vi "Main.vi"() -> ()   [LabVIEW 2024]
uses:
  1. CTL/Brain_Loop_CTL.ctl
  <vilib>/Utility/sysdir.llb/System Directory Type.ctl
  <vilib>/Utility/miscctls.llb/LVPointTypeDef.ctl
panel:
  out "Water_Velocity_2_4":waveform(dbl)(graph)
  out "현재 날짜":string="20"
  out "Averange_Soundspeed_4_5":dbl=7.316387579983064e-08
  out "Averange_Soundspeed_3_5":dbl=2.63750763247972e-07
  out "Averange_Soundspeed_3_4":dbl=7.517605612501092e-08
  out "Averange_Soundspeed_2_5":dbl=3.648976015497772e-07
  out "Averange_Soundspeed_2_4":dbl=2.893826616008644e-07
  out "Averange_Soundspeed_2_3":dbl=7.204154122037209e-07
  out "Averange_Soundspeed_1_5":dbl=6.49097871998956e-08
  out "Averange_Soundspeed_1_4":dbl=1.690561397420498e-07
  out "Averange_Soundspeed_1_3":dbl=1.3254525208911302e-07
  out "Averange_Soundspeed_1_2":dbl=1.8535860648145934e-07
  out "Water_Velocity_4_5":dbl=-0.00010251507677933109
  out "Water_Velocity_3_5":dbl=2.0738097770401804e-05
  out "Water_Velocity_3_4":dbl=-0.00010383942518398899
  out "Water_Velocity_2_5":dbl=-0.01115620755326451
  out "Water_Velocity_2_4":dbl=-0.05349117371632417
  out "Water_Velocity_2_3":dbl=-0.0019132083831803978
  out "Water_Velocity_1_5":dbl=-2.0298889268723733e-05
  out "Water_Velocity_1_4":dbl=0.0007566055432670952
  out "Water_Velocity_1_2":dbl=-0.0005455624048940616
  out "Water_Velocity_1_3":dbl=-0.00019492950449177826
  out "배열":string[](array[string])=["5.120312e-10", "+004.20"]
  out "Averange_Soundspeed_4_5":waveform(dbl)(graph)
  out "Averange_Soundspeed_3_5":waveform(dbl)(graph)
  out "Averange_Soundspeed_3_4":waveform(dbl)(graph)
  out "Averange_Soundspeed_2_5":waveform(dbl)(graph)
  out "Averange_Soundspeed_2_4":waveform(dbl)(graph)
  out "Averange_Soundspeed_2_3":waveform(dbl)(graph)
  out "Averange_Soundspeed_1_5":waveform(dbl)(graph)
  out "Averange_Soundspeed_1_4":waveform(dbl)(graph)
  out "Averange_Soundspeed_1_3":waveform(dbl)(graph)
  out "Averange_Soundspeed_1_2":waveform(dbl)(graph)
  out "Water_Velocity_4_5":waveform(dbl)(graph)
  out "Water_Velocity_3_5":waveform(dbl)(graph)
  out "Water_Velocity_3_4":waveform(dbl)(graph)
  out "Water_Velocity_2_5":waveform(dbl)(graph)
  out "Water_Velocity_2_3":waveform(dbl)(graph)
  out "Water_Velocity_1_5":waveform(dbl)(graph)
  out "Water_Velocity_1_4":waveform(dbl)(graph)
  out "Water_Velocity_1_3":waveform(dbl)(graph)
  out "Water_Velocity_1_2":waveform(dbl)(graph)
  in  "유속 데이터 흐름표_50분":i32(listbox)=-1
  in  "유속 데이터 흐름표_30분":i32(listbox)=-1
  in  "유속 데이터 흐름표_10분":i32(listbox)=-1
  in  "유속 데이터":T1
  in  "데이터 통계":T2
  in  "관리자":T3
  out "디버깅 로그 기록":string="queue2:배터리 전원,소모전류,컨트롤 온도,수온,압력,ROLL,Pitch,2, queue3:(1, 2, 2000, 0, 0, 0, 0, 0, 0, 0, 0, 0, 0, 0, 0, 0, 0, 0, 0, 0, 0, 0, 0, 0, 0, 0, 0, 0, 0, 0, 0, 0, 0, 0, 0, 0, 0, 0, 0, 0, 0, 0, 0, 0, 0, 0, 0, 0, 0, 0, 0, 0, 0, 0, 0, 0, 0, 0, 0, 0, 0, 0, 0, 0, 0, 0, 0, 0, 0, 0, 0, 0, 0, 0, 0, 0, 0, 0, 0, 0, 0, 0, 0, 0, 0, 0, 0, 0, 0, 0, 0, 0, 0, 0, 0, 0, 0, 0, 0, 0, 0, 0, 0, 0, 0, 0, 0, 0, 0, 0, 0, 0, 0, 0, 0, 0, 0, 0, 0, 0, 0, 0, 0, 0, 0, 0, 0, 0, 0, 0, 0, 0, 0, 0, 0, 0, 0, 0, 0, 0, 0, 0, 0, 0, 0, 0, 0, 0, 0, 0, 0, 0, 0, 0, 0, 0, 0, 0, 0, 0, 0, 0, 0, 0, 0, 0, 0, 0, 0, 0, 0, 0, 0, 0, 0, 0, 0, 0, 0, 0, 0, 0, 0, 0, 0, 0, 0, 0, 1, 1, 1, 1, 1, 1, 1, 1, 1, 1, 1, 1, 1, 1, 1, 1, 1, 1, 1, 1, 1, 1, 1, 1, 1, 1, 1, 1, 1, 1, 1, 1, 1, 1, 1, 1, 1, 1, 1, 1, 1, 1, 1, 1, 1, 1, 1, 1, 1, 1, 1, 1, 1, 1, 1, 1, 1, 1, 1, 1, 1, 1, 1, 1, 1, 1, 1, 1, 1, 1, 1, 1, 1, 1, 1, 1, 1, 1, 1, 1, 1, 1, 1, 1, 1, 1, 1, 1, 1, 1, 1, 1, 1, 1, 1, 1, 1, 1, 1, 1, 1, 1, 1, 1, 1, 1, 1, 1, 1, 1, 1, 1, 1, 1, 1, 1, 1, 1, 1, 1, 1, 1, 1, 1, 1, 1, 1, 1, 1, 1, 1, 1, 1, 1, 1, 1, 1, 1, 1, 1, 2, 2, 2, 2, 2, 2, 2, 2, 2, 2, 2, 2, 2, 2, 2, 2, 2, 2, 2, 2, 2, 2, 2, 2, 2, 2, 2, 2, 2, 2, 2, 2, 2, 2, 2, 2, 2, 2, 2, 2, 2, 2, 2, 2, 2, 2, 2, 2, 2, 2, 2, 2, 2, 2, 2, 2, 2, 2, 2, 2, 2, 2, 2, 2, 2, 2, 2, 2, 2, 2, 2, 2, 2, 2, 2, 2, 2, 2, 2, 2, 2, 2, 2, 2, 2, 2, 2, 2, 2, 2, 2, 2, 2, 2, 2, 2, 2, 2, 3, 3, 3, 3, 3, 3, 3, 3, 3, 3, 3, 3, 3, 3, 3, 3, 3, 3, 3, 3, 3, 3, 3, 3, 3, 3, 3, 3, 3, 3, 3, 3, 3, 3, 3, 3, 3, 3, 3, 3, 3, 3, 3, 3, 3, 3, 3, 3, 3, 3, 3, 3, 3, 3, 3, 3, 3, 3, 3, 3, 3, 3, 3, 3, 3, 3, 3, 3, 3, 3, 3, 3, 3, 3, 3, 3, 3, 3, 3, 3, 3, 3, 4, 4, 4, 4, 4, 4, 4, 4, 4, 4, 4, 4, 4, 4, 4, 4, 4, 4, 4, 4, 4, 4, 4, 4, 4, 4, 4, 4, 4, 4, 4, 4, 4, 4, 4, 4, 4, 4, 4, 4, 4, 4, 4, 4, 4, 4, 4, 4, 4, 4, 4, 4, 4, 4, 4, 4, 4, 4, 4, 4, 4, 4, 4, 4, 4, 4, 4, 4, 4, 4, 4, 5, 5, 5, 5, 5, 5, 5, 5, 5, 5, 5, 5, 5, 5, 5, 5, 5, 5, 5, 5, 5, 5, 5, 5, 5, 5, 5, 5, 5, 5, 5, 5, 5, 5, 5, 5, 5, 5, 5, 5, 5, 5, 5, 5, 5, 5, 5, 5, 5, 5, 5, 5, 5, 5, 5, 5, 5, 5, 5, 5, 5, 5, 5, 5, 5, 6, 6, 6, 6, 6, 6, 6, 6, 6, 6, 6, 6, 6, 6, 6, 6, 6, 6, 6, 6, 6, 6, 6, 6, 6, 6, 6, 6, 6, 6, 6, 6, 6, 6, 6, 6, 6, 6, 6, 6, 6, 6, 6, 6, 6, 6, 6, 6, 6, 6, 6, 6, 6, 6, 6, 6, 6, 6, 6, 7, 7, 7, 7, 7, 7, 7, 7, 7, 7, 7, 7, 7, 7, 7, 7, 7, 7, 7, 7, 7, 7, 7, 7, 7, 7, 7, 7, 7, 7, 7, 7, 7, 7, 7, 7, 7, 7, 7, 7, 7, 7, 7, 7, 7, 7, 7, 7, 7, 7, 7, 7, 7, 7, 7, 7, 8, 8, 8, 8, 8, 8, 8, 8, 8, 8, 8, 8, 8, 8, 8, 8, 8, 8, 8, 8, 8, 8, 8, 8, 8, 8, 8, 8, 8, 8, 8, 8, 8, 8, 8, 8, 8, 8, 8, 8, 8, 8, 8, 8, 8, 8, 8, 8, 8, 8, 8, 8, 8, 9, 9, 9, 9, 9, 9, 9, 9, 9, 9, 9, 9, 9, 9, 9, 9, 9, 9, 9, 9, 9, 9, 9, 9, 9, 9, 9, 9, 9, 9, 9, 9, 9, 9, 9, 9, 9, 9, 9, 9, 9, 9, 9, 9, 9, 9, 9, 9, 9, 9, 9, 10, 10, 10, 10, 10, 10, 10, 10, 10, 10, 10, 10, 10, 10, 10, 10, 10, 10, 10, 10, 10, 10, 10, 10, 10, 10, 10, 10, 10, 10, 10, 10, 10, 10, 10, 10, 10, 10, 10, 10, 10, 10, 10, 10, 10, 10, 10, 10, 11, 11, 11, 11, 11, 11, 11, 11, 11, 11, 11, 11, 11, 11, 11, 11, 11, 11, 11, 11, 11, 11, 11, 11, 11, 11, 11, 11, 11, 11, 11, 11, 11, 11, 11, 11, 11, 11, 11, 11, 11, 11, 11, 11, 11, 11, 11, 12, 12, 12, 12, 12, 12, 12, 12, 12, 12, 12, 12, 12, 12, 12, 12, 12, 12, 12, 12, 12, 12, 12, 12, 12, 12, 12, 12, 12, 12, 12, 12, 12, 12, 12, 12, 12, 12, 12, 12, 12, 12, 12, 12, 12, 13, 13, 13, 13, 13, 13, 13, 13, 13, 13, 13, 13, 13, 13, 13, 13, 13, 13, 13, 13, 13, 13, 13, 13, 13, 13, 13, 13, 13, 13, 13, 13, 13, 13, 13, 13, 13, 13, 13, 13, 13, 13, 13, 13, 14, 14, 14, 14, 14, 14, 14, 14, 14, 14, 14, 14, 14, 14, 14, 14, 14, 14, 14, 14, 14, 14, 14, 14, 14, 14, 14, 14, 14, 14, 14, 14, 14, 14, 14, 14, 14, 14, 14, 14, 14, 14, 15, 15, 15, 15, 15, 15, 15, 15, 15, 15, 15, 15, 15, 15, 15, 15, 15, 15, 15, 15, 15, 15, 15, 15, 15, 15, 15, 15, 15, 15, 15, 15, 15, 15, 15, 15, 15, 15, 15, 15, 15, 15, 16, 16, 16, 16, 16, 16, 16, 16, 16, 16, 16, 16, 16, 16, 16, 16, 16, 16, 16, 16, 16, 16, 16, 16, 16, 16, 16, 16, 16, 16, 16, 16, 16, 16, 16, 16, 16, 16, 16, 16, 16, 17, 17, 17, 17, 17, 17, 17, 17, 17, 17, 17, 17, 17, 17, 17, 17, 17, 17, 17, 17, 17, 17, 17, 17, 17, 17, 17, 17, 17, 17, 17, 17, 17, 17, 17, 17, 17, 17, 17, 17, 18, 18, 18, 18, 18, 18, 18, 18, 18, 18, 18, 18, 18, 18, 18, 18, 18, 18, 18, 18, 18, 18, 18, 18, 18, 18, 18, 18, 18, 18, 18, 18, 18, 18, 18, 18, 18, 18, 18, 19, 19, 19, 19, 19, 19, 19, 19, 19, 19, 19, 19, 19, 19, 19, 19, 19, 19, 19, 19, 19, 19, 19, 19, 19, 19, 19, 19, 19, 19, 19, 19, 19, 19, 19, 19, 19, 19, 20, 20, 20, 20, 20, 20, 20, 20, 20, 20, 20, 20, 20, 20, 20, 20, 20, 20, 20, 20, 20, 20, 20, 20, 20, 20, 20, 20, 20, 20, 20, 20, 20, 20, 20, 20, 20, 20, 21, 21, 21, 21, 21, 21, 21, 21, 21, 21, 21, 21, 21, 21, 21, 21, 21, 21, 21, 21, 21, 21, 21, 21, 21, 21, 21, 21, 21, 21, 21, 21, 21, 21, 21, 21, 21, 21, 22, 22, 22, 22, 22, 22, 22, 22, 22, 22, 22, 22, 22, 22, 22, 22, 22, 22, 22, 22, 22, 22, 22, 22, 22, 22, 22, 22, 22, 22, 22, 22, 22, 22, 22, 22, 23, 23, 23, 23, 23, 23, 23, 23, 23, 23, 23, 23, 23, 23, 23, 23, 23, 23, 23, 23, 23, 23, 23, 23, 23, 23, 23, 23, 23, 23, 23, 23, 23, 23, 23, 23, 23, 24, 24, 24, 24, 24, 24, 24, 24, 24, 24, 24, 24, 24, 24, 24, 24, 24, 24, 24, 24, 24, 24, 24, 24, 24, 24, 24, 24, 24, 24, 24, 24, 24, 24, 24, 24, 25, 25, 25, 25, 25, 25, 25, 25, 25, 25, 25, 25, 25, 25, 25, 25, 25, 25, 25, 25, 25, 25, 25, 25, 25, 25, 25, 25, 25, 25, 25, 25, 25, 25, 25, 25, 26, 26, 26, 26, 26, 26, 26, 26, 26, 26, 26, 26, 26, 26, 26, 26, 26, 26, 26, 26, 26, 26, 26, 26, 26, 26, 26, 26, 26, 26, 26, 26, 26, 26, 26, 27, 27, 27, 27, 27, 27, 27, 27, 27, 27, 27, 27, 27, 27, 27, 27, 27, 27, 27, 27, 27, 27, 27, 27, 27, 27, 27, 27, 27, 27, 27, 27, 27, 27, 27, 28, 28, 28, 28, 28, 28, 28, 28, 28, 28, 28, 28, 28, 28, 28, 28, 28, 28, 28, 28, 28, 28, 28, 28, 28, 28, 28, 28, 28, 28, 28, 28, 28, 28, 28, 29, 29, 29, 29, 29, 29, 29, 29, 29, 29, 29, 29, 29, 29, 29, 29, 29, 29, 29, 29, 29, 29, 29, 29, 29, 29, 29, 29, 29, 29, 29, 29, 29, 29, 30, 30, 30, 30, 30, 30, 30, 30, 30, 30, 30, 30, 30, 30, 30, 30, 30, 30, 30, 30, 30, 30, 30, 30, 30, 30, 30, 30, 30, 30, 30, 30, 30, 30, 31, 31, 31, 31, 31, 31, 31, 31, 31, 31, 31, 31, 31, 31, 31, 31, 31, 31, 31, 31, 31, 31, 31, 31, 31, 31, 31, 31, 31, 31, 31, 31, 31, 31, 31, 32, 32, 32, 32, 32, 32, 32, 32, 32, 32, 32, 32, 32, 32, 32, 32, 32, 32, 32, 32, 32, 32, 32, 32, 32, 32, 32, 32, 32, 32, 32, 32, 32, 33, 33, 33, 33, 33, 33, 33, 33, 33, 33, 33, 33, 33, 33, 33, 33, 33, 33, 33, 33, 33, 33, 33, 33, 33, 33, 33, 33, 33, 33, 33, 33, 33, 33, 34, 34, 34, 34, 34, 34, 34, 34, 34, 34, 34, 34, 34, 34, 34, 34, 34, 34, 34, 34, 34, 34, 34, 34, 34, 34, 34, 34, 34, 34, 34, 34, 34, 34, 35, 35, 35, 35, 35, 35, 35, 35, 35, 35, 35, 35, 35, 35, 35, 35, 35, 35, 35, 35, 35, 35, 35, 35, 35, 35, 35, 35, 35, 35, 35, 35, 35, 36, 36, 36, 36, 36, 36, 36, 36, 36, 36, 36, 36, 36, 36, 36, 36, 36, 36, 36, 36, 36, 36, 36, 36, 36, 36, 36, 36, 36, 36, 36, 36, 36, 36, 37, 37, 37, 37, 37, 37, 37, 37, 37, 37, 37, 37, 37, 37, 37, 37, 37, 37, 37, 37, 37, 37, 37, 37, 37, 37, 37, 37, 37, 37, 37, 37, 37, 38, 38, 38, 38, 38, 38, 38, 38, 38, 38, 38, 38, 38, 38, 38, 38, 38, 38, 38, 38, 38, 38, 38, 38, 38, 38, 38, 38, 38, 38, 38, 38, 38, 38, 39, 39, 39, 39, 39, 39, 39, 39, 39, 39, 39, 39, 39, 39, 39, 39, 39, 39, 39, 39, 39, 39, 39, 39, 39, 39, 39, 39, 39, 39, 39, 39, 39, 40, 40, 40, 40, 40, 40, 40, 40, 40, 40, 40, 40, 40, 40, 40, 40, 40, 40, 40, 40, 40, 40, 40, 40, 40, 40, 40, 40, 40, 40, 40, 40, 40, 40, 40, 39, 39, 39, 39, 39, 39, 39, 39, 39, 39, 39, 39, 39, 39, 39, 39, 39, 39, 39, 39, 39, 39, 39, 39, 39, 39, 39, 39, 39, 39, 39, 39, 39, 38, 38, 38, 38, 38, 38, 38, 38, 38, 38, 38, 38, 38, 38, 38, 38, 38, 38, 38, 38, 38, 38, 38, 38, 38, 38, 38, 38, 38, 38, 38, 38, 38, 38, 37, 37, 37, 37, 37, 37, 37, 37, 37, 37, 37, 37, 37, 37, 37, 37, 37, 37, 37, 37, 37, 37, 37, 37, 37, 37, 37, 37, 37, 37, 37, 37, 37, 36, 36, 36, 36, 36, 36, 36, 36, 36, 36, 36, 36, 36, 36, 36, 36, 36, 36, 36, 36, 36, 36, 36, 36, 36, 36, 36, 36, 36, 36, 36, 36, 36, 36, 35, 35, 35, 35, 35, 35, 35, 35, 35, 35, 35, 35, 35, 35, 35, 35, 35, 35, 35, 35, 35, 35, 35, 35, 35, 35, 35, 35, 35, 35, 35, 35, 35, 34, 34, 34, 34, 34, 34, 34, 34, 34, 34, 34, 34, 34, 34, 34, 34, 34, 34, 34, 34, 34, 34, 34, 34, 34, 34, 34, 34, 34, 34, 34, 34, 34, 34, 33, 33, 33, 33, 33, 33, 33, 33, 33, 33, 33, 33, 33, 33, 33, 33, 33, 33, 33, 33, 33, 33, 33, 33, 33, 33, 33, 33, 33, 33, 33, 33, 33, 33, 32, 32, 32, 32, 32, 32, 32, 32, 32, 32, 32, 32, 32, 32, 32, 32, 32, 32, 32, 32, 32, 32, 32, 32, 32, 32, 32, 32, 32, 32, 32, 32, 32, 31, 31, 31, 31, 31, 31, 31, 31, 31, 31, 31, 31, 31, 31, 31, 31, 31, 31, 31, 31, 31, 31, 31, 31, 31, 31, 31, 31, 31, 31, 31, 31, 31, 31, 31, 30, 30, 30, 30, 30, 30, 30, 30, 30, 30, 30, 30, 30, 30, 30, 30, 30, 30, 30, 30, 30, 30, 30, 30, 30, 30, 30, 30, 30, 30, 30, 30, 30, 30, 29, 29, 29, 29, 29, 29, 29, 29, 29, 29, 29, 29, 29, 29, 29, 29, 29, 29, 29, 29, 29, 29, 29, 29, 29, 29, 29, 29, 29, 29, 29, 29, 29, 29, 28, 28, 28, 28, 28, 28, 28, 28, 28, 28, 28, 28, 28, 28, 28, 28, 28, 28, 28, 28, 28, 28, 28, 28, 28, 28, 28, 28, 28, 28, 28, 28, 28, 28, 28, 27, 27, 27, 27, 27, 27, 27, 27, 27, 27, 27, 27, 27, 27, 27, 27, 27, 27, 27, 27, 27, 27, 27, 27, 27, 27, 27, 27, 27, 27, 27, 27, 27, 27, 27, 26, 26, 26, 26, 26, 26, 26, 26, 26, 26, 26, 26, 26, 26, 26, 26, 26, 26, 26, 26, 26, 26, 26, 26, 26, 26, 26, 26, 26, 26, 26, 26, 26, 26, 26, 25, 25, 25, 25, 25, 25, 25, 25, 25, 25, 25, 25, 25, 25, 25, 25, 25, 25, 25, 25, 25, 25, 25, 25, 25, 25, 25, 25, 25, 25, 25, 25, 25, 25, 25, 25, 24, 24, 24, 24, 24, 24, 24, 24, 24, 24, 24, 24, 24, 24, 24, 24, 24, 24, 24, 24, 24, 24, 24, 24, 24, 24, 24, 24, 24, 24, 24, 24, 24, 24, 24, 24, 23, 23, 23, 23, 23, 23, 23, 23, 23, 23, 23, 23, 23, 23, 23, 23, 23, 23, 23, 23, 23, 23, 23, 23, 23, 23, 23, 23, 23, 23, 23, 23, 23, 23, 23, 23, 23, 22, 22, 22, 22, 22, 22, 22, 22, 22, 22, 22, 22, 22, 22, 22, 22, 22, 22, 22, 22, 22, 22, 22, 22, 22, 22, 22, 22, 22, 22, 22, 22, 22, 22, 22, 22, 21, 21, 21, 21, 21, 21, 21, 21, 21, 21, 21, 21, 21, 21, 21, 21, 21, 21, 21, 21, 21, 21, 21, 21, 21, 21, 21, 21, 21, 21, 21, 21, 21, 21, 21, 21, 21, 21, 20, 20, 20, 20, 20, 20, 20, 20, 20, 20, 20, 20, 20, 20, 20, 20, 20, 20, 20, 20, 20, 20, 20, 20, 20, 20, 20, 20, 20, 20, 20, 20, 20, 20, 20, 20, 20, 20, 19, 19, 19, 19, 19, 19, 19, 19, 19, 19, 19, 19, 19, 19, 19, 19, 19, 19, 19, 19, 19, 19, 19, 19, 19, 19, 19, 19, 19, 19, 19, 19, 19, 19, 19, 19, 19, 19, 18, 18, 18, 18, 18, 18, 18, 18, 18, 18, 18, 18, 18, 18, 18, 18, 18, 18, 18, 18, 18, 18, 18, 18, 18, 18, 18, 18, 18, 18, 18, 18, 18, 18, 18, 18, 18, 18, 18, 17, 17, 17, 17, 17, 17, 17, 17, 17, 17, 17, 17, 17, 17, 17, 17, 17, 17, 17, 17, 17, 17, 17, 17, 17, 17, 17, 17, 17, 17, 17, 17, 17, 17, 17, 17, 17, 17, 17, 17, 16, 16, 16, 16, 16, 16, 16, 16, 16, 16, 16, 16, 16, 16, 16, 16, 16, 16, 16, 16, 16, 16, 16, 16, 16, 16, 16, 16, 16, 16, 16, 16, 16, 16, 16, 16, 16, 16, 16, 16, 16, 15, 15, 15, 15, 15, 15, 15, 15, 15, 15, 15, 15, 15, 15, 15, 15, 15, 15, 15, 15, 15, 15, 15, 15, 15, 15, 15, 15, 15, 15, 15, 15, 15, 15, 15, 15, 15, 15, 15, 15, 15, 15, 14, 14, 14, 14, 14, 14, 14, 14, 14, 14, 14, 14, 14, 14, 14, 14, 14, 14, 14, 14, 14, 14, 14, 14, 14, 14, 14, 14, 14, 14, 14, 14, 14, 14, 14, 14, 14, 14, 14, 14, 14, 14, 13, 13, 13, 13, 13, 13, 13, 13, 13, 13, 13, 13, 13, 13, 13, 13, 13, 13, 13, 13, 13, 13, 13, 13, 13, 13, 13, 13, 13, 13, 13, 13, 13, 13, 13, 13, 13, 13, 13, 13, 13, 13, 13, 13, 12, 12, 12, 12, 12, 12, 12, 12, 12, 12, 12, 12, 12, 12, 12, 12, 12, 12, 12, 12, 12, 12, 12, 12, 12, 12, 12, 12, 12, 12, 12, 12, 12, 12, 12, 12, 12, 12, 12, 12, 12, 12, 12, 12, 12, 11, 11, 11, 11, 11, 11, 11, 11, 11, 11, 11, 11, 11, 11, 11, 11, 11, 11, 11, 11, 11, 11, 11, 11, 11, 11, 11, 11, 11, 11, 11, 11, 11, 11, 11, 11, 11, 11, 11, 11, 11, 11, 11, 11, 11, 11, 11, 10, 10, 10, 10, 10, 10, 10, 10, 10, 10, 10, 10, 10, 10, 10, 10, 10, 10, 10, 10, 10, 10, 10, 10, 10, 10, 10, 10, 10, 10, 10, 10, 10, 10, 10, 10, 10, 10, 10, 10, 10, 10, 10, 10, 10, 10, 10, 10, 9, 9, 9, 9, 9, 9, 9, 9, 9, 9, 9, 9, 9, 9, 9, 9, 9, 9, 9, 9, 9, 9, 9, 9, 9, 9, 9, 9, 9, 9, 9, 9, 9, 9, 9, 9, 9, 9, 9, 9, 9, 9, 9, 9, 9, 9, 9, 9, 9, 9, 9, 8, 8, 8, 8, 8, 8, 8, 8, 8, 8, 8, 8, 8, 8, 8, 8, 8, 8, 8, 8, 8, 8, 8, 8, 8, 8, 8, 8, 8, 8, 8, 8, 8, 8, 8, 8, 8, 8, 8, 8, 8, 8, 8, 8, 8, 8, 8, 8, 8, 8, 8, 8, 8, 7, 7, 7, 7, 7, 7, 7, 7, 7, 7, 7, 7, 7, 7, 7, 7, 7, 7, 7, 7, 7, 7, 7, 7, 7, 7, 7, 7, 7, 7, 7, 7, 7, 7, 7, 7, 7, 7, 7, 7, 7, 7, 7, 7, 7, 7, 7, 7, 7, 7, 7, 7, 7, 7, 7, 7, 6, 6, 6, 6, 6, 6, 6, 6, 6, 6, 6, 6, 6, 6, 6, 6, 6, 6, 6, 6, 6, 6, 6, 6, 6, 6, 6, 6, 6, 6, 6, 6, 6, 6, 6, 6, 6, 6, 6, 6, 6, 6, 6, 6, 6, 6, 6, 6, 6, 6, 6, 6, 6, 6, 6, 6, 6, 6, 6, 5, 5, 5, 5, 5, 5, 5, 5, 5, 5, 5, 5, 5, 5, 5, 5, 5, 5, 5, 5, 5, 5, 5, 5, 5, 5, 5, 5, 5, 5, 5, 5, 5, 5, 5, 5, 5, 5, 5, 5, 5, 5, 5, 5, 5, 5, 5, 5, 5, 5, 5, 5, 5, 5, 5, 5, 5, 5, 5, 5, 5, 5, 5, 5, 5, 4, 4, 4, 4, 4, 4, 4, 4, 4, 4, 4, 4, 4, 4, 4, 4, 4, 4, 4, 4, 4, 4, 4, 4, 4, 4, 4, 4, 4, 4, 4, 4, 4, 4, 4, 4, 4, 4, 4, 4, 4, 4, 4, 4, 4, 4, 4, 4, 4, 4, 4, 4, 4, 4, 4, 4, 4, 4, 4, 4, 4, 4, 4, 4, 4, 4, 4, 4, 4, 4, 4, 3, 3, 3, 3, 3, 3, 3, 3, 3, 3, 3, 3, 3, 3, 3, 3, 3, 3, 3, 3, 3, 3, 3, 3, 3, 3, 3, 3, 3, 3, 3, 3, 3, 3, 3, 3, 3, 3, 3, 3, 3, 3, 3, 3, 3, 3, 3, 3, 3, 3, 3, 3, 3, 3, 3, 3, 3, 3, 3, 3, 3, 3, 3, 3, 3, 3, 3, 3, 3, 3, 3, 3, 3, 3, 3, 3, 3, 3, 3, 3, 3, 3, 2, 2, 2, 2, 2, 2, 2, 2, 2, 2, 2, 2, 2, 2, 2, 2, 2, 2, 2, 2, 2, 2, 2, 2, 2, 2, 2, 2, 2, 2, 2, 2, 2, 2, 2, 2, 2, 2, 2, 2, 2, 2, 2, 2, 2, 2, 2, 2, 2, 2, 2, 2, 2, 2, 2, 2, 2, 2, 2, 2, 2, 2, 2, 2, 2, 2, 2, 2, 2, 2, 2, 2, 2, 2, 2, 2, 2, 2, 2, 2, 2, 2, 2, 2, 2, 2, 2, 2, 2, 2, 2, 2, 2, 2, 2, 2, 2, 2, 1, 1, 1, 1, 1, 1, 1, 1, 1, 1, 1, 1, 1, 1, 1, 1, 1, 1, 1, 1, 1, 1, 1, 1, 1, 1, 1, 1, 1, 1, 1, 1, 1, 1, 1, 1, 1, 1, 1, 1, 1, 1, 1, 1, 1, 1, 1, 1, 1, 1, 1, 1, 1, 1, 1, 1, 1, 1, 1, 1, 1, 1, 1, 1, 1, 1, 1, 1, 1, 1, 1, 1, 1, 1, 1, 1, 1, 1, 1, 1, 1, 1, 1, 1, 1, 1, 1, 1, 1, 1, 1, 1, 1, 1, 1, 1, 1, 1, 1, 1, 1, 1, 1, 1, 1, 1, 1, 1, 1, 1, 1, 1, 1, 1, 1, 1, 1, 1, 1, 1, 1, 1, 1, 1, 1, 1, 1, 1, 1, 1, 1, 1, 1, 1, 1, 1, 1, 1, 1, 1, 0, 0, 0, 0, 0, 0, 0, 0, 0, 0, 0, 0, 0, 0, 0, 0, 0, 0, 0, 0, 0, 0, 0, 0, 0, 0, 0, 0, 0, 0, 0, 0, 0, 0, 0, 0, 0, 0, 0, 0, 0, 0, 0, 0, 0, 0, 0, 0, 0, 0, 0, 0, 0, 0, 0, 0, 0, 0, 0, 0, 0, 0, 0, 0, 0, 0, 0, 0, 0, 0, 0, 0, 0, 0, 0, 0, 0, 0, 0, 0, 0, 0, 0, 0, 0, 0, 0, 0, 0, 0, 0, 0, 0, 0, 0, 0, 0, 0, 0, 0, 0, 0, 0, 0, 0, 0, 0, 0, 0, 0, 0, 0, 0, 0, 0, 0, 0, 0, 0, 0, 0, 0, 0, 0, 0, 0, 0, 0, 0, 0, 0, 0, 0, 0, 0, 0, 0, 0, 0, 0, 0, 0, 0, 0, 0, 0, 0, 0, 0, 0, 0, 0, 0, 0, 0, 0, 0, 0, 0, 0, 0, 0, 0, 0, 0, 0, 0, 0, 0, 0, 0, 0, 0, 0, 0, 0, 0, 0, 0, 0, 0, 0, 0, 0, 0), queue4:1PPS,37.4172384,127.1338756,2"
  in  "전체메뉴_탭_컨트롤":enum32{"지도", "데이터 통계", "관리자", "유속 데이터"}(tab)=enum."관리자"
  out "Station_5_수신시작시간":string
  out "Station_4_수신시작시간":string
  out "Station_3_수신시작시간":string
  out "Station_2_수신시작시간":string
  out "Station_1_수신시작시간":string
  out "Station_5":cluster{dbl[], i32[]}(graph)
  out "TX_LED_5":bool
  out "RX_LED_5":bool
  out "Station_4":cluster{dbl[], i32[]}(graph)
  out "TX_LED_4":bool
  out "RX_LED_4":bool
  out "Station_3":cluster{dbl[], i32[]}(graph)
  out "TX_LED_3":bool
  out "RX_LED_3":bool
  out "Station_2":cluster{dbl[], i32[]}(graph)
  out "TX_LED_2":bool
  out "RX_LED_2":bool
  out "Station_1":cluster{dbl[], i32[]}(graph)
  out "TX_LED_1":bool
  out "RX_LED_1":bool
  in  "관리자_내부_탭_컨트롤":enum32{"실시간 현황", "Setting"}(tab) caption="탭 컨트롤 2"
  out "Station_현황_GPS":i32[](listbox)
  out "데이터 통계 현황_결과창":string
  out "Station_현황_TRX_Controller":i32[](listbox)
  in  "SET 버튼":bool
  in  "Python 경로":path=path "D:/Python39-32/python.exe"
  out "적용_LED":bool
  in  "적용 버튼":bool
  in  "정지":bool
  in  "Publish_모듈 경로":path=path "C:/Users/kjsiot/Desktop/CATS_V4.0/5. Python/Mqtt_Publish_Client.py"
  in  "Subscribe_모듈 경로":path=path "C:/Users/kjsiot/Desktop/CATS_V4.0/5. Python/Mqtt_Subscribe_Client.py"
  in  "지도 모듈 경로":path=path "C:/Users/kjsiot/Desktop/CATS_V4.0/5. Python/Generate_map.py"
  out "적용_LED 2":bool
  in  "Wake_UP버튼":bool
  out "지도모듈_LED":bool
  in  "지도":T4
  in  "Order":i32=12
  in  "Q 값":i32=4
  # "데이터 통계 현황"
  # "Costal Acoustic Tomography Setting"
  # "Data_path"
  # "Coastal_TMC_Set_Variable"
  # "Coastal_TMC_Map_Web"
  # "Sation_Wake_UP"
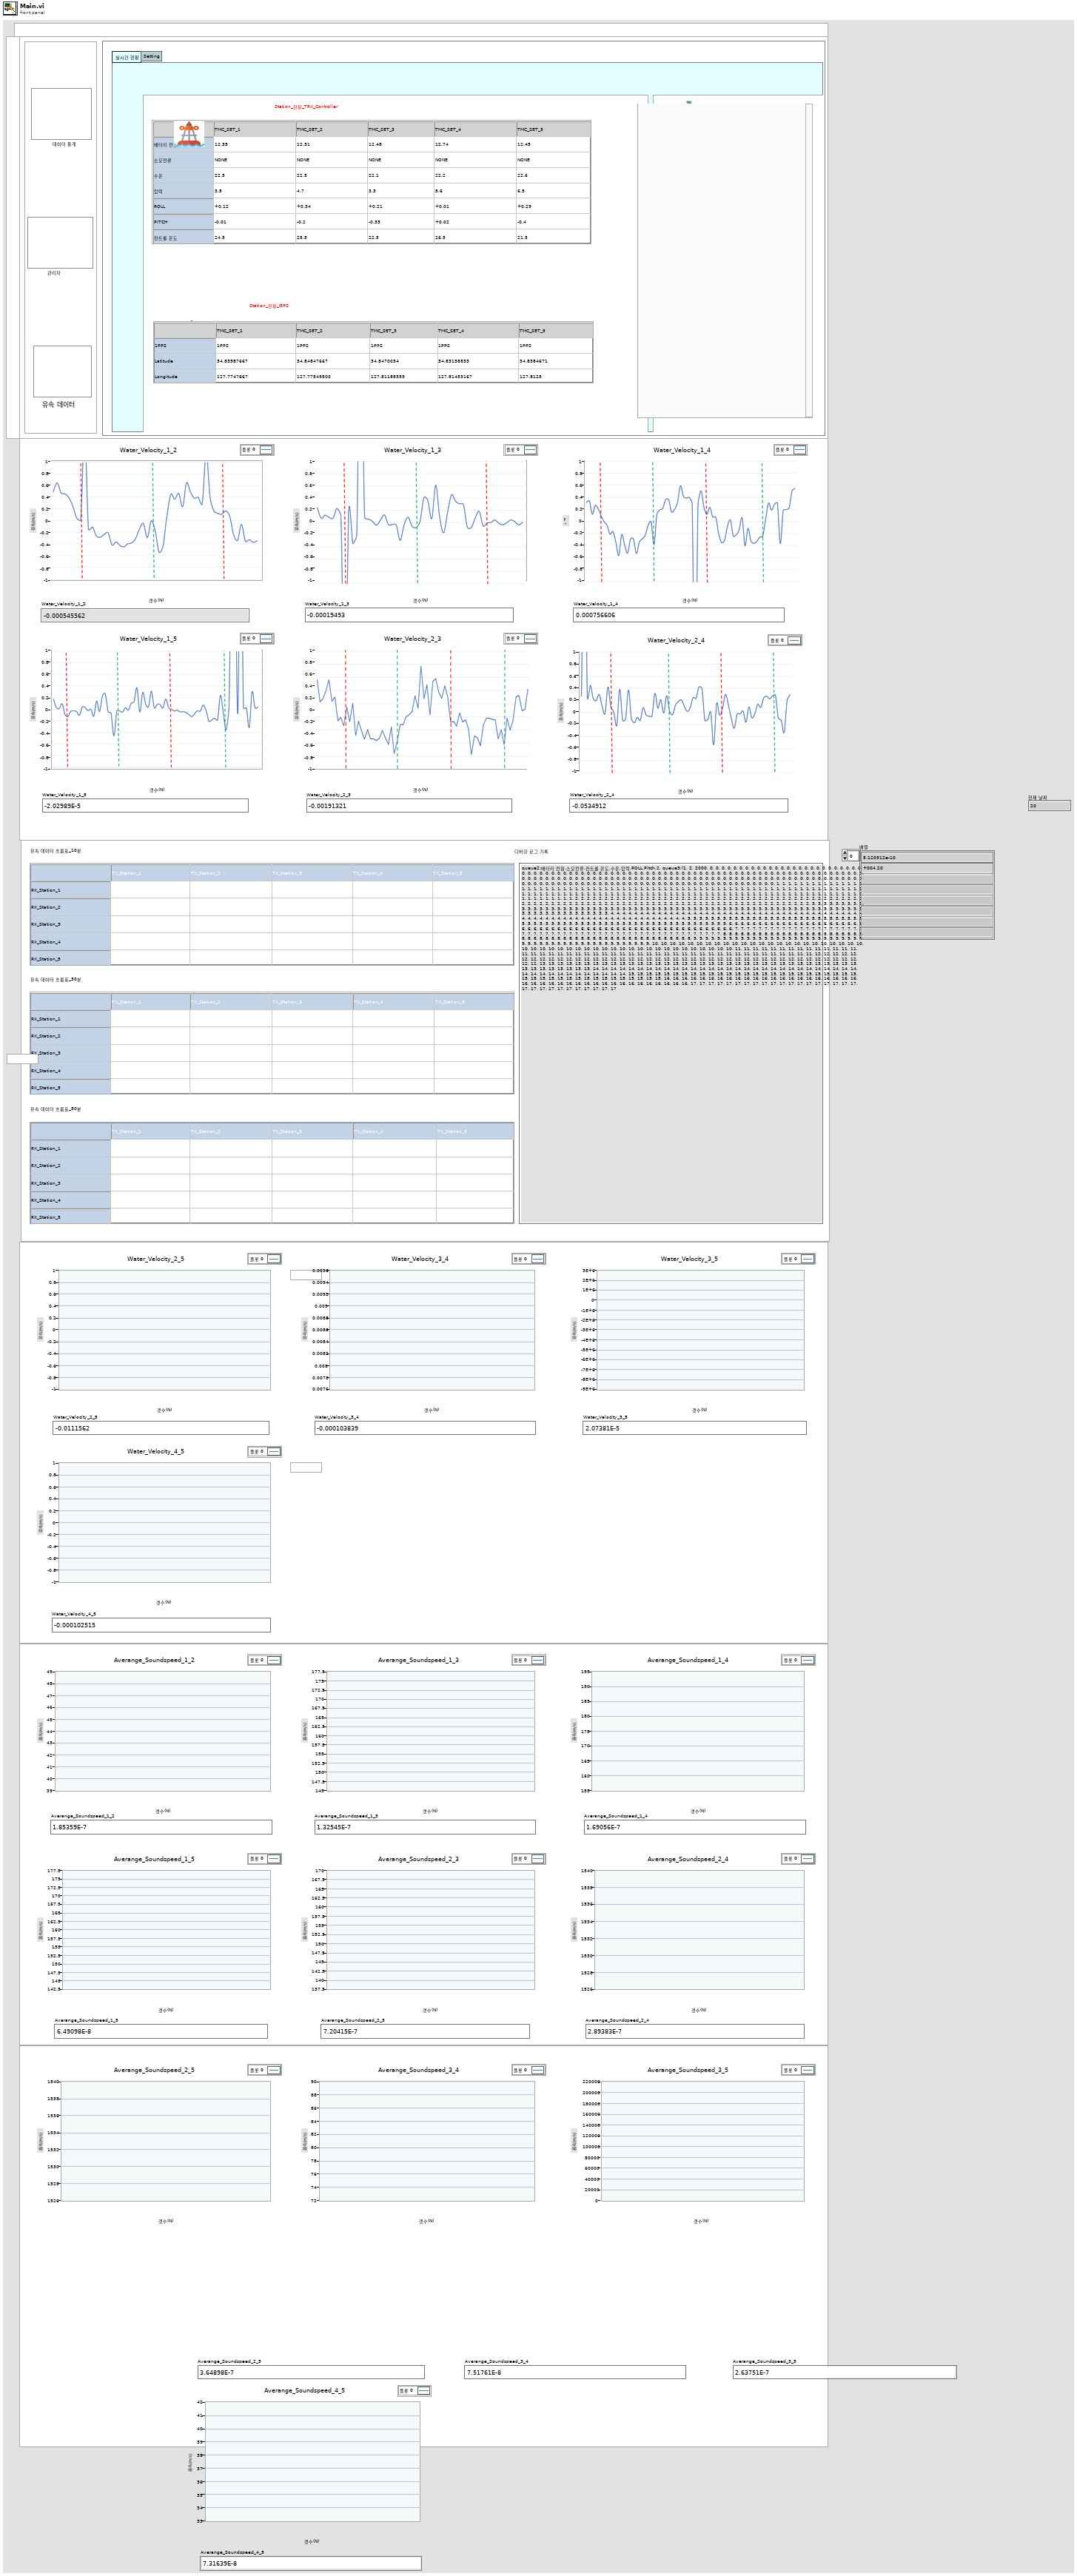
[diagram p1: front panel]
types:
  T1 = typedef "알림 컨트롤.ctl" = bool
  T2 = typedef "데이터 컨트롤.ctl" = bool
  T3 = typedef "관리 컨트롤.ctl" = bool
  T4 = typedef "지도 컨트롤.ctl" = bool
  T5 = cluster{"Water_Velocity_1_3":dbl, "Water_Velocity_1_2":dbl, "Water_Velocity_1_4":dbl, "Water_Velocity_1_5":dbl, "Water_Velocity_2_3":dbl, "Water_Velocity_2_4":dbl, "Water_Velocity_2_5":dbl, "Water_Velocity_3_4":dbl, "Water_Velocity_3_5":dbl, "Water_Velocity_4_5":dbl, "Averange_Soundspeed_1_2":dbl, "Averange_Soundspeed_1_3":dbl, "Averange_Soundspeed_1_4":dbl, "Averange_Soundspeed_1_5":dbl, "Averange_Soundspeed_2_3":dbl, "Averange_Soundspeed_2_4":dbl, "Averange_Soundspeed_2_5":dbl, "Averange_Soundspeed_3_4":dbl, "Averange_Soundspeed_3_5":dbl, "Averange_Soundspeed_4_5":dbl}
  T6 = cluster{"로그기록":string, "RX_그래프_LED":bool, "RX_그래프2_LED":bool, "RX_그래프3_LED":bool, "RX_그래프4_LED":bool, "RX_그래프5_LED":bool}
  T7 = cluster{"TX_그래프_LED":bool, "TX_그래프2_LED":bool, "TX_그래프3_LED":bool, "TX_그래프4_LED":bool, "TX_그래프5_LED":bool, "유속데이터흐름표_10분":string[][], "유속데이터흐름표_30분":string[][], "유속데이터흐름표_50분":string[][]}
  T8 = cluster{"Python 경로":path, "Publish 모듈 경로":path, "지도 모듈 경로":path, "Subscribe 모듈 경로":path}
  T9 = typedef "Brain_Loop_CTL.ctl" = enum16{"초기화", "Mqtt_Subscribe", "Mqtt_Publish", "지도", "관리자", "데이터통계", "유속 데이터", "정지", "Mqtt_Publish_2"}
  T10 = typedef "System Directory Type.ctl" = i32
  T11 = typedef "LVPointTypeDef.ctl" = cluster{"Horizontal":i16, "Vertical":i16}
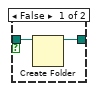
[diagram p2: hidden frame]
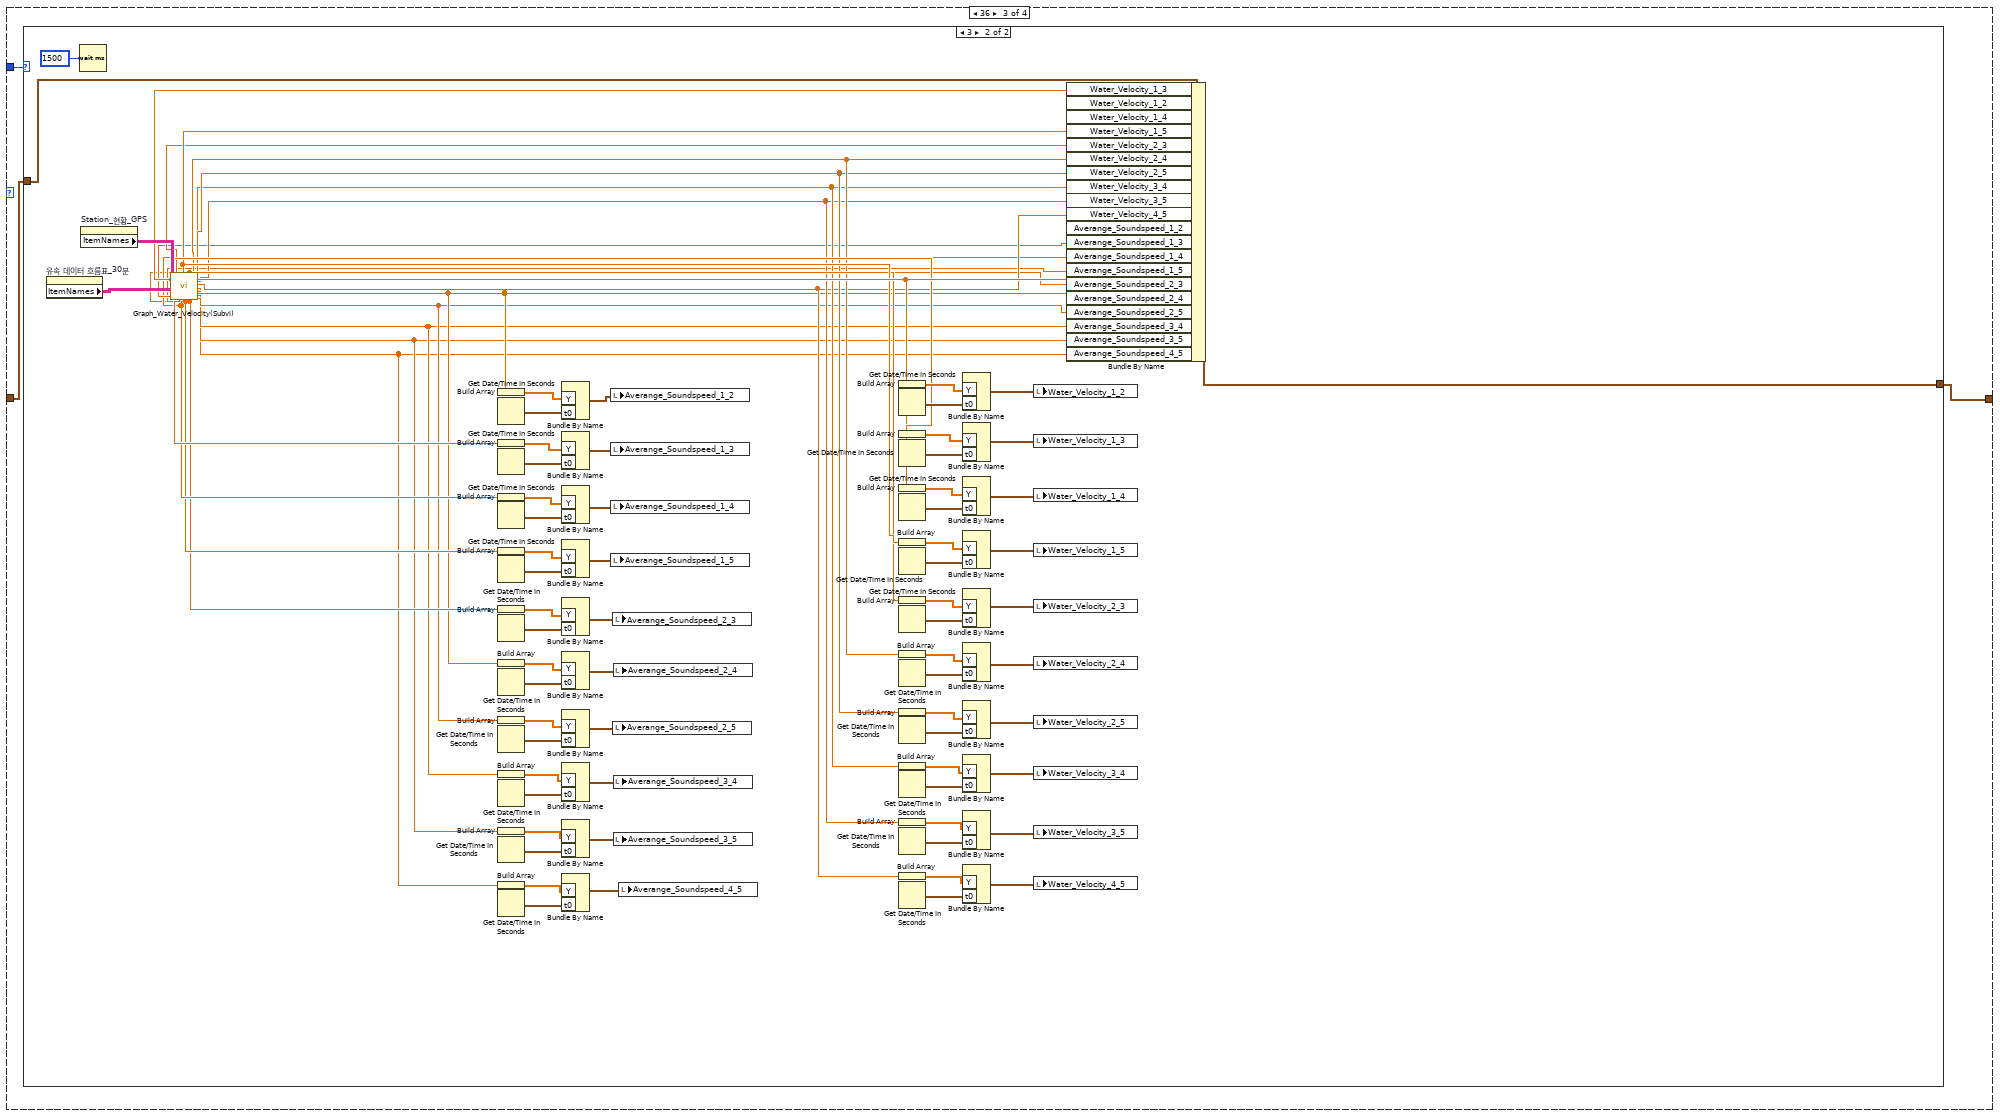
[diagram p6: hidden frame]
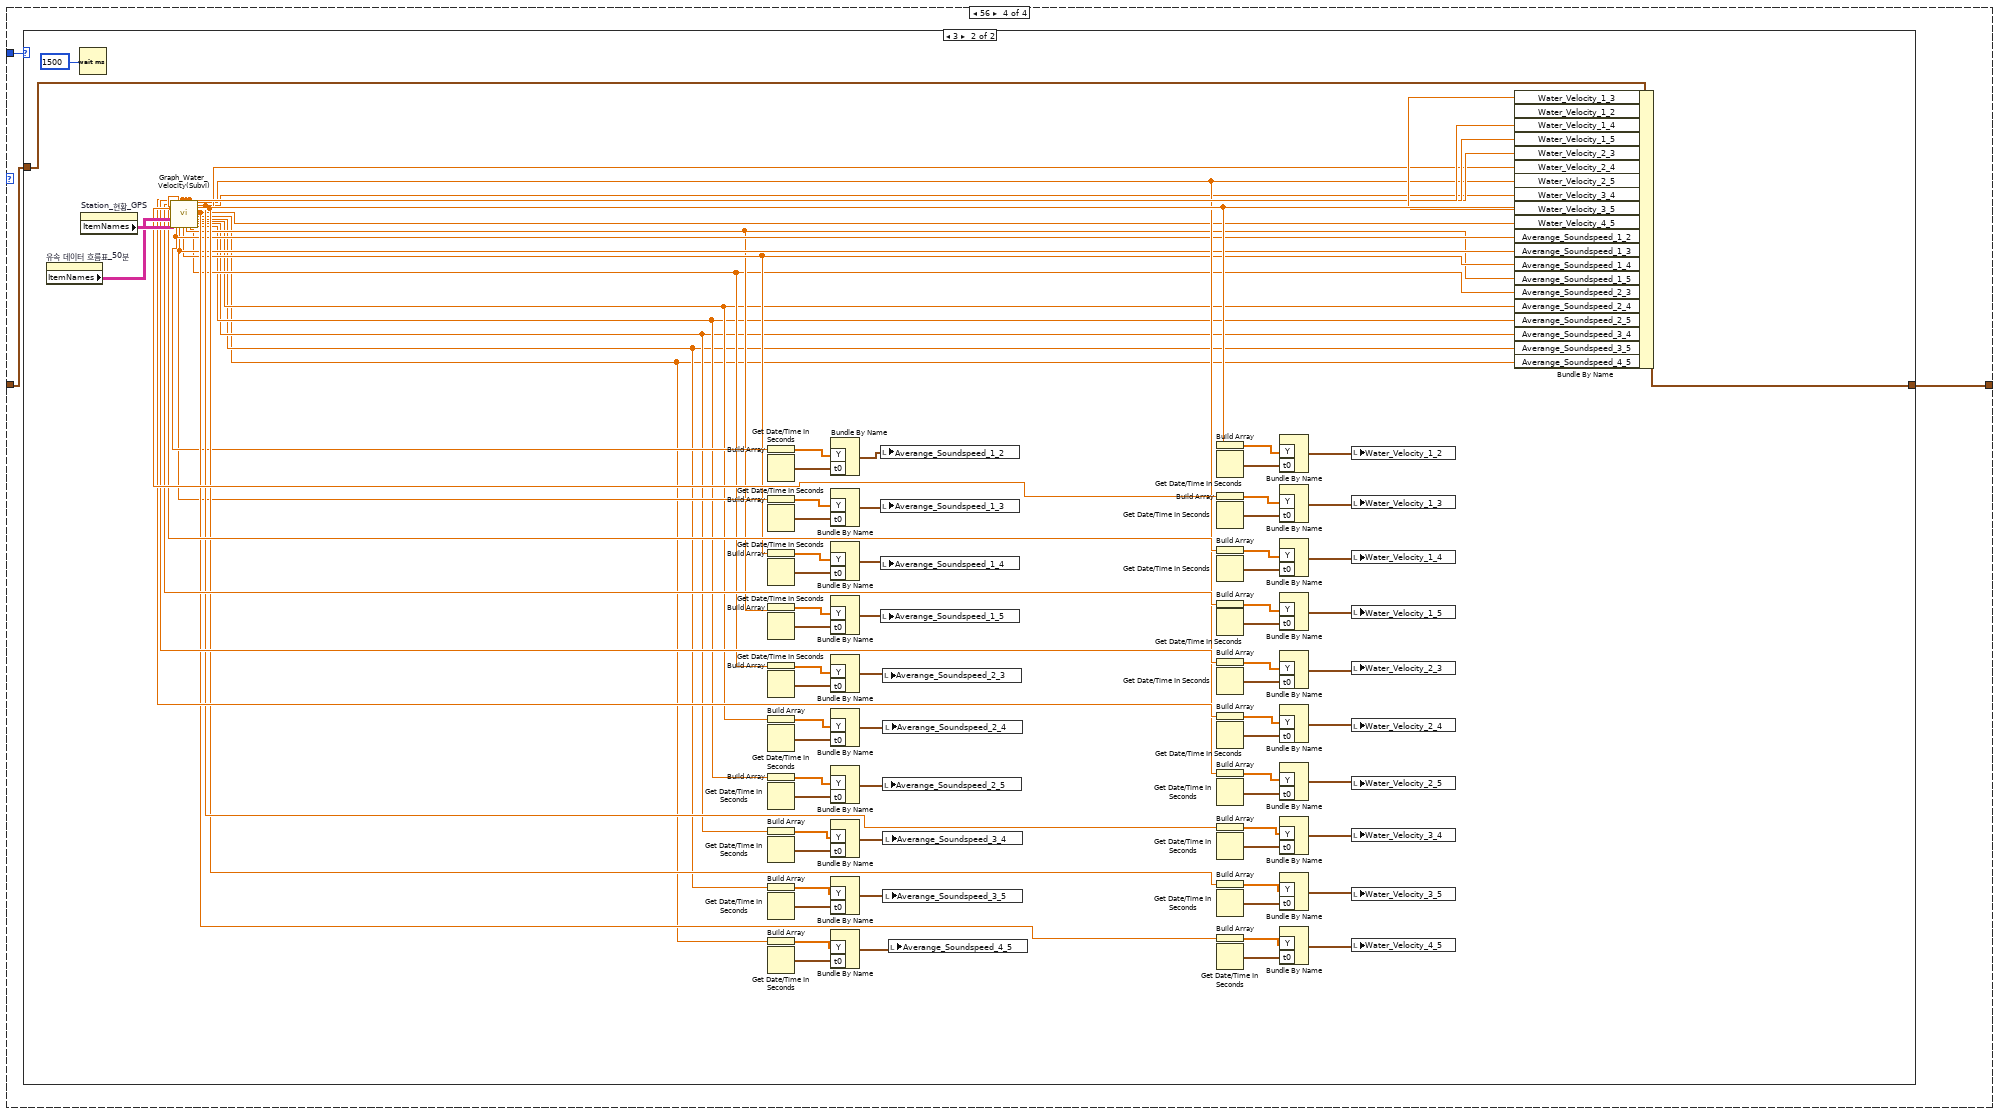
[diagram p8: hidden frame]
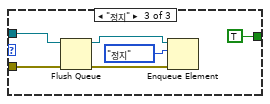
[diagram p11: hidden frame]
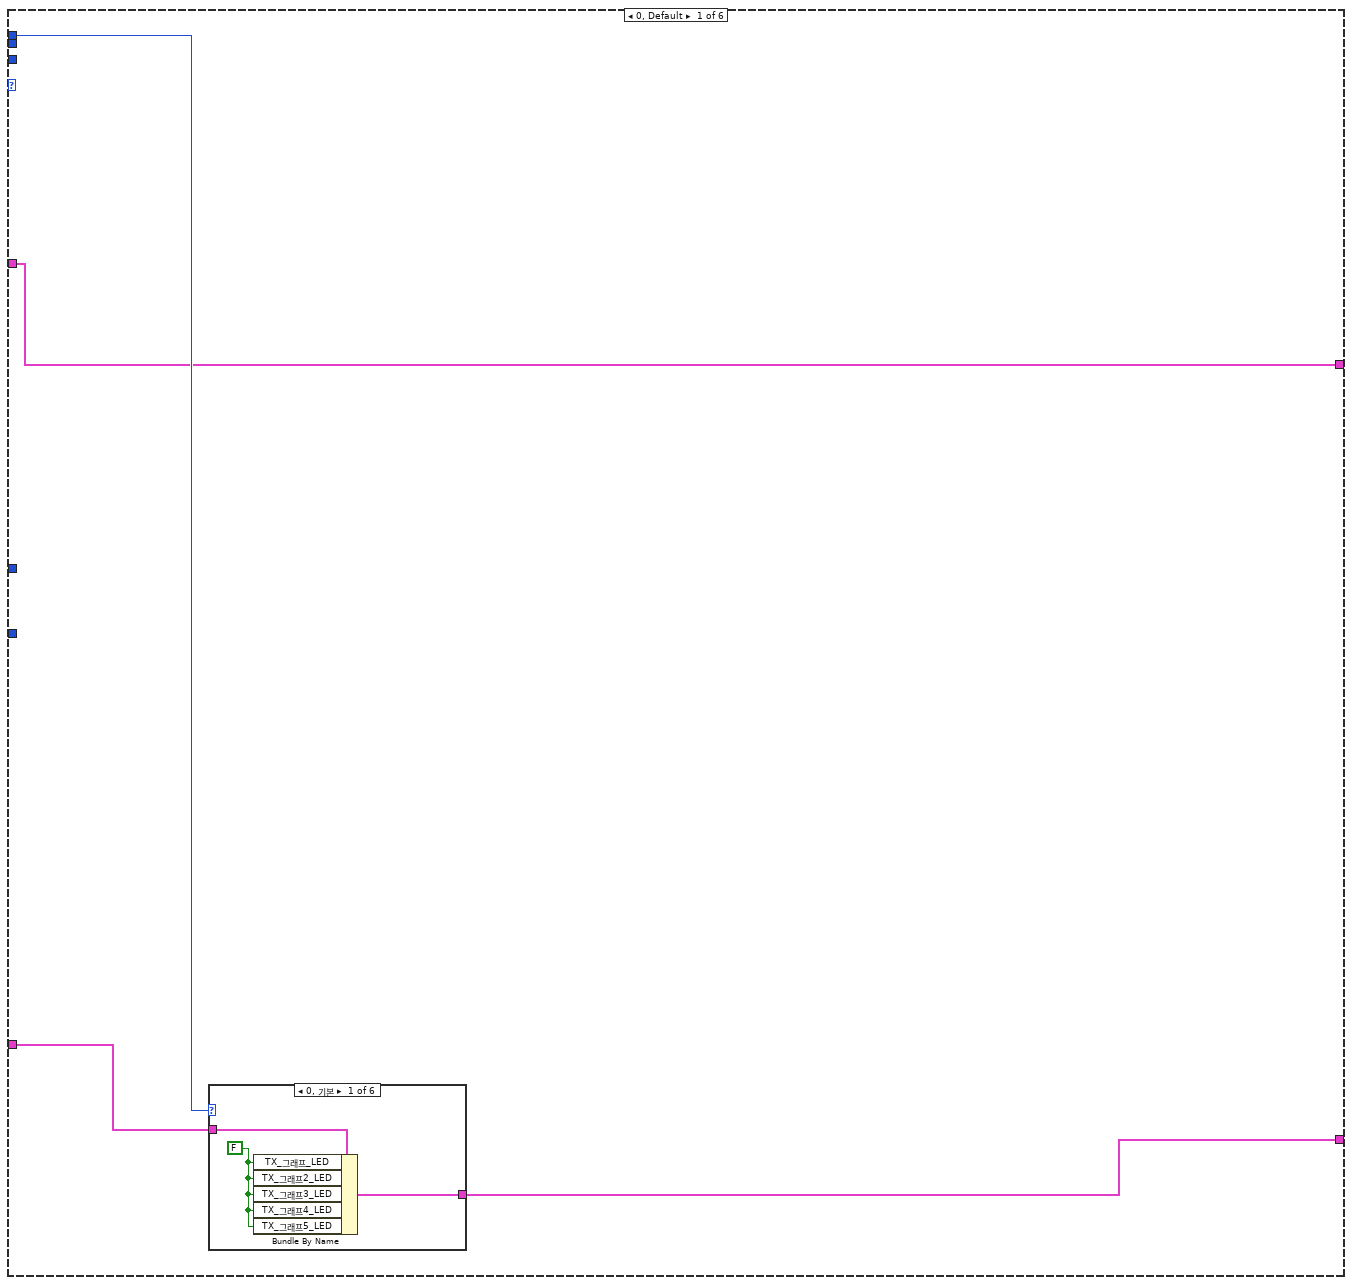
[diagram p12: hidden frame]
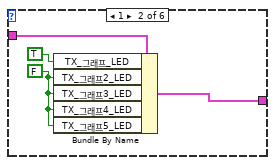
[diagram p13: hidden frame]
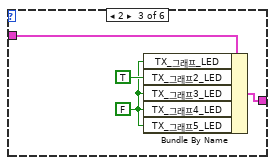
[diagram p14: hidden frame]
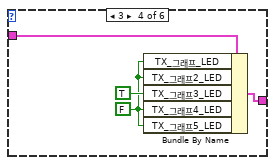
[diagram p15: hidden frame]
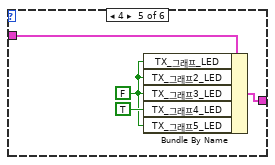
[diagram p16: hidden frame]
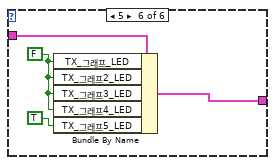
[diagram p17: hidden frame]
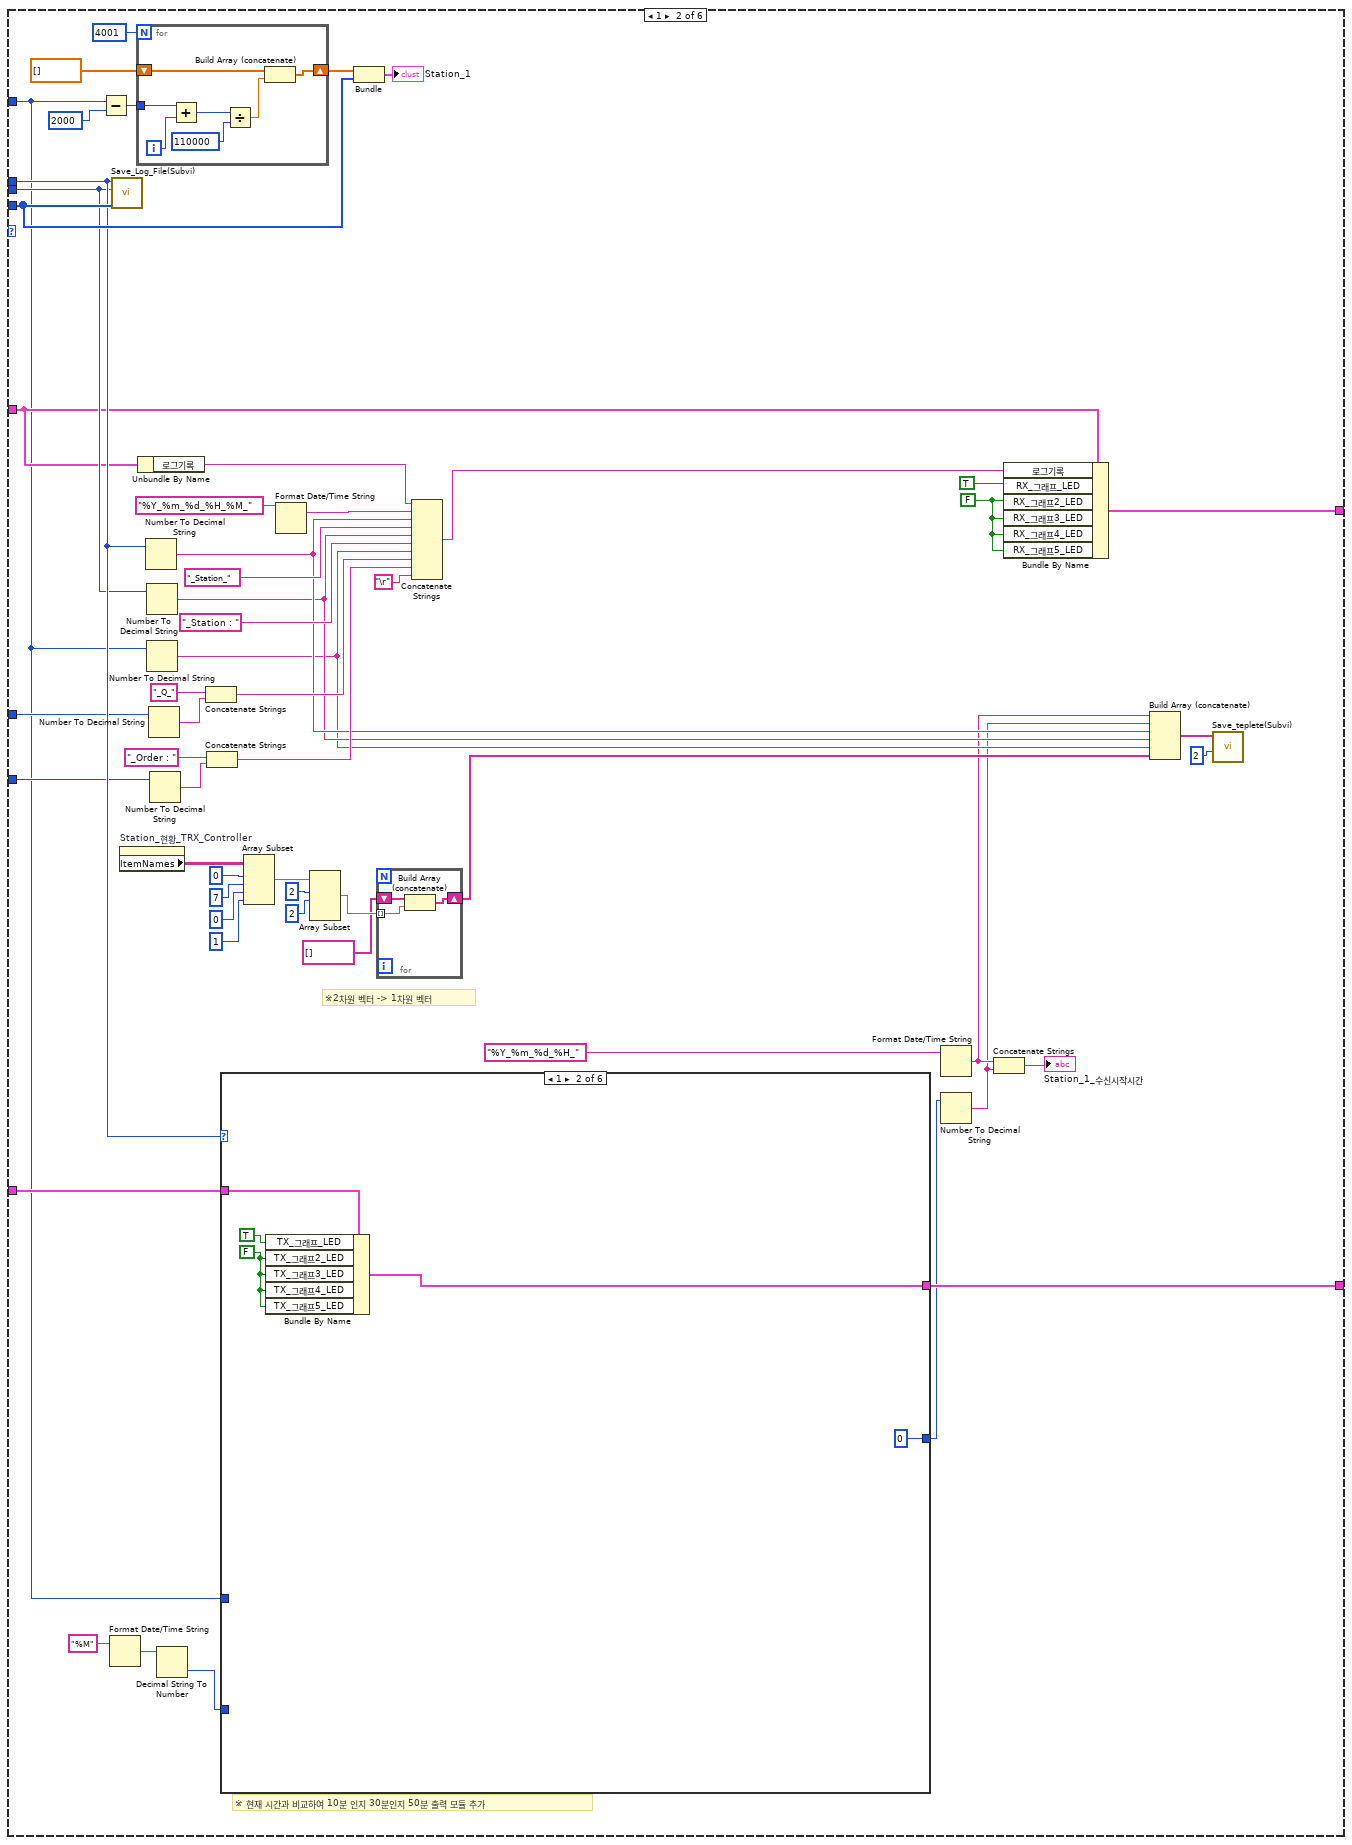
[diagram p18: hidden frame]
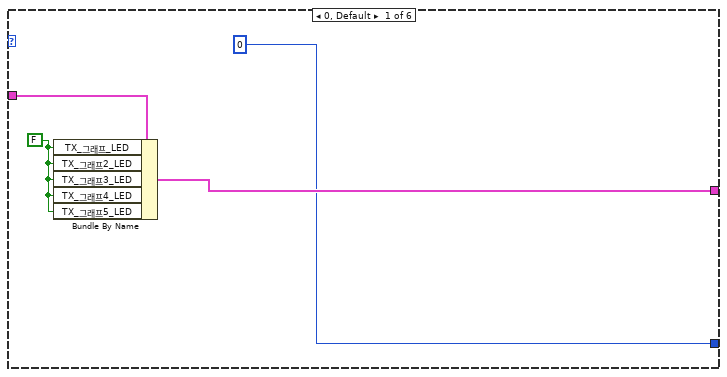
[diagram p19: hidden frame]
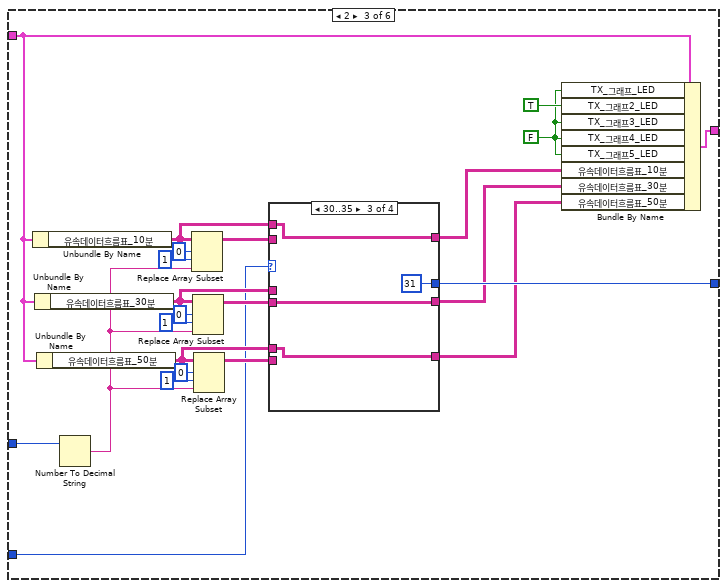
[diagram p20: hidden frame]
diagram:
  w24 = string[] []
  w25 = Brain_Loop_CTL."초기화"
  # "※ 현재 시간과 비교하여 10분 인지 30분인지 50분 출력 모듈 추가"
  # "Queue4: GPSDATA_처리 LOOP"
  # "GPS_리스트 박스 데이터 초기 값"
  # "TRX_Controller_리스트 박스 데이터 초기 값"
  # "Date: 2024.02.05\nTitle: Costal Acoustic Tmography GUI V1.1\nBy: KangJinSeong"
  n1 = Obtain Queue(element data type=w24) -> (queue out=w23:refnum<queue>, error out=w22:errorcluster)  [unwired: 4 in, 1 out]
  n2 = Obtain Queue(element data type=w24) -> (queue out=w12:refnum<queue>, error out=w11:errorcluster)  [unwired: 4 in, 1 out]
  n3 = Obtain Queue(element data type=w24) -> (queue out=w21:refnum<queue>, error out=w20:errorcluster)  [unwired: 4 in, 1 out]
  n4 = Obtain Queue(element data type=w25) -> (queue out=w28:refnum<queue>, error out=w30:errorcluster)  [unwired: 4 in, 1 out]
  n5 = Obtain Queue(element data type=w25) -> (queue out=w7:refnum<queue>, error out=w6:errorcluster)  [unwired: 4 in, 1 out]
  n6 = Enqueue Element(queue=w28, element=w25, error in (no error)=w30) -> (queue out=w19:refnum<queue>, error out=w29:errorcluster)  [unwired: 1 in, 1 out]
  n7 = while {
    tunnel: w19 -> [w33]
    shift-right: [w32] -> w27
    shift-left: w29 -> [w34]
    stop <- w31 stop-if-true
    n8 = event shown="[7] \"SET 버튼\": 값 변경" {
      selector: _ -> [_ _ _ _ _ _ _ _]
      dyn-events: _ -> [_ _ _ _ _ _ _ _]
      timeout: _ -> [_ _ _ _ _ _ _ _]
      tunnel: w34 -> [w39 w44 w46 w51 w59 w64 w70 w73]
      tunnel: w33 -> [w38 w43 w48 w53 w58 w63 w69 w74]
      tunnel: [w36 w41 w47 w52 w56 w62 w67 w71] -> _
      tunnel: [w35 w40 w45 w50 w55 w61 w66 w72] -> w32
      tunnel: [_ _ _ _ _ _ TRUE _] -> w31
      event Value Change {
        n9 = event-data() -> ()  [unwired: 1 in, 1 out]
        n10 = Enqueue Element(queue=w38, element=Brain_Loop_CTL."지도", error in (no error)=w39) -> (queue out=w36:refnum<queue>, error out=w35:errorcluster)  [unwired: 1 in, 1 out]
      }
      event Value Change {
        n11 = event-data() -> ()  [unwired: 1 in, 1 out]
        n12 = Enqueue Element(queue=w43, element=Brain_Loop_CTL."데이터통계", error in (no error)=w44) -> (queue out=w41:refnum<queue>, error out=w40:errorcluster)  [unwired: 1 in, 1 out]
      }
      event "적용 버튼": Value Change {
        n13 = event-data() -> ()  [unwired: 1 in, 1 out]
        n14 = Enqueue Element(queue=w48, element=Brain_Loop_CTL."Mqtt_Publish", error in (no error)=w46) -> (queue out=w47:refnum<queue>, error out=w45:errorcluster)  [unwired: 1 in, 1 out]
      }
      event "Wake_UP버튼": Value Change {
        n15 = event-data() -> ()  [unwired: 1 in, 1 out]
        n16 = Enqueue Element(queue=w53, element=Brain_Loop_CTL."Mqtt_Publish_2", error in (no error)=w51) -> (queue out=w52:refnum<queue>, error out=w50:errorcluster)  [unwired: 1 in, 1 out]
      }
      event Value Change {
        n17 = event-data() -> ()  [unwired: 1 in, 1 out]
        n18 = Enqueue Element(queue=w58, element=Brain_Loop_CTL."관리자", error in (no error)=w59) -> (queue out=w56:refnum<queue>, error out=w55:errorcluster)  [unwired: 1 in, 1 out]
      }
      event Value Change {
        n19 = event-data() -> ()  [unwired: 1 in, 1 out]
        n20 = Enqueue Element(queue=w63, element=Brain_Loop_CTL."유속 데이터", error in (no error)=w64) -> (queue out=w62:refnum<queue>, error out=w61:errorcluster)  [unwired: 1 in, 1 out]
      }
      event "정지": Value Change {
        n21 = event-data() -> ()  [unwired: 1 in, 1 out]
        n22 = Enqueue Element(queue=w69, element=Brain_Loop_CTL."정지", error in (no error)=w70) -> (queue out=w67:refnum<queue>, error out=w66:errorcluster)  [unwired: 1 in, 1 out]
      }
      event "SET 버튼": Value Change {
        n23 = event-data() -> ()  [unwired: 1 in, 1 out]
        n24 = Enqueue Element(queue=w74, element=Brain_Loop_CTL."초기화", error in (no error)=w73) -> (queue out=w71:refnum<queue>, error out=w72:errorcluster)  [unwired: 1 in, 1 out]
      }
    }
  }
  n25 = while {
    tunnel: w7 -> [w88]
    tunnel: w6 -> [w87]
    tunnel: w23 -> [w83]
    tunnel: w22 -> [w82]
    tunnel: [errorcluster {"status"=FALSE, "code"=0, "source"=""} ("에러 상수")] -> w16
    tunnel: w12 -> [w80]
    tunnel: w11 -> [w79]
    tunnel: w21 -> [w78]
    tunnel: w20 -> [w77]
    stop <- w86 stop-if-true
    # "Mqtt_Subscribe_Loop\n※ Brain_Loop의 Queue 값의 따라 작동(Mqtt_Subscribe, 정지, 초기화)"
    n26 = Dequeue Element(queue=w88, error in (no error)=w87) -> (queue out=w85:refnum<queue>, element=w76:T9, error out=w84:errorcluster)  [unwired: 1 in, 1 out]
    n27 = case shown="\"Mqtt_Subscribe\"" w76 {
      tunnel: [_ _ TRUE] -> w86
      tunnel: w85 -> [_ w109 w117]
      tunnel: w84 -> [_ w108 w116]
      tunnel: w83 -> [_ w106 _]
      tunnel: w82 -> [_ w105 _]
      tunnel: w80 -> [_ w104 _]
      tunnel: w79 -> [_ w103 _]
      tunnel: w78 -> [_ w102 _]
      tunnel: w77 -> [_ w101 _]
      frame "초기화", Default {
      }
      frame "Mqtt_Subscribe" {
        # "※ Queue 값의 따라 Python 모듈을 실행 해당 값을 통해 각 Loop 값에 데이터 전달"
        n28 = local read "Python 경로"() -> (w90:path)
        n29 = Enqueue Element(queue=w109, element=Brain_Loop_CTL."Mqtt_Subscribe", error in (no error)=w108) -> ()  [unwired: 1 in, 3 out]
        n30 = Open Python Session(python version="3.9" ("Python 버전"), python path=w90) -> (session out=w95:refnum<k35>, error out=w111:errorcluster)  [unwired: 1 in]
        n31 = local read "Subscribe_모듈 경로"() -> (w89:path)
        n32 = node(w95, w89, "Mqtt_Subscribe" ("함수 이름"), w111, "") -> (w97:refnum<k35>, w96:errorcluster, w93:string)  [unwired: 2 out]
        "디버깅 로그 기록" <- w93
        n33 = Close Python Session(session in=w97, error in=w96) -> (11:w92:errorcluster)
        n34 = call "Split_Queue(Subvi).vi"("입력 문자열"=w93) -> ("Split_Queue2_Result"=w100:string[], "Split_Queue3_Result"=w99:string[], "Split_Queue4_Result"=w98:string[])  [unwired: 5 in, 3 out]
        n35 = call <vilib>:"Clear Errors.vi"("error in (no error)"=w92, "specific error code to clear (0: all)"=0) -> ()  [unwired: 4 in, 2 out]
        n36 = Enqueue Element(queue=w106, element=w100, error in (no error)=w105) -> ()  [unwired: 1 in, 3 out]
        n37 = Enqueue Element(queue=w102, element=w98, error in (no error)=w101) -> ()  [unwired: 1 in, 3 out]
        n38 = Enqueue Element(queue=w104, element=w99, error in (no error)=w103) -> ()  [unwired: 1 in, 3 out]
      }
      frame "정지" {
        # "※ Queue 값의 따라 정지 인경우 해당 큐를 비우고 정지 전달"
        n39 = Flush Queue(queue=w117, error in (no error)=w116) -> (queue out=w115:refnum<queue>, error out=w114:errorcluster)  [unwired: 1 out]
        n40 = Enqueue Element(queue=w115, element=Brain_Loop_CTL."정지", error in (no error)=w114) -> ()  [unwired: 1 in, 3 out]
      }
    }
  }
  n41 = while "While 루프" {
    tunnel: w7 -> [w154]
    tunnel: w6 -> [w153]
    tunnel: w12 -> [w152]
    tunnel: w11 -> [w151]
    shift-right: [w134] -> _
    shift-left: T7 {"TX_그래프_LED"=FALSE, "TX_그래프2_LED"=FALSE, "TX_그래프3_LED"=FALSE, "TX_그래프4_LED"=FALSE, "TX_그래프5_LED"=FALSE, "유속데이터흐름표_10분"=[["", "", "", "", "", ""], ["", "", "", "", "", ""], ["", "", "", "", "", ""], ["", "", "", "", "", ""], ["", "", "", "", "", ""], ["", "", "", "", "", "0"]], "유속데이터흐름표_30분"=[["", "", "", "", "", ""], ["", "", "", "", "", ""], ["", "", "", "", "", ""], ["", "", "", "", "", ""], ["", "", "", "", "", ""], ["", "", "", "", "", "0"]], "유속데이터흐름표_50분"=[["", "", "", "", "", ""], ["", "", "", "", "", ""], ["", "", "", "", "", ""], ["", "", "", "", "", ""], ["", "", "", "", "", ""], ["", "", "", "", "", "0"]]} -> [w140]
    shift-right: [w129] -> _
    shift-left: T6 {"로그기록"="", "RX_그래프_LED"=FALSE, "RX_그래프2_LED"=FALSE, "RX_그래프3_LED"=FALSE, "RX_그래프4_LED"=FALSE, "RX_그래프5_LED"=FALSE} -> [w133]
    tunnel: [errorcluster {"status"=FALSE, "code"=0, "source"=""} ("에러 상수")] -> w4
    stop <- w155 stop-if-true
    # "※ Queue3 처리 LOOP에 데이터가 들어오는 경우 각 인덱스에 맞게 데이터 분리 후 웨이브폼 그래프에 표시\n   TX_Station/RX_Station 값에 따라 .CSV 파일로 데이터 저장"
    # "※ TX_Station 번호 별로 그래프 하단에 LED 점멸(빨간색)\n    RX_Station 번호 별로 그래프 하단에 LED 점멸(파란색)"
    # "0 index: TX_Station\n1 index: RX_Station\n2 index: Max index"
    # "FPGA 신호처리된 결과값"
    # "Queue3: SIGDATA 처리 LOOP\n신호처리된 데이터 가시화 경우 시간 데이터로 표시"
    n42 = Dequeue Element(queue=w154, error in (no error)=w153) -> (queue out=w157:refnum<queue>, element=w156:T9, error out=w158:errorcluster)  [unwired: 1 in, 1 out]
    n43 = Dequeue Element(queue=w152, error in (no error)=w151) -> (element=w150:string[])  [unwired: 1 in, 3 out]
    n44 = case shown="\"Mqtt_Subscribe\"" w156 {
      tunnel: [_ _ TRUE] -> w155
      tunnel: w157 -> [_ w1337 w1342]
      tunnel: w158 -> [_ w1336 w1341]
      frame "초기화", Default {
      }
      frame "Mqtt_Subscribe" {
        n45 = Enqueue Element(queue=w1337, element=Brain_Loop_CTL."Mqtt_Subscribe", error in (no error)=w1336) -> ()  [unwired: 1 in, 3 out]
      }
      frame "정지" {
        n46 = Flush Queue(queue=w1342, error in (no error)=w1341) -> (queue out=w1340:refnum<queue>, error out=w1339:errorcluster)  [unwired: 1 out]
        n47 = Enqueue Element(queue=w1340, element=Brain_Loop_CTL."정지", error in (no error)=w1339) -> ()  [unwired: 1 in, 3 out]
      }
    }
    n48 = Decimal String To Number(string=w150) -> (number=w142:i32[])  [unwired: 2 in, 1 out]
    n49 = Array Subset(array=w142, index=4 ("인덱스"), length=4000 ("길이")) -> (w120:i32[])
    n50 = Index Array(array=w142, index #1=1 ("인덱스"), index #2=0 ("인덱스"), index #3=2 ("인덱스")) -> (element #1=w143:i32, element #2=w144:i32, element #3=w141:i32)
    n51 = local read "Order"() -> (w131:i32)
    n52 = local read "Q 값"() -> (w132:i32)
    n53 = case shown="3" w143 {
      tunnel: w144 -> [w162 w219 w424 w652 w880 w1110]
      tunnel: w143 -> [_ w218 w445 w679 w908 w1138]
      tunnel: w120 -> [_ w235 w465 w695 w925 w1155]
      tunnel: w141 -> [_ w190 w421 w651 w879 w1109]
      tunnel: w140 -> [w161 w233 w423 w653 w881 w1111]
      tunnel: [w160 w232 w420 w649 w882 w1112] -> w134
      tunnel: w133 -> [w159 w215 w446 w680 w909 w1139]
      tunnel: w132 -> [_ w217 w448 w678 w907 w1137]
      tunnel: w131 -> [_ w216 w447 w677 w906 w1136]
      tunnel: [w159 w211 w449 w681 w910 w1140] -> w129
      frame 0, Default {
        n54 = case shown="0, 기본" w162 {
          tunnel: w161 -> [w165 w169 w173 w177 w181 w185]
          tunnel: [w164 w166 w172 w176 w180 w184] -> w160
          frame 0, Default {
            w163 = FALSE
            n55 = Bundle By Name(cluster=w165, "TX_그래프_LED"=w163, "TX_그래프2_LED"=w163, "TX_그래프3_LED"=w163, "TX_그래프4_LED"=w163, "TX_그래프5_LED"=w163) -> (w164:T7)
          }
          frame 1 {
            w167 = FALSE
            n56 = Bundle By Name(cluster=w169, "TX_그래프_LED"=TRUE, "TX_그래프2_LED"=w167, "TX_그래프3_LED"=w167, "TX_그래프4_LED"=w167, "TX_그래프5_LED"=w167) -> (w166:T7)
          }
          frame 2 {
            w170 = FALSE
            n57 = Bundle By Name(cluster=w173, "TX_그래프_LED"=w170, "TX_그래프2_LED"=TRUE, "TX_그래프3_LED"=w170, "TX_그래프4_LED"=w170, "TX_그래프5_LED"=w170) -> (w172:T7)
          }
          frame 3 {
            w174 = FALSE
            n58 = Bundle By Name(cluster=w177, "TX_그래프_LED"=w174, "TX_그래프2_LED"=w174, "TX_그래프3_LED"=TRUE, "TX_그래프4_LED"=w174, "TX_그래프5_LED"=w174) -> (w176:T7)
          }
          frame 4 {
            w178 = FALSE
            n59 = Bundle By Name(cluster=w181, "TX_그래프_LED"=w178, "TX_그래프2_LED"=w178, "TX_그래프3_LED"=w178, "TX_그래프4_LED"=TRUE, "TX_그래프5_LED"=w178) -> (w180:T7)
          }
          frame 5 {
            w182 = FALSE
            n60 = Bundle By Name(cluster=w185, "TX_그래프_LED"=w182, "TX_그래프2_LED"=w182, "TX_그래프3_LED"=w182, "TX_그래프4_LED"=w182, "TX_그래프5_LED"=TRUE) -> (w184:T7)
          }
        }
      }
      frame 1 {
        w212 = FALSE
        # "※ 현재 시간과 비교하여 10분 인지 30분인지 50분 출력 모듈 추가"
        # "※2차원 벡터 -> 1차원 벡터"
        n61 = Subtract(x=w190, y=2000) -> (x-y=w238:i32)
        n62 = Format Date/Time String(time format string (%c)="%M" ("시간 포맷 문자열 (%c)")) -> (date/time string=w189:string)  [unwired: 2 in]
        n63 = call "Save_Log_File(Subvi).vi"("TX_Station"=w219, "RX_Station"=w218, "1D data"=w235) -> ()  [unwired: 7 in, 1 out]
        n64 = property on="Station_현황_TRX_Controller" class="MCListbox (엄격한)"() -> ("ItemNames"=w206:string[][])  [unwired: 2 in, 2 out]
        n65 = for {
          N: 4001 -> [_]
          tunnel: w238 -> [w415]
          shift-right: [w410] -> w236
          shift-left: dbl[] [] -> [w412]
          i -> [w409]
          n66 = Add(x=w415, y=w409) -> (x+y=w414:i32)
          n67 = Divide(x=w414, y=110000) -> (x/y=w411:dbl)
          n68 = Build Array (concatenate)(w412, w411) -> (w410:dbl[])
        }
        n69 = Unbundle By Name(w215) -> ("로그기록"=w220:string)
        n70 = Number To Decimal String(number=w219) -> (decimal integer string=w200:string)  [unwired: 1 in]
        n71 = Number To Decimal String(number=w218) -> (decimal integer string=w199:string)  [unwired: 1 in]
        n72 = Number To Decimal String(number=w190) -> (decimal integer string=w198:string)  [unwired: 1 in]
        n73 = Number To Decimal String(number=w217) -> (decimal integer string=w227:string)  [unwired: 1 in]
        n74 = Number To Decimal String(number=w216) -> (decimal integer string=w226:string)  [unwired: 1 in]
        n75 = Decimal String To Number(string=w189) -> (number=w187:i32)  [unwired: 2 in, 1 out]
        n76 = Concatenate Strings("_Q_" ("시간 포맷 문자열 (%c)"), w227) -> (w224:string)
        n77 = Concatenate Strings("_Order : " ("시간 포맷 문자열 (%c)"), w226) -> (w223:string)
        n78 = case shown="1" w219 {
          tunnel: w233 -> [w247 w252 w266 w298 w337 w374]
          tunnel: [w246 w249 w269 w314 w353 w392] -> w232
          tunnel: [0 0 w273 w296 w335 w376] -> w209
          tunnel: w190 -> [_ _ w270 w297 w336 w375]
          tunnel: w187 -> [_ _ w253 w292 w331 w370]
          frame 0, Default {
            w245 = FALSE
            n79 = Bundle By Name(cluster=w247, "TX_그래프_LED"=w245, "TX_그래프2_LED"=w245, "TX_그래프3_LED"=w245, "TX_그래프4_LED"=w245, "TX_그래프5_LED"=w245) -> (w246:T7)
          }
          frame 1 {
            w250 = FALSE
            n80 = Bundle By Name(cluster=w252, "TX_그래프_LED"=TRUE, "TX_그래프2_LED"=w250, "TX_그래프3_LED"=w250, "TX_그래프4_LED"=w250, "TX_그래프5_LED"=w250) -> (w249:T7)
          }
          frame 2 {
            w274 = FALSE
            n81 = Unbundle By Name(w266) -> ("유속데이터흐름표_10분"=w254:string[][])
            n82 = Unbundle By Name(w266) -> ("유속데이터흐름표_30분"=w256:string[][])
            n83 = Unbundle By Name(w266) -> ("유속데이터흐름표_50분"=w255:string[][])
            n84 = Number To Decimal String(number=w270) -> (decimal integer string=w263:string)  [unwired: 1 in]
            n85 = Replace Array Subset(array=w254, new element=w263, index (row)=0 ("인덱스 (행)"), index (col)=1 ("비활성화된 인덱스 (열)")) -> (w262:string[][])
            n86 = Replace Array Subset(array=w256, new element=w263, index (row)=0 ("인덱스 (행)"), index (col)=1 ("비활성화된 인덱스 (열)")) -> (w261:string[][])
            n87 = Replace Array Subset(array=w255, new element=w263, index (row)=0 ("인덱스 (행)"), index (col)=1 ("비활성화된 인덱스 (열)")) -> (w260:string[][])
            n88 = case shown="30..35" w253 {
              tunnel: [0 11 31 51] -> w273
              tunnel: w262 -> [_ w282 _ _]
              tunnel: w261 -> [_ _ w285 _]
              tunnel: w260 -> [_ _ _ w288]
              tunnel: [w278 w282 w286 w290] -> w259
              tunnel: [w277 w281 w285 w289] -> w258
              tunnel: [w276 w280 w284 w288] -> w257
              tunnel: w256 -> [w277 w281 _ w289]
              tunnel: w255 -> [w276 w280 w284 _]
              tunnel: w254 -> [w278 _ w286 w290]
              frame 0, Default {
              }
              frame 10..15 {
              }
              frame 30..35 {
              }
              frame 50..55 {
              }
            }
            n89 = Bundle By Name(cluster=w266, "TX_그래프_LED"=w274, "TX_그래프2_LED"=TRUE, "TX_그래프3_LED"=w274, "TX_그래프4_LED"=w274, "TX_그래프5_LED"=w274, "유속데이터흐름표_10분"=w259, "유속데이터흐름표_30분"=w258, "유속데이터흐름표_50분"=w257) -> (w269:T7)
          }
          frame 3 {
            w312 = FALSE
            n90 = Unbundle By Name(w298) -> ("유속데이터흐름표_10분"=w311:string[][])
            n91 = Unbundle By Name(w298) -> ("유속데이터흐름표_30분"=w309:string[][])
            n92 = Unbundle By Name(w298) -> ("유속데이터흐름표_50분"=w310:string[][])
            n93 = Number To Decimal String(number=w297) -> (decimal integer string=w305:string)  [unwired: 1 in]
            n94 = Replace Array Subset(array=w311, new element=w305, index (row)=0 ("인덱스 (행)"), index (col)=2 ("비활성화된 인덱스 (열)")) -> (w306:string[][])
            n95 = Replace Array Subset(array=w309, new element=w305, index (row)=0 ("인덱스 (행)"), index (col)=2 ("비활성화된 인덱스 (열)")) -> (w307:string[][])
            n96 = Replace Array Subset(array=w310, new element=w305, index (row)=0 ("인덱스 (행)"), index (col)=2 ("비활성화된 인덱스 (열)")) -> (w308:string[][])
            n97 = case shown="50..55" w292 {
              tunnel: [0 12 32 52] -> w296
              tunnel: w306 -> [_ w321 _ _]
              tunnel: w307 -> [_ _ w324 _]
              tunnel: w308 -> [_ _ _ w327]
              tunnel: [w317 w321 w325 w329] -> w295
              tunnel: [w316 w320 w324 w328] -> w294
              tunnel: [w315 w319 w323 w327] -> w293
              tunnel: w309 -> [w316 w320 _ w328]
              tunnel: w310 -> [w315 w319 w323 _]
              tunnel: w311 -> [w317 _ w325 w329]
              frame 0, Default {
              }
              frame 10..15 {
              }
              frame 30..35 {
              }
              frame 50..55 {
              }
            }
            n98 = Bundle By Name(cluster=w298, "TX_그래프_LED"=w312, "TX_그래프2_LED"=w312, "TX_그래프3_LED"=TRUE, "TX_그래프4_LED"=w312, "TX_그래프5_LED"=w312, "유속데이터흐름표_10분"=w295, "유속데이터흐름표_30분"=w294, "유속데이터흐름표_50분"=w293) -> (w314:T7)
          }
          frame 4 {
            w351 = FALSE
            n99 = Unbundle By Name(w337) -> ("유속데이터흐름표_10분"=w350:string[][])
            n100 = Unbundle By Name(w337) -> ("유속데이터흐름표_30분"=w348:string[][])
            n101 = Unbundle By Name(w337) -> ("유속데이터흐름표_50분"=w349:string[][])
            n102 = Number To Decimal String(number=w336) -> (decimal integer string=w344:string)  [unwired: 1 in]
            n103 = Replace Array Subset(array=w350, new element=w344, index (row)=0 ("인덱스 (행)"), index (col)=3 ("비활성화된 인덱스 (열)")) -> (w345:string[][])
            n104 = Replace Array Subset(array=w348, new element=w344, index (row)=0 ("인덱스 (행)"), index (col)=3 ("비활성화된 인덱스 (열)")) -> (w346:string[][])
            n105 = Replace Array Subset(array=w349, new element=w344, index (row)=0 ("인덱스 (행)"), index (col)=3 ("비활성화된 인덱스 (열)")) -> (w347:string[][])
            n106 = case shown="10..15" w331 {
              tunnel: [0 13 33 53] -> w335
              tunnel: w345 -> [_ w360 _ _]
              tunnel: w346 -> [_ _ w363 _]
              tunnel: w347 -> [_ _ _ w366]
              tunnel: [w356 w360 w364 w368] -> w334
              tunnel: [w355 w359 w363 w367] -> w333
              tunnel: [w354 w358 w362 w366] -> w332
              tunnel: w348 -> [w355 w359 _ w367]
              tunnel: w349 -> [w354 w358 w362 _]
              tunnel: w350 -> [w356 _ w364 w368]
              frame 0, Default {
              }
              frame 10..15 {
              }
              frame 30..35 {
              }
              frame 50..55 {
              }
            }
            n107 = Bundle By Name(cluster=w337, "TX_그래프_LED"=w351, "TX_그래프2_LED"=w351, "TX_그래프3_LED"=w351, "TX_그래프4_LED"=TRUE, "TX_그래프5_LED"=w351, "유속데이터흐름표_10분"=w334, "유속데이터흐름표_30분"=w333, "유속데이터흐름표_50분"=w332) -> (w353:T7)
          }
          frame 5 {
            w390 = FALSE
            n108 = Unbundle By Name(w374) -> ("유속데이터흐름표_10분"=w389:string[][])
            n109 = Unbundle By Name(w374) -> ("유속데이터흐름표_30분"=w387:string[][])
            n110 = Unbundle By Name(w374) -> ("유속데이터흐름표_50분"=w388:string[][])
            n111 = Number To Decimal String(number=w375) -> (decimal integer string=w383:string)  [unwired: 1 in]
            n112 = Replace Array Subset(array=w389, new element=w383, index (row)=0 ("인덱스 (행)"), index (col)=4 ("비활성화된 인덱스 (열)")) -> (w384:string[][])
            n113 = Replace Array Subset(array=w387, new element=w383, index (row)=0 ("인덱스 (행)"), index (col)=4 ("비활성화된 인덱스 (열)")) -> (w385:string[][])
            n114 = Replace Array Subset(array=w388, new element=w383, index (row)=0 ("인덱스 (행)"), index (col)=4 ("비활성화된 인덱스 (열)")) -> (w386:string[][])
            n115 = case shown="50..55" w370 {
              tunnel: [0 14 34 54] -> w376
              tunnel: w384 -> [_ w399 _ _]
              tunnel: w385 -> [_ _ w402 _]
              tunnel: w386 -> [_ _ _ w405]
              tunnel: [w395 w399 w403 w407] -> w373
              tunnel: [w394 w398 w402 w406] -> w372
              tunnel: [w393 w397 w401 w405] -> w371
              tunnel: w387 -> [w394 w398 _ w406]
              tunnel: w388 -> [w393 w397 w401 _]
              tunnel: w389 -> [w395 _ w403 w407]
              frame 0, Default {
              }
              frame 10..15 {
              }
              frame 30..35 {
              }
              frame 50..55 {
              }
            }
            n116 = Bundle By Name(cluster=w374, "TX_그래프_LED"=w390, "TX_그래프2_LED"=w390, "TX_그래프3_LED"=w390, "TX_그래프4_LED"=w390, "TX_그래프5_LED"=TRUE, "유속데이터흐름표_10분"=w373, "유속데이터흐름표_30분"=w372, "유속데이터흐름표_50분"=w371) -> (w392:T7)
          }
        }
        n117 = Array Subset(array=w206, index (row)=0 ("인덱스"), length (row)=7 ("길이"), index (col)=0 ("인덱스"), length (col)=1 ("길이")) -> (w186:string[][])
        n118 = Format Date/Time String(time format string (%c)="%Y_%m_%d_%H_%M_" ("시간 포맷 문자열 (%c)")) -> (date/time string=w221:string)  [unwired: 2 in]
        n119 = Array Subset(array=w186, index (row)=2 ("인덱스"), length (row)=2 ("길이")) -> (w197:string[][])  [unwired: 2 in]
        n120 = Bundle(w236, w235) -> (→"Station_1":cluster{dbl[], i32[]})  [unwired: 1 in]
        n121 = for {
          tunnel: w197 -> [w242] mode=indexing
          shift-right: [w241] -> w195
          shift-left: string[] [] -> [w243]
          n122 = Build Array (concatenate)(w243, w242) -> (w241:string[])
        }
        n123 = Concatenate Strings(w220, w221, w200, "_Station_" ("시간 포맷 문자열 (%c)"), w199, "_Station : " ("시간 포맷 문자열 (%c)"), w198, w224, w223, "\r") -> (w214:string)
        n124 = Format Date/Time String(time format string (%c)="%Y_%m_%d_%H_" ("시간 포맷 문자열 (%c)")) -> (date/time string=w192:string)  [unwired: 2 in]
        n125 = Number To Decimal String(number=w209) -> (decimal integer string=w191:string)  [unwired: 1 in]
        n126 = Concatenate Strings(w192, w191) -> (→"Station_1_수신시작시간":string)
        n127 = Bundle By Name(cluster=w215, "로그기록"=w214, "RX_그래프_LED"=TRUE, "RX_그래프2_LED"=w212, "RX_그래프3_LED"=w212, "RX_그래프4_LED"=w212, "RX_그래프5_LED"=w212) -> (w211:T6)
        n128 = Build Array (concatenate)(w192, w191, w200, w199, w198, w195) -> (w194:string[])
        n129 = call "Save_teplete(Subvi).vi"("숫자형"=2, "배열"=w194) -> ()  [unwired: 10 in]
      }
      frame 2 {
        w419 = FALSE
        # "※ 2차원 벡터 -> 1차원 벡터"
        n130 = Subtract(x=w421, y=2000) -> (x-y=w468:i32)
        n131 = Format Date/Time String(time format string (%c)="%M" ("시간 포맷 문자열 (%c)")) -> (date/time string=w418:string)  [unwired: 2 in]
        n132 = call "Save_Log_File(Subvi).vi"("TX_Station"=w424, "RX_Station"=w445, "1D data"=w465) -> ()  [unwired: 7 in, 1 out]
        n133 = property on="Station_현황_TRX_Controller" class="MCListbox (엄격한)"() -> ("ItemNames"=w441:string[][])  [unwired: 2 in, 2 out]
        n134 = for {
          N: 4001 -> [_]
          tunnel: w468 -> [w645]
          shift-right: [w640] -> w466
          shift-left: dbl[] [] -> [w642]
          i -> [w639]
          n135 = Add(x=w645, y=w639) -> (x+y=w644:i32)
          n136 = Divide(x=w644, y=110000) -> (x/y=w641:dbl)
          n137 = Build Array (concatenate)(w642, w641) -> (w640:dbl[])
        }
        n138 = Decimal String To Number(string=w418) -> (number=w416:i32)  [unwired: 2 in, 1 out]
        n139 = Unbundle By Name(w446) -> ("로그기록"=w452:string)
        n140 = Number To Decimal String(number=w424) -> (decimal integer string=w429:string)  [unwired: 1 in]
        n141 = Number To Decimal String(number=w445) -> (decimal integer string=w428:string)  [unwired: 1 in]
        n142 = Number To Decimal String(number=w421) -> (decimal integer string=w427:string)  [unwired: 1 in]
        n143 = Number To Decimal String(number=w448) -> (decimal integer string=w459:string)  [unwired: 1 in]
        n144 = Number To Decimal String(number=w447) -> (decimal integer string=w458:string)  [unwired: 1 in]
        n145 = case shown="5" w424 {
          tunnel: w423 -> [w474 w479 w515 w525 w564 w601]
          tunnel: [w473 w495 w516 w541 w580 w619] -> w420
          tunnel: [0 w481 0 w523 w562 w603] -> w422
          tunnel: w421 -> [_ w480 _ w524 w563 w602]
          tunnel: w416 -> [_ w475 _ w519 w558 w597]
          frame 0, Default {
            w472 = FALSE
            n146 = Bundle By Name(cluster=w474, "TX_그래프_LED"=w472, "TX_그래프2_LED"=w472, "TX_그래프3_LED"=w472, "TX_그래프4_LED"=w472, "TX_그래프5_LED"=w472) -> (w473:T7)
          }
          frame 1 {
            w496 = FALSE
            n147 = Unbundle By Name(w479) -> ("유속데이터흐름표_10분"=w482:string[][])
            n148 = Unbundle By Name(w479) -> ("유속데이터흐름표_30분"=w484:string[][])
            n149 = Unbundle By Name(w479) -> ("유속데이터흐름표_50분"=w483:string[][])
            n150 = Number To Decimal String(number=w480) -> (decimal integer string=w488:string)  [unwired: 1 in]
            n151 = Replace Array Subset(array=w482, new element=w488, index (row)=1 ("인덱스 (행)"), index (col)=0 ("비활성화된 인덱스 (열)")) -> (w487:string[][])
            n152 = Replace Array Subset(array=w484, new element=w488, index (row)=1 ("인덱스 (행)"), index (col)=0 ("비활성화된 인덱스 (열)")) -> (w486:string[][])
            n153 = Replace Array Subset(array=w483, new element=w488, index (row)=1 ("인덱스 (행)"), index (col)=0 ("비활성화된 인덱스 (열)")) -> (w485:string[][])
            n154 = case shown="30..35" w475 {
              tunnel: [0 10 30 50] -> w481
              tunnel: w487 -> [_ w504 _ _]
              tunnel: w486 -> [_ _ w507 _]
              tunnel: w485 -> [_ _ _ w510]
              tunnel: [w500 w504 w508 w512] -> w478
              tunnel: [w499 w503 w507 w511] -> w477
              tunnel: [w498 w502 w506 w510] -> w476
              tunnel: w484 -> [w499 w503 _ w511]
              tunnel: w483 -> [w498 w502 w506 _]
              tunnel: w482 -> [w500 _ w508 w512]
              frame 0, Default {
              }
              frame 10..15 {
              }
              frame 30..35 {
              }
              frame 50..55 {
              }
            }
            n155 = Bundle By Name(cluster=w479, "TX_그래프_LED"=TRUE, "TX_그래프2_LED"=w496, "TX_그래프3_LED"=w496, "TX_그래프4_LED"=w496, "TX_그래프5_LED"=w496, "유속데이터흐름표_10분"=w478, "유속데이터흐름표_30분"=w477, "유속데이터흐름표_50분"=w476) -> (w495:T7)
          }
          frame 2 {
            w517 = FALSE
            n156 = Bundle By Name(cluster=w515, "TX_그래프_LED"=w517, "TX_그래프2_LED"=TRUE, "TX_그래프3_LED"=w517, "TX_그래프4_LED"=w517, "TX_그래프5_LED"=w517) -> (w516:T7)
          }
          frame 3 {
            w539 = FALSE
            n157 = Unbundle By Name(w525) -> ("유속데이터흐름표_10분"=w538:string[][])
            n158 = Unbundle By Name(w525) -> ("유속데이터흐름표_30분"=w536:string[][])
            n159 = Unbundle By Name(w525) -> ("유속데이터흐름표_50분"=w537:string[][])
            n160 = Number To Decimal String(number=w524) -> (decimal integer string=w532:string)  [unwired: 1 in]
            n161 = Replace Array Subset(array=w538, new element=w532, index (row)=1 ("인덱스 (행)"), index (col)=2 ("비활성화된 인덱스 (열)")) -> (w533:string[][])
            n162 = Replace Array Subset(array=w536, new element=w532, index (row)=1 ("인덱스 (행)"), index (col)=2 ("비활성화된 인덱스 (열)")) -> (w534:string[][])
            n163 = Replace Array Subset(array=w537, new element=w532, index (row)=1 ("인덱스 (행)"), index (col)=2 ("비활성화된 인덱스 (열)")) -> (w535:string[][])
            n164 = case shown="50..55" w519 {
              tunnel: [0 12 32 52] -> w523
              tunnel: w533 -> [_ w548 _ _]
              tunnel: w534 -> [_ _ w551 _]
              tunnel: w535 -> [_ _ _ w554]
              tunnel: [w544 w548 w552 w556] -> w522
              tunnel: [w543 w547 w551 w555] -> w521
              tunnel: [w542 w546 w550 w554] -> w520
              tunnel: w536 -> [w543 w547 _ w555]
              tunnel: w537 -> [w542 w546 w550 _]
              tunnel: w538 -> [w544 _ w552 w556]
              frame 0, Default {
              }
              frame 10..15 {
              }
              frame 30..35 {
              }
              frame 50..55 {
              }
            }
            n165 = Bundle By Name(cluster=w525, "TX_그래프_LED"=w539, "TX_그래프2_LED"=w539, "TX_그래프3_LED"=TRUE, "TX_그래프4_LED"=w539, "TX_그래프5_LED"=w539, "유속데이터흐름표_10분"=w522, "유속데이터흐름표_30분"=w521, "유속데이터흐름표_50분"=w520) -> (w541:T7)
          }
          frame 4 {
            w578 = FALSE
            n166 = Unbundle By Name(w564) -> ("유속데이터흐름표_10분"=w577:string[][])
            n167 = Unbundle By Name(w564) -> ("유속데이터흐름표_30분"=w575:string[][])
            n168 = Unbundle By Name(w564) -> ("유속데이터흐름표_50분"=w576:string[][])
            n169 = Number To Decimal String(number=w563) -> (decimal integer string=w571:string)  [unwired: 1 in]
            n170 = Replace Array Subset(array=w577, new element=w571, index (row)=1 ("인덱스 (행)"), index (col)=3 ("비활성화된 인덱스 (열)")) -> (w572:string[][])
            n171 = Replace Array Subset(array=w575, new element=w571, index (row)=1 ("인덱스 (행)"), index (col)=3 ("비활성화된 인덱스 (열)")) -> (w573:string[][])
            n172 = Replace Array Subset(array=w576, new element=w571, index (row)=1 ("인덱스 (행)"), index (col)=3 ("비활성화된 인덱스 (열)")) -> (w574:string[][])
            n173 = case shown="10..15" w558 {
              tunnel: [0 13 33 53] -> w562
              tunnel: w572 -> [_ w587 _ _]
              tunnel: w573 -> [_ _ w590 _]
              tunnel: w574 -> [_ _ _ w593]
              tunnel: [w583 w587 w591 w595] -> w561
              tunnel: [w582 w586 w590 w594] -> w560
              tunnel: [w581 w585 w589 w593] -> w559
              tunnel: w575 -> [w582 w586 _ w594]
              tunnel: w576 -> [w581 w585 w589 _]
              tunnel: w577 -> [w583 _ w591 w595]
              frame 0, Default {
              }
              frame 10..15 {
              }
              frame 30..35 {
              }
              frame 50..55 {
              }
            }
            n174 = Bundle By Name(cluster=w564, "TX_그래프_LED"=w578, "TX_그래프2_LED"=w578, "TX_그래프3_LED"=w578, "TX_그래프4_LED"=TRUE, "TX_그래프5_LED"=w578, "유속데이터흐름표_10분"=w561, "유속데이터흐름표_30분"=w560, "유속데이터흐름표_50분"=w559) -> (w580:T7)
          }
          frame 5 {
            w617 = FALSE
            n175 = Unbundle By Name(w601) -> ("유속데이터흐름표_10분"=w616:string[][])
            n176 = Unbundle By Name(w601) -> ("유속데이터흐름표_30분"=w614:string[][])
            n177 = Unbundle By Name(w601) -> ("유속데이터흐름표_50분"=w615:string[][])
            n178 = Number To Decimal String(number=w602) -> (decimal integer string=w610:string)  [unwired: 1 in]
            n179 = Replace Array Subset(array=w616, new element=w610, index (row)=1 ("인덱스 (행)"), index (col)=4 ("비활성화된 인덱스 (열)")) -> (w611:string[][])
            n180 = Replace Array Subset(array=w614, new element=w610, index (row)=1 ("인덱스 (행)"), index (col)=4 ("비활성화된 인덱스 (열)")) -> (w612:string[][])
            n181 = Replace Array Subset(array=w615, new element=w610, index (row)=1 ("인덱스 (행)"), index (col)=4 ("비활성화된 인덱스 (열)")) -> (w613:string[][])
            n182 = case shown="0, 기본" w597 {
              tunnel: [0 14 34 54] -> w603
              tunnel: w611 -> [_ w626 _ _]
              tunnel: w612 -> [_ _ w629 _]
              tunnel: w613 -> [_ _ _ w632]
              tunnel: [w622 w626 w630 w634] -> w600
              tunnel: [w621 w625 w629 w633] -> w599
              tunnel: [w620 w624 w628 w632] -> w598
              tunnel: w614 -> [w621 w625 _ w633]
              tunnel: w615 -> [w620 w624 w628 _]
              tunnel: w616 -> [w622 _ w630 w634]
              frame 0, Default {
              }
              frame 10..15 {
              }
              frame 30..35 {
              }
              frame 50..55 {
              }
            }
            n183 = Bundle By Name(cluster=w601, "TX_그래프_LED"=w617, "TX_그래프2_LED"=w617, "TX_그래프3_LED"=w617, "TX_그래프4_LED"=w617, "TX_그래프5_LED"=TRUE, "유속데이터흐름표_10분"=w600, "유속데이터흐름표_30분"=w599, "유속데이터흐름표_50분"=w598) -> (w619:T7)
          }
        }
        n184 = Concatenate Strings("_Q_" ("시간 포맷 문자열 (%c)"), w459) -> (w456:string)
        n185 = Concatenate Strings("_Order : " ("시간 포맷 문자열 (%c)"), w458) -> (w455:string)
        n186 = Array Subset(array=w441, index (row)=0 ("인덱스"), length (row)=7 ("길이"), index (col)=1 ("인덱스"), length (col)=1 ("길이")) -> (w434:string[][])
        n187 = Format Date/Time String(time format string (%c)="%Y_%m_%d_%H_%M_" ("시간 포맷 문자열 (%c)")) -> (date/time string=w453:string)  [unwired: 2 in]
        n188 = Array Subset(array=w434, index (row)=2 ("인덱스"), length (row)=2 ("길이")) -> (w439:string[][])  [unwired: 2 in]
        n189 = Bundle(w466, w465) -> (→"Station_2":cluster{dbl[], i32[]})  [unwired: 1 in]
        n190 = for {
          tunnel: w439 -> [w637] mode=indexing
          shift-right: [w636] -> w426
          shift-left: string[] [] -> [w638]
          n191 = Build Array (concatenate)(w638, w637) -> (w636:string[])
        }
        n192 = Concatenate Strings(w452, w453, w429, "_Station_" ("시간 포맷 문자열 (%c)"), w428, "_Station : " ("시간 포맷 문자열 (%c)"), w427, w456, w455, "\r") -> (w451:string)
        n193 = Number To Decimal String(number=w422) -> (decimal integer string=w430:string)  [unwired: 1 in]
        n194 = Format Date/Time String(time format string (%c)="%Y_%m_%d_%H_" ("시간 포맷 문자열 (%c)")) -> (date/time string=w431:string)  [unwired: 2 in]
        n195 = Concatenate Strings(w431, w430) -> (→"Station_2_수신시작시간":string)
        n196 = Bundle By Name(cluster=w446, "로그기록"=w451, "RX_그래프_LED"=w419, "RX_그래프2_LED"=TRUE, "RX_그래프3_LED"=w419, "RX_그래프4_LED"=w419, "RX_그래프5_LED"=w419) -> (w449:T6)
        n197 = Build Array (concatenate)(w431, w430, w429, w428, w427, w426) -> (w425:string[])
        n198 = call "Save_teplete(Subvi).vi"("숫자형"=2, "배열"=w425) -> ()  [unwired: 10 in]
      }
      frame 3 {
        w675 = FALSE
        # "※2차원 벡터 -> 1차원 벡터"
        n199 = Format Date/Time String(time format string (%c)="%M" ("시간 포맷 문자열 (%c)")) -> (date/time string=w648:string)  [unwired: 2 in]
        n200 = Subtract(x=w651, y=2000) -> (x-y=w698:i32)
        n201 = call "Save_Log_File(Subvi).vi"("TX_Station"=w652, "RX_Station"=w679, "1D data"=w695) -> ()  [unwired: 7 in, 1 out]
        n202 = property on="Station_현황_TRX_Controller" class="MCListbox (엄격한)"() -> ("ItemNames"=w672:string[][])  [unwired: 2 in, 2 out]
        n203 = for {
          N: 4001 -> [_]
          tunnel: w698 -> [w875]
          shift-right: [w870] -> w696
          shift-left: dbl[] [] -> [w872]
          i -> [w869]
          n204 = Add(x=w875, y=w869) -> (x+y=w874:i32)
          n205 = Divide(x=w874, y=110000) -> (x/y=w871:dbl)
          n206 = Build Array (concatenate)(w872, w871) -> (w870:dbl[])
        }
        n207 = Decimal String To Number(string=w648) -> (number=w646:i32)  [unwired: 2 in, 1 out]
        n208 = Unbundle By Name(w680) -> ("로그기록"=w683:string)
        n209 = Number To Decimal String(number=w652) -> (decimal integer string=w659:string)  [unwired: 1 in]
        n210 = Number To Decimal String(number=w679) -> (decimal integer string=w654:string)  [unwired: 1 in]
        n211 = Number To Decimal String(number=w651) -> (decimal integer string=w657:string)  [unwired: 1 in]
        n212 = Number To Decimal String(number=w678) -> (decimal integer string=w690:string)  [unwired: 1 in]
        n213 = Number To Decimal String(number=w677) -> (decimal integer string=w689:string)  [unwired: 1 in]
        n214 = case shown="5" w652 {
          tunnel: w653 -> [w704 w709 w749 w784 w794 w831]
          tunnel: [w703 w725 w764 w787 w810 w849] -> w649
          tunnel: [0 w711 w748 0 w792 w833] -> w650
          tunnel: w651 -> [_ w710 w750 _ w793 w832]
          tunnel: w646 -> [_ w705 w744 _ w788 w827]
          frame 0, Default {
            w702 = FALSE
            n215 = Bundle By Name(cluster=w704, "TX_그래프_LED"=w702, "TX_그래프2_LED"=w702, "TX_그래프3_LED"=w702, "TX_그래프4_LED"=w702, "TX_그래프5_LED"=w702) -> (w703:T7)
          }
          frame 1 {
            w726 = FALSE
            n216 = Unbundle By Name(w709) -> ("유속데이터흐름표_10분"=w712:string[][])
            n217 = Unbundle By Name(w709) -> ("유속데이터흐름표_30분"=w714:string[][])
            n218 = Unbundle By Name(w709) -> ("유속데이터흐름표_50분"=w713:string[][])
            n219 = Number To Decimal String(number=w710) -> (decimal integer string=w718:string)  [unwired: 1 in]
            n220 = Replace Array Subset(array=w712, new element=w718, index (row)=2 ("인덱스 (행)"), index (col)=0 ("비활성화된 인덱스 (열)")) -> (w717:string[][])
            n221 = Replace Array Subset(array=w714, new element=w718, index (row)=2 ("인덱스 (행)"), index (col)=0 ("비활성화된 인덱스 (열)")) -> (w716:string[][])
            n222 = Replace Array Subset(array=w713, new element=w718, index (row)=2 ("인덱스 (행)"), index (col)=0 ("비활성화된 인덱스 (열)")) -> (w715:string[][])
            n223 = case shown="10..15" w705 {
              tunnel: [0 10 30 50] -> w711
              tunnel: w717 -> [_ w734 _ _]
              tunnel: w716 -> [_ _ w737 _]
              tunnel: w715 -> [_ _ _ w740]
              tunnel: [w730 w734 w738 w742] -> w708
              tunnel: [w729 w733 w737 w741] -> w707
              tunnel: [w728 w732 w736 w740] -> w706
              tunnel: w714 -> [w729 w733 _ w741]
              tunnel: w713 -> [w728 w732 w736 _]
              tunnel: w712 -> [w730 _ w738 w742]
              frame 0, Default {
              }
              frame 10..15 {
              }
              frame 30..35 {
              }
              frame 50..55 {
              }
            }
            n224 = Bundle By Name(cluster=w709, "TX_그래프_LED"=TRUE, "TX_그래프2_LED"=w726, "TX_그래프3_LED"=w726, "TX_그래프4_LED"=w726, "TX_그래프5_LED"=w726, "유속데이터흐름표_10분"=w708, "유속데이터흐름표_30분"=w707, "유속데이터흐름표_50분"=w706) -> (w725:T7)
          }
          frame 2 {
            w765 = FALSE
            n225 = Unbundle By Name(w749) -> ("유속데이터흐름표_10분"=w751:string[][])
            n226 = Unbundle By Name(w749) -> ("유속데이터흐름표_30분"=w753:string[][])
            n227 = Unbundle By Name(w749) -> ("유속데이터흐름표_50분"=w752:string[][])
            n228 = Number To Decimal String(number=w750) -> (decimal integer string=w757:string)  [unwired: 1 in]
            n229 = Replace Array Subset(array=w751, new element=w757, index (row)=2 ("인덱스 (행)"), index (col)=1 ("비활성화된 인덱스 (열)")) -> (w756:string[][])
            n230 = Replace Array Subset(array=w753, new element=w757, index (row)=2 ("인덱스 (행)"), index (col)=1 ("비활성화된 인덱스 (열)")) -> (w755:string[][])
            n231 = Replace Array Subset(array=w752, new element=w757, index (row)=2 ("인덱스 (행)"), index (col)=1 ("비활성화된 인덱스 (열)")) -> (w754:string[][])
            n232 = case shown="50..55" w744 {
              tunnel: [0 11 31 51] -> w748
              tunnel: w756 -> [_ w773 _ _]
              tunnel: w755 -> [_ _ w776 _]
              tunnel: w754 -> [_ _ _ w779]
              tunnel: [w769 w773 w777 w781] -> w747
              tunnel: [w768 w772 w776 w780] -> w746
              tunnel: [w767 w771 w775 w779] -> w745
              tunnel: w753 -> [w768 w772 _ w780]
              tunnel: w752 -> [w767 w771 w775 _]
              tunnel: w751 -> [w769 _ w777 w781]
              frame 0, Default {
              }
              frame 10..15 {
              }
              frame 30..35 {
              }
              frame 50..55 {
              }
            }
            n233 = Bundle By Name(cluster=w749, "TX_그래프_LED"=w765, "TX_그래프2_LED"=TRUE, "TX_그래프3_LED"=w765, "TX_그래프4_LED"=w765, "TX_그래프5_LED"=w765, "유속데이터흐름표_10분"=w747, "유속데이터흐름표_30분"=w746, "유속데이터흐름표_50분"=w745) -> (w764:T7)
          }
          frame 3 {
            w785 = FALSE
            n234 = Bundle By Name(cluster=w784, "TX_그래프_LED"=w785, "TX_그래프2_LED"=w785, "TX_그래프3_LED"=TRUE, "TX_그래프4_LED"=w785, "TX_그래프5_LED"=w785) -> (w787:T7)
          }
          frame 4 {
            w808 = FALSE
            n235 = Unbundle By Name(w794) -> ("유속데이터흐름표_10분"=w807:string[][])
            n236 = Unbundle By Name(w794) -> ("유속데이터흐름표_30분"=w805:string[][])
            n237 = Unbundle By Name(w794) -> ("유속데이터흐름표_50분"=w806:string[][])
            n238 = Number To Decimal String(number=w793) -> (decimal integer string=w801:string)  [unwired: 1 in]
            n239 = Replace Array Subset(array=w807, new element=w801, index (row)=2 ("인덱스 (행)"), index (col)=3 ("비활성화된 인덱스 (열)")) -> (w802:string[][])
            n240 = Replace Array Subset(array=w805, new element=w801, index (row)=2 ("인덱스 (행)"), index (col)=3 ("비활성화된 인덱스 (열)")) -> (w803:string[][])
            n241 = Replace Array Subset(array=w806, new element=w801, index (row)=2 ("인덱스 (행)"), index (col)=3 ("비활성화된 인덱스 (열)")) -> (w804:string[][])
            n242 = case shown="10..15" w788 {
              tunnel: [0 13 33 53] -> w792
              tunnel: w802 -> [_ w817 _ _]
              tunnel: w803 -> [_ _ w820 _]
              tunnel: w804 -> [_ _ _ w823]
              tunnel: [w813 w817 w821 w825] -> w791
              tunnel: [w812 w816 w820 w824] -> w790
              tunnel: [w811 w815 w819 w823] -> w789
              tunnel: w805 -> [w812 w816 _ w824]
              tunnel: w806 -> [w811 w815 w819 _]
              tunnel: w807 -> [w813 _ w821 w825]
              frame 0, Default {
              }
              frame 10..15 {
              }
              frame 30..35 {
              }
              frame 50..55 {
              }
            }
            n243 = Bundle By Name(cluster=w794, "TX_그래프_LED"=w808, "TX_그래프2_LED"=w808, "TX_그래프3_LED"=w808, "TX_그래프4_LED"=TRUE, "TX_그래프5_LED"=w808, "유속데이터흐름표_10분"=w791, "유속데이터흐름표_30분"=w790, "유속데이터흐름표_50분"=w789) -> (w810:T7)
          }
          frame 5 {
            w847 = FALSE
            n244 = Unbundle By Name(w831) -> ("유속데이터흐름표_10분"=w846:string[][])
            n245 = Unbundle By Name(w831) -> ("유속데이터흐름표_30분"=w844:string[][])
            n246 = Unbundle By Name(w831) -> ("유속데이터흐름표_50분"=w845:string[][])
            n247 = Number To Decimal String(number=w832) -> (decimal integer string=w840:string)  [unwired: 1 in]
            n248 = Replace Array Subset(array=w846, new element=w840, index (row)=2 ("인덱스 (행)"), index (col)=4 ("비활성화된 인덱스 (열)")) -> (w841:string[][])
            n249 = Replace Array Subset(array=w844, new element=w840, index (row)=2 ("인덱스 (행)"), index (col)=4 ("비활성화된 인덱스 (열)")) -> (w842:string[][])
            n250 = Replace Array Subset(array=w845, new element=w840, index (row)=2 ("인덱스 (행)"), index (col)=4 ("비활성화된 인덱스 (열)")) -> (w843:string[][])
            n251 = case shown="0, 기본" w827 {
              tunnel: [0 14 34 54] -> w833
              tunnel: w841 -> [_ w856 _ _]
              tunnel: w842 -> [_ _ w859 _]
              tunnel: w843 -> [_ _ _ w862]
              tunnel: [w852 w856 w860 w864] -> w830
              tunnel: [w851 w855 w859 w863] -> w829
              tunnel: [w850 w854 w858 w862] -> w828
              tunnel: w844 -> [w851 w855 _ w863]
              tunnel: w845 -> [w850 w854 w858 _]
              tunnel: w846 -> [w852 _ w860 w864]
              frame 0, Default {
              }
              frame 10..15 {
              }
              frame 30..35 {
              }
              frame 50..55 {
              }
            }
            n252 = Bundle By Name(cluster=w831, "TX_그래프_LED"=w847, "TX_그래프2_LED"=w847, "TX_그래프3_LED"=w847, "TX_그래프4_LED"=w847, "TX_그래프5_LED"=TRUE, "유속데이터흐름표_10분"=w830, "유속데이터흐름표_30분"=w829, "유속데이터흐름표_50분"=w828) -> (w849:T7)
          }
        }
        n253 = Concatenate Strings("_Q_" ("시간 포맷 문자열 (%c)"), w690) -> (w687:string)
        n254 = Concatenate Strings("_Order : " ("시간 포맷 문자열 (%c)"), w689) -> (w686:string)
        n255 = Array Subset(array=w672, index (row)=0 ("인덱스"), length (row)=7 ("길이"), index (col)=2 ("인덱스"), length (col)=1 ("길이")) -> (w665:string[][])
        n256 = Format Date/Time String(time format string (%c)="%Y_%m_%d_%H_%M_" ("시간 포맷 문자열 (%c)")) -> (date/time string=w684:string)  [unwired: 2 in]
        n257 = Array Subset(array=w665, index (row)=2 ("인덱스"), length (row)=2 ("길이")) -> (w670:string[][])  [unwired: 2 in]
        n258 = Bundle(w696, w695) -> (→"Station_3":cluster{dbl[], i32[]})  [unwired: 1 in]
        n259 = for {
          tunnel: w670 -> [w867] mode=indexing
          shift-right: [w866] -> w656
          shift-left: string[] [] -> [w868]
          n260 = Build Array (concatenate)(w868, w867) -> (w866:string[])
        }
        "배열" <- w656
        n261 = Concatenate Strings(w683, w684, w659, "_Station_" ("시간 포맷 문자열 (%c)"), w654, "_Station : " ("시간 포맷 문자열 (%c)"), w657, w687, w686, "\r") -> (w682:string)
        n262 = Number To Decimal String(number=w650) -> (decimal integer string=w660:string)  [unwired: 1 in]
        n263 = Format Date/Time String(time format string (%c)="%Y_%m_%d_%H_" ("시간 포맷 문자열 (%c)")) -> (date/time string=w661:string)  [unwired: 2 in]
        n264 = Concatenate Strings(w661, w660) -> (→"Station_3_수신시작시간":string)
        n265 = Bundle By Name(cluster=w680, "로그기록"=w682, "RX_그래프_LED"=w675, "RX_그래프2_LED"=w675, "RX_그래프3_LED"=TRUE, "RX_그래프4_LED"=w675, "RX_그래프5_LED"=w675) -> (w681:T6)
        n266 = Build Array (concatenate)(w661, w660, w659, w654, w657, w656) -> (w655:string[])
        n267 = call "Save_teplete(Subvi).vi"("숫자형"=2, "배열"=w655) -> ()  [unwired: 10 in]
      }
      frame 4 {
        w904 = FALSE
        # "※2차원 벡터 -> 1차원 벡터"
        n268 = Format Date/Time String(time format string (%c)="%M" ("시간 포맷 문자열 (%c)")) -> (date/time string=w878:string)  [unwired: 2 in]
        n269 = Subtract(x=w879, y=2000) -> (x-y=w928:i32)
        n270 = Decimal String To Number(string=w878) -> (number=w876:i32)  [unwired: 2 in, 1 out]
        n271 = call "Save_Log_File(Subvi).vi"("TX_Station"=w880, "RX_Station"=w908, "1D data"=w925) -> ()  [unwired: 7 in, 1 out]
        n272 = Unbundle By Name(w909) -> ("로그기록"=w912:string)
        n273 = Number To Decimal String(number=w880) -> (decimal integer string=w887:string)  [unwired: 1 in]
        n274 = Number To Decimal String(number=w908) -> (decimal integer string=w886:string)  [unwired: 1 in]
        n275 = Number To Decimal String(number=w879) -> (decimal integer string=w885:string)  [unwired: 1 in]
        n276 = Number To Decimal String(number=w907) -> (decimal integer string=w919:string)  [unwired: 1 in]
        n277 = Number To Decimal String(number=w906) -> (decimal integer string=w918:string)  [unwired: 1 in]
        n278 = for {
          N: 4001 -> [_]
          tunnel: w928 -> [w1105]
          shift-right: [w1100] -> w926
          shift-left: dbl[] [] -> [w1102]
          i -> [w1099]
          n279 = Add(x=w1105, y=w1099) -> (x+y=w1104:i32)
          n280 = Divide(x=w1104, y=110000) -> (x/y=w1101:dbl)
          n281 = Build Array (concatenate)(w1102, w1101) -> (w1100:dbl[])
        }
        n282 = case shown="1" w880 {
          tunnel: [w934 w955 w994 w1035 w1056 w1079] -> w882
          tunnel: [0 w944 w983 w1020 0 w1066] -> w883
          tunnel: w881 -> [w931 w940 w979 w1022 w1053 w1062]
          tunnel: w879 -> [_ w939 w978 w1021 _ w1061]
          tunnel: w876 -> [_ w935 w974 w1013 _ w1057]
          frame 0, Default {
            w933 = FALSE
            n283 = Bundle By Name(cluster=w931, "TX_그래프_LED"=w933, "TX_그래프2_LED"=w933, "TX_그래프3_LED"=w933, "TX_그래프4_LED"=w933, "TX_그래프5_LED"=w933) -> (w934:T7)
          }
          frame 1 {
            w956 = FALSE
            n284 = Unbundle By Name(w940) -> ("유속데이터흐름표_10분"=w938:string[][])
            n285 = Unbundle By Name(w940) -> ("유속데이터흐름표_30분"=w937:string[][])
            n286 = Unbundle By Name(w940) -> ("유속데이터흐름표_50분"=w936:string[][])
            n287 = Number To Decimal String(number=w939) -> (decimal integer string=w948:string)  [unwired: 1 in]
            n288 = Replace Array Subset(array=w938, new element=w948, index (row)=3 ("인덱스 (행)"), index (col)=0 ("비활성화된 인덱스 (열)")) -> (w947:string[][])
            n289 = Replace Array Subset(array=w937, new element=w948, index (row)=3 ("인덱스 (행)"), index (col)=0 ("비활성화된 인덱스 (열)")) -> (w946:string[][])
            n290 = Replace Array Subset(array=w936, new element=w948, index (row)=3 ("인덱스 (행)"), index (col)=0 ("비활성화된 인덱스 (열)")) -> (w945:string[][])
            n291 = case shown="50..55" w935 {
              tunnel: [0 10 30 50] -> w944
              tunnel: w947 -> [_ w964 _ _]
              tunnel: w946 -> [_ _ w968 _]
              tunnel: w945 -> [_ _ _ w972]
              tunnel: [w960 w964 w967 w971] -> w943
              tunnel: [w959 w963 w968 w970] -> w942
              tunnel: [w958 w962 w966 w972] -> w941
              tunnel: w937 -> [w959 w963 _ w970]
              tunnel: w936 -> [w958 w962 w966 _]
              tunnel: w938 -> [w960 _ w967 w971]
              frame 0, Default {
              }
              frame 10..15 {
              }
              frame 30..35 {
              }
              frame 50..55 {
              }
            }
            n292 = Bundle By Name(cluster=w940, "TX_그래프_LED"=TRUE, "TX_그래프2_LED"=w956, "TX_그래프3_LED"=w956, "TX_그래프4_LED"=w956, "TX_그래프5_LED"=w956, "유속데이터흐름표_10분"=w943, "유속데이터흐름표_30분"=w942, "유속데이터흐름표_50분"=w941) -> (w955:T7)
          }
          frame 2 {
            w995 = FALSE
            n293 = Unbundle By Name(w979) -> ("유속데이터흐름표_10분"=w977:string[][])
            n294 = Unbundle By Name(w979) -> ("유속데이터흐름표_30분"=w976:string[][])
            n295 = Unbundle By Name(w979) -> ("유속데이터흐름표_50분"=w975:string[][])
            n296 = Number To Decimal String(number=w978) -> (decimal integer string=w987:string)  [unwired: 1 in]
            n297 = Replace Array Subset(array=w977, new element=w987, index (row)=3 ("인덱스 (행)"), index (col)=1 ("비활성화된 인덱스 (열)")) -> (w986:string[][])
            n298 = Replace Array Subset(array=w976, new element=w987, index (row)=3 ("인덱스 (행)"), index (col)=1 ("비활성화된 인덱스 (열)")) -> (w985:string[][])
            n299 = Replace Array Subset(array=w975, new element=w987, index (row)=3 ("인덱스 (행)"), index (col)=1 ("비활성화된 인덱스 (열)")) -> (w984:string[][])
            n300 = case shown="10..15" w974 {
              tunnel: [0 11 31 51] -> w983
              tunnel: w986 -> [_ w1003 _ _]
              tunnel: w985 -> [_ _ w1007 _]
              tunnel: w984 -> [_ _ _ w1011]
              tunnel: [w999 w1003 w1006 w1010] -> w982
              tunnel: [w998 w1002 w1007 w1009] -> w981
              tunnel: [w997 w1001 w1005 w1011] -> w980
              tunnel: w976 -> [w998 w1002 _ w1009]
              tunnel: w975 -> [w997 w1001 w1005 _]
              tunnel: w977 -> [w999 _ w1006 w1010]
              frame 0, Default {
              }
              frame 10..15 {
              }
              frame 30..35 {
              }
              frame 50..55 {
              }
            }
            n301 = Bundle By Name(cluster=w979, "TX_그래프_LED"=w995, "TX_그래프2_LED"=TRUE, "TX_그래프3_LED"=w995, "TX_그래프4_LED"=w995, "TX_그래프5_LED"=w995, "유속데이터흐름표_10분"=w982, "유속데이터흐름표_30분"=w981, "유속데이터흐름표_50분"=w980) -> (w994:T7)
          }
          frame 3 {
            w1033 = FALSE
            n302 = Unbundle By Name(w1022) -> ("유속데이터흐름표_10분"=w1016:string[][])
            n303 = Unbundle By Name(w1022) -> ("유속데이터흐름표_30분"=w1015:string[][])
            n304 = Unbundle By Name(w1022) -> ("유속데이터흐름표_50분"=w1014:string[][])
            n305 = Number To Decimal String(number=w1021) -> (decimal integer string=w1026:string)  [unwired: 1 in]
            n306 = Replace Array Subset(array=w1016, new element=w1026, index (row)=3 ("인덱스 (행)"), index (col)=2 ("비활성화된 인덱스 (열)")) -> (w1025:string[][])
            n307 = Replace Array Subset(array=w1015, new element=w1026, index (row)=3 ("인덱스 (행)"), index (col)=2 ("비활성화된 인덱스 (열)")) -> (w1024:string[][])
            n308 = Replace Array Subset(array=w1014, new element=w1026, index (row)=3 ("인덱스 (행)"), index (col)=2 ("비활성화된 인덱스 (열)")) -> (w1023:string[][])
            n309 = case shown="10..15" w1013 {
              tunnel: [0 12 32 52] -> w1020
              tunnel: w1025 -> [_ w1042 _ _]
              tunnel: w1024 -> [_ _ w1046 _]
              tunnel: w1023 -> [_ _ _ w1050]
              tunnel: [w1038 w1042 w1045 w1049] -> w1019
              tunnel: [w1037 w1041 w1046 w1048] -> w1018
              tunnel: [w1036 w1040 w1044 w1050] -> w1017
              tunnel: w1015 -> [w1037 w1041 _ w1048]
              tunnel: w1014 -> [w1036 w1040 w1044 _]
              tunnel: w1016 -> [w1038 _ w1045 w1049]
              frame 0, Default {
              }
              frame 10..15 {
              }
              frame 30..35 {
              }
              frame 50..55 {
              }
            }
            n310 = Bundle By Name(cluster=w1022, "TX_그래프_LED"=w1033, "TX_그래프2_LED"=w1033, "TX_그래프3_LED"=TRUE, "TX_그래프4_LED"=w1033, "TX_그래프5_LED"=w1033, "유속데이터흐름표_10분"=w1019, "유속데이터흐름표_30분"=w1018, "유속데이터흐름표_50분"=w1017) -> (w1035:T7)
          }
          frame 4 {
            w1054 = FALSE
            n311 = Bundle By Name(cluster=w1053, "TX_그래프_LED"=w1054, "TX_그래프2_LED"=w1054, "TX_그래프3_LED"=w1054, "TX_그래프4_LED"=TRUE, "TX_그래프5_LED"=w1054) -> (w1056:T7)
          }
          frame 5 {
            w1077 = FALSE
            n312 = Unbundle By Name(w1062) -> ("유속데이터흐름표_10분"=w1060:string[][])
            n313 = Unbundle By Name(w1062) -> ("유속데이터흐름표_30분"=w1059:string[][])
            n314 = Unbundle By Name(w1062) -> ("유속데이터흐름표_50분"=w1058:string[][])
            n315 = Number To Decimal String(number=w1061) -> (decimal integer string=w1073:string)  [unwired: 1 in]
            n316 = Replace Array Subset(array=w1060, new element=w1073, index (row)=3 ("인덱스 (행)"), index (col)=4 ("비활성화된 인덱스 (열)")) -> (w1074:string[][])
            n317 = Replace Array Subset(array=w1059, new element=w1073, index (row)=3 ("인덱스 (행)"), index (col)=4 ("비활성화된 인덱스 (열)")) -> (w1075:string[][])
            n318 = Replace Array Subset(array=w1058, new element=w1073, index (row)=3 ("인덱스 (행)"), index (col)=4 ("비활성화된 인덱스 (열)")) -> (w1076:string[][])
            n319 = case shown="10..15" w1057 {
              tunnel: [0 14 34 54] -> w1066
              tunnel: w1074 -> [_ w1086 _ _]
              tunnel: w1075 -> [_ _ w1090 _]
              tunnel: w1076 -> [_ _ _ w1094]
              tunnel: [w1082 w1086 w1089 w1093] -> w1065
              tunnel: [w1081 w1085 w1090 w1092] -> w1064
              tunnel: [w1080 w1084 w1088 w1094] -> w1063
              tunnel: w1059 -> [w1081 w1085 _ w1092]
              tunnel: w1058 -> [w1080 w1084 w1088 _]
              tunnel: w1060 -> [w1082 _ w1089 w1093]
              frame 0, Default {
              }
              frame 10..15 {
              }
              frame 30..35 {
              }
              frame 50..55 {
              }
            }
            n320 = Bundle By Name(cluster=w1062, "TX_그래프_LED"=w1077, "TX_그래프2_LED"=w1077, "TX_그래프3_LED"=w1077, "TX_그래프4_LED"=w1077, "TX_그래프5_LED"=TRUE, "유속데이터흐름표_10분"=w1065, "유속데이터흐름표_30분"=w1064, "유속데이터흐름표_50분"=w1063) -> (w1079:T7)
          }
        }
        n321 = Concatenate Strings("_Q_" ("시간 포맷 문자열 (%c)"), w919) -> (w916:string)
        n322 = Concatenate Strings("_Order : " ("시간 포맷 문자열 (%c)"), w918) -> (w915:string)
        n323 = Format Date/Time String(time format string (%c)="%Y_%m_%d_%H_%M_" ("시간 포맷 문자열 (%c)")) -> (date/time string=w913:string)  [unwired: 2 in]
        n324 = Bundle(w926, w925) -> (→"Station_4":cluster{dbl[], i32[]})  [unwired: 1 in]
        n325 = Concatenate Strings(w912, w913, w887, "_Station_" ("시간 포맷 문자열 (%c)"), w886, "_Station : " ("시간 포맷 문자열 (%c)"), w885, w916, w915, "\r") -> (w911:string)
        n326 = property on="Station_현황_TRX_Controller" class="MCListbox (엄격한)"() -> ("ItemNames"=w901:string[][])  [unwired: 2 in, 2 out]
        n327 = Array Subset(array=w901, index (row)=0 ("인덱스"), length (row)=7 ("길이"), index (col)=3 ("인덱스"), length (col)=1 ("길이")) -> (w894:string[][])
        n328 = Array Subset(array=w894, index (row)=2 ("인덱스"), length (row)=2 ("길이")) -> (w899:string[][])  [unwired: 2 in]
        n329 = for {
          tunnel: w899 -> [w1097] mode=indexing
          shift-right: [w1096] -> w884
          shift-left: string[] [] -> [w1098]
          n330 = Build Array (concatenate)(w1098, w1097) -> (w1096:string[])
        }
        n331 = Format Date/Time String(time format string (%c)="%Y_%m_%d_%H_" ("시간 포맷 문자열 (%c)")) -> (date/time string=w890:string)  [unwired: 2 in]
        n332 = Number To Decimal String(number=w883) -> (decimal integer string=w889:string)  [unwired: 1 in]
        n333 = Concatenate Strings(w890, w889) -> (→"Station_4_수신시작시간":string)
        n334 = Bundle By Name(cluster=w909, "로그기록"=w911, "RX_그래프_LED"=w904, "RX_그래프2_LED"=w904, "RX_그래프3_LED"=w904, "RX_그래프4_LED"=TRUE, "RX_그래프5_LED"=w904) -> (w910:T6)
        n335 = Build Array (concatenate)(w890, w889, w887, w886, w885, w884) -> (w888:string[])
        n336 = call "Save_teplete(Subvi).vi"("숫자형"=2, "배열"=w888) -> ()  [unwired: 10 in]
      }
      frame 5 {
        w1134 = FALSE
        # "※2차원 벡터 -> 1차원 벡터"
        n337 = Format Date/Time String(time format string (%c)="%M" ("시간 포맷 문자열 (%c)")) -> (date/time string=w1108:string)  [unwired: 2 in]
        n338 = property on="Station_현황_TRX_Controller" class="MCListbox (엄격한)"() -> ("ItemNames"=w1131:string[][])  [unwired: 2 in, 2 out]
        n339 = Subtract(x=w1109, y=2000) -> (x-y=w1158:i32)
        n340 = Decimal String To Number(string=w1108) -> (number=w1106:i32)  [unwired: 2 in, 1 out]
        n341 = call "Save_Log_File(Subvi).vi"("TX_Station"=w1110, "RX_Station"=w1138, "1D data"=w1155) -> ()  [unwired: 7 in, 1 out]
        n342 = for {
          N: 4001 -> [_]
          tunnel: w1158 -> [w1335]
          shift-right: [w1330] -> w1156
          shift-left: dbl[] [] -> [w1332]
          i -> [w1329]
          n343 = Add(x=w1335, y=w1329) -> (x+y=w1334:i32)
          n344 = Divide(x=w1334, y=110000) -> (x/y=w1331:dbl)
          n345 = Build Array (concatenate)(w1332, w1331) -> (w1330:dbl[])
        }
        n346 = Unbundle By Name(w1139) -> ("로그기록"=w1142:string)
        n347 = Number To Decimal String(number=w1110) -> (decimal integer string=w1118:string)  [unwired: 1 in]
        n348 = case shown="1" w1110 {
          tunnel: [w1164 w1185 w1224 w1265 w1304 w1325] -> w1112
          tunnel: [0 w1174 w1213 w1250 w1289 0] -> w1113
          tunnel: w1111 -> [w1161 w1170 w1209 w1252 w1291 w1322]
          tunnel: w1109 -> [_ w1169 w1208 w1251 w1290 _]
          tunnel: w1106 -> [_ w1165 w1204 w1243 w1282 _]
          frame 0, Default {
            w1163 = FALSE
            n349 = Bundle By Name(cluster=w1161, "TX_그래프_LED"=w1163, "TX_그래프2_LED"=w1163, "TX_그래프3_LED"=w1163, "TX_그래프4_LED"=w1163, "TX_그래프5_LED"=w1163) -> (w1164:T7)
          }
          frame 1 {
            w1186 = FALSE
            n350 = Unbundle By Name(w1170) -> ("유속데이터흐름표_10분"=w1168:string[][])
            n351 = Unbundle By Name(w1170) -> ("유속데이터흐름표_30분"=w1167:string[][])
            n352 = Unbundle By Name(w1170) -> ("유속데이터흐름표_50분"=w1166:string[][])
            n353 = Number To Decimal String(number=w1169) -> (decimal integer string=w1178:string)  [unwired: 1 in]
            n354 = Replace Array Subset(array=w1168, new element=w1178, index (row)=4 ("인덱스 (행)"), index (col)=0 ("비활성화된 인덱스 (열)")) -> (w1177:string[][])
            n355 = Replace Array Subset(array=w1167, new element=w1178, index (row)=4 ("인덱스 (행)"), index (col)=0 ("비활성화된 인덱스 (열)")) -> (w1176:string[][])
            n356 = Replace Array Subset(array=w1166, new element=w1178, index (row)=4 ("인덱스 (행)"), index (col)=0 ("비활성화된 인덱스 (열)")) -> (w1175:string[][])
            n357 = case shown="50..55" w1165 {
              tunnel: [0 10 30 50] -> w1174
              tunnel: w1177 -> [_ w1194 _ _]
              tunnel: w1176 -> [_ _ w1198 _]
              tunnel: w1175 -> [_ _ _ w1202]
              tunnel: [w1190 w1194 w1197 w1201] -> w1173
              tunnel: [w1189 w1193 w1198 w1200] -> w1172
              tunnel: [w1188 w1192 w1196 w1202] -> w1171
              tunnel: w1167 -> [w1189 w1193 _ w1200]
              tunnel: w1166 -> [w1188 w1192 w1196 _]
              tunnel: w1168 -> [w1190 _ w1197 w1201]
              frame 0, Default {
              }
              frame 10..15 {
              }
              frame 30..35 {
              }
              frame 50..55 {
              }
            }
            n358 = Bundle By Name(cluster=w1170, "TX_그래프_LED"=TRUE, "TX_그래프2_LED"=w1186, "TX_그래프3_LED"=w1186, "TX_그래프4_LED"=w1186, "TX_그래프5_LED"=w1186, "유속데이터흐름표_10분"=w1173, "유속데이터흐름표_30분"=w1172, "유속데이터흐름표_50분"=w1171) -> (w1185:T7)
          }
          frame 2 {
            w1225 = FALSE
            n359 = Unbundle By Name(w1209) -> ("유속데이터흐름표_10분"=w1207:string[][])
            n360 = Unbundle By Name(w1209) -> ("유속데이터흐름표_30분"=w1206:string[][])
            n361 = Unbundle By Name(w1209) -> ("유속데이터흐름표_50분"=w1205:string[][])
            n362 = Number To Decimal String(number=w1208) -> (decimal integer string=w1217:string)  [unwired: 1 in]
            n363 = Replace Array Subset(array=w1207, new element=w1217, index (row)=4 ("인덱스 (행)"), index (col)=1 ("비활성화된 인덱스 (열)")) -> (w1216:string[][])
            n364 = Replace Array Subset(array=w1206, new element=w1217, index (row)=4 ("인덱스 (행)"), index (col)=1 ("비활성화된 인덱스 (열)")) -> (w1215:string[][])
            n365 = Replace Array Subset(array=w1205, new element=w1217, index (row)=4 ("인덱스 (행)"), index (col)=1 ("비활성화된 인덱스 (열)")) -> (w1214:string[][])
            n366 = case shown="50..55" w1204 {
              tunnel: [0 11 31 51] -> w1213
              tunnel: w1216 -> [_ w1233 _ _]
              tunnel: w1215 -> [_ _ w1237 _]
              tunnel: w1214 -> [_ _ _ w1241]
              tunnel: [w1229 w1233 w1236 w1240] -> w1212
              tunnel: [w1228 w1232 w1237 w1239] -> w1211
              tunnel: [w1227 w1231 w1235 w1241] -> w1210
              tunnel: w1206 -> [w1228 w1232 _ w1239]
              tunnel: w1205 -> [w1227 w1231 w1235 _]
              tunnel: w1207 -> [w1229 _ w1236 w1240]
              frame 0, Default {
              }
              frame 10..15 {
              }
              frame 30..35 {
              }
              frame 50..55 {
              }
            }
            n367 = Bundle By Name(cluster=w1209, "TX_그래프_LED"=w1225, "TX_그래프2_LED"=TRUE, "TX_그래프3_LED"=w1225, "TX_그래프4_LED"=w1225, "TX_그래프5_LED"=w1225, "유속데이터흐름표_10분"=w1212, "유속데이터흐름표_30분"=w1211, "유속데이터흐름표_50분"=w1210) -> (w1224:T7)
          }
          frame 3 {
            w1263 = FALSE
            n368 = Unbundle By Name(w1252) -> ("유속데이터흐름표_10분"=w1246:string[][])
            n369 = Unbundle By Name(w1252) -> ("유속데이터흐름표_30분"=w1245:string[][])
            n370 = Unbundle By Name(w1252) -> ("유속데이터흐름표_50분"=w1244:string[][])
            n371 = Number To Decimal String(number=w1251) -> (decimal integer string=w1256:string)  [unwired: 1 in]
            n372 = Replace Array Subset(array=w1246, new element=w1256, index (row)=4 ("인덱스 (행)"), index (col)=2 ("비활성화된 인덱스 (열)")) -> (w1255:string[][])
            n373 = Replace Array Subset(array=w1245, new element=w1256, index (row)=4 ("인덱스 (행)"), index (col)=2 ("비활성화된 인덱스 (열)")) -> (w1254:string[][])
            n374 = Replace Array Subset(array=w1244, new element=w1256, index (row)=4 ("인덱스 (행)"), index (col)=2 ("비활성화된 인덱스 (열)")) -> (w1253:string[][])
            n375 = case shown="10..15" w1243 {
              tunnel: [0 12 32 52] -> w1250
              tunnel: w1255 -> [_ w1272 _ _]
              tunnel: w1254 -> [_ _ w1276 _]
              tunnel: w1253 -> [_ _ _ w1280]
              tunnel: [w1268 w1272 w1275 w1279] -> w1249
              tunnel: [w1267 w1271 w1276 w1278] -> w1248
              tunnel: [w1266 w1270 w1274 w1280] -> w1247
              tunnel: w1245 -> [w1267 w1271 _ w1278]
              tunnel: w1244 -> [w1266 w1270 w1274 _]
              tunnel: w1246 -> [w1268 _ w1275 w1279]
              frame 0, Default {
              }
              frame 10..15 {
              }
              frame 30..35 {
              }
              frame 50..55 {
              }
            }
            n376 = Bundle By Name(cluster=w1252, "TX_그래프_LED"=w1263, "TX_그래프2_LED"=w1263, "TX_그래프3_LED"=TRUE, "TX_그래프4_LED"=w1263, "TX_그래프5_LED"=w1263, "유속데이터흐름표_10분"=w1249, "유속데이터흐름표_30분"=w1248, "유속데이터흐름표_50분"=w1247) -> (w1265:T7)
          }
          frame 4 {
            w1302 = FALSE
            n377 = Unbundle By Name(w1291) -> ("유속데이터흐름표_10분"=w1285:string[][])
            n378 = Unbundle By Name(w1291) -> ("유속데이터흐름표_30분"=w1284:string[][])
            n379 = Unbundle By Name(w1291) -> ("유속데이터흐름표_50분"=w1283:string[][])
            n380 = Number To Decimal String(number=w1290) -> (decimal integer string=w1295:string)  [unwired: 1 in]
            n381 = Replace Array Subset(array=w1285, new element=w1295, index (row)=4 ("인덱스 (행)"), index (col)=3 ("비활성화된 인덱스 (열)")) -> (w1294:string[][])
            n382 = Replace Array Subset(array=w1284, new element=w1295, index (row)=4 ("인덱스 (행)"), index (col)=3 ("비활성화된 인덱스 (열)")) -> (w1293:string[][])
            n383 = Replace Array Subset(array=w1283, new element=w1295, index (row)=4 ("인덱스 (행)"), index (col)=3 ("비활성화된 인덱스 (열)")) -> (w1292:string[][])
            n384 = case shown="10..15" w1282 {
              tunnel: [0 13 33 53] -> w1289
              tunnel: w1294 -> [_ w1311 _ _]
              tunnel: w1293 -> [_ _ w1315 _]
              tunnel: w1292 -> [_ _ _ w1319]
              tunnel: [w1307 w1311 w1314 w1318] -> w1288
              tunnel: [w1306 w1310 w1315 w1317] -> w1287
              tunnel: [w1305 w1309 w1313 w1319] -> w1286
              tunnel: w1284 -> [w1306 w1310 _ w1317]
              tunnel: w1283 -> [w1305 w1309 w1313 _]
              tunnel: w1285 -> [w1307 _ w1314 w1318]
              frame 0, Default {
              }
              frame 10..15 {
              }
              frame 30..35 {
              }
              frame 50..55 {
              }
            }
            n385 = Bundle By Name(cluster=w1291, "TX_그래프_LED"=w1302, "TX_그래프2_LED"=w1302, "TX_그래프3_LED"=w1302, "TX_그래프4_LED"=TRUE, "TX_그래프5_LED"=w1302, "유속데이터흐름표_10분"=w1288, "유속데이터흐름표_30분"=w1287, "유속데이터흐름표_50분"=w1286) -> (w1304:T7)
          }
          frame 5 {
            w1323 = FALSE
            n386 = Bundle By Name(cluster=w1322, "TX_그래프_LED"=w1323, "TX_그래프2_LED"=w1323, "TX_그래프3_LED"=w1323, "TX_그래프4_LED"=w1323, "TX_그래프5_LED"=TRUE) -> (w1325:T7)
          }
        }
        n387 = Number To Decimal String(number=w1138) -> (decimal integer string=w1117:string)  [unwired: 1 in]
        n388 = Number To Decimal String(number=w1109) -> (decimal integer string=w1116:string)  [unwired: 1 in]
        n389 = Number To Decimal String(number=w1137) -> (decimal integer string=w1149:string)  [unwired: 1 in]
        n390 = Number To Decimal String(number=w1136) -> (decimal integer string=w1148:string)  [unwired: 1 in]
        n391 = Concatenate Strings("_Q_" ("시간 포맷 문자열 (%c)"), w1149) -> (w1146:string)
        n392 = Concatenate Strings("_Order : " ("시간 포맷 문자열 (%c)"), w1148) -> (w1145:string)
        n393 = Array Subset(array=w1131, index (row)=0 ("인덱스"), length (row)=7 ("길이"), index (col)=4 ("인덱스"), length (col)=1 ("길이")) -> (w1129:string[][])
        n394 = Format Date/Time String(time format string (%c)="%Y_%m_%d_%H_%M_" ("시간 포맷 문자열 (%c)")) -> (date/time string=w1143:string)  [unwired: 2 in]
        n395 = Array Subset(array=w1129, index (row)=2 ("인덱스"), length (row)=2 ("길이")) -> (w1130:string[][])  [unwired: 2 in]
        n396 = Bundle(w1156, w1155) -> (→"Station_5":cluster{dbl[], i32[]})  [unwired: 1 in]
        n397 = for {
          tunnel: w1130 -> [w1327] mode=indexing
          shift-right: [w1326] -> w1115
          shift-left: string[] [] -> [w1328]
          n398 = Build Array (concatenate)(w1328, w1327) -> (w1326:string[])
        }
        n399 = Concatenate Strings(w1142, w1143, w1118, "_Station_" ("시간 포맷 문자열 (%c)"), w1117, "_Station : " ("시간 포맷 문자열 (%c)"), w1116, w1146, w1145, "\r") -> (w1141:string)
        n400 = Format Date/Time String(time format string (%c)="%Y_%m_%d_%H_" ("시간 포맷 문자열 (%c)")) -> (date/time string=w1120:string)  [unwired: 2 in]
        n401 = Number To Decimal String(number=w1113) -> (decimal integer string=w1119:string)  [unwired: 1 in]
        n402 = Concatenate Strings(w1120, w1119) -> (→"Station_5_수신시작시간":string)
        n403 = Bundle By Name(cluster=w1139, "로그기록"=w1141, "RX_그래프_LED"=w1134, "RX_그래프2_LED"=w1134, "RX_그래프3_LED"=w1134, "RX_그래프4_LED"=w1134, "RX_그래프5_LED"=TRUE) -> (w1140:T6)
        n404 = Build Array (concatenate)(w1120, w1119, w1118, w1117, w1116, w1115) -> (w1114:string[])
        n405 = call "Save_teplete(Subvi).vi"("숫자형"=2, "배열"=w1114) -> ()  [unwired: 10 in]
      }
    }
    n406 = Unbundle By Name(w134) -> ("TX_그래프_LED"=→"TX_LED_1":bool, "TX_그래프2_LED"=→"TX_LED_2":bool, "TX_그래프3_LED"=→"TX_LED_3":bool, "TX_그래프4_LED"=→"TX_LED_4":bool, "TX_그래프5_LED"=→"TX_LED_5":bool, "유속데이터흐름표_10분"=w123:string[][], "유속데이터흐름표_30분"=w122:string[][], "유속데이터흐름표_50분"=w121:string[][])
    n407 = Unbundle By Name(w129) -> ("로그기록"=→"데이터 통계 현황_결과창":string, "RX_그래프_LED"=→"RX_LED_1":bool, "RX_그래프2_LED"=→"RX_LED_2":bool, "RX_그래프3_LED"=→"RX_LED_3":bool, "RX_그래프4_LED"=→"RX_LED_4":bool, "RX_그래프5_LED"=→"RX_LED_5":bool)
    n408 = property on="유속 데이터 흐름표_10분" class="MCListbox (엄격한)"("ItemNames"=w123) -> ()  [unwired: 2 in, 2 out]
    n409 = property on="유속 데이터 흐름표_30분" class="MCListbox (엄격한)"("ItemNames"=w122) -> ()  [unwired: 2 in, 2 out]
    n410 = property on="유속 데이터 흐름표_50분" class="MCListbox (엄격한)"("ItemNames"=w121) -> ()  [unwired: 2 in, 2 out]
  }
  n411 = while {
    tunnel: w7 -> [w1358]
    tunnel: w6 -> [w1357]
    tunnel: w23 -> [w1354]
    tunnel: w22 -> [w1353]
    shift-right: [w1346] -> _
    shift-left: string[][] [["", "", "", "", "", ""], ["", "", "", "", "", ""], ["", "", "", "", "", ""], ["", "", "", "", "", ""], ["", "", "", "", "", ""], ["", "", "", "", "", ""], ["", "", "", "", "", ""], ["", "", "", "", "", "0"], ["", "", "", "", "", ""], ["", "", "", "", "", ""], ["", "", "", "", "", ""], ["", "", "", "", "", ""], ["", "", "", "", "", ""]] -> [w1347]
    tunnel: [errorcluster {"status"=FALSE, "code"=0, "source"=""} ("에러 상수")] -> w15
    stop <- w1355 stop-if-true
    # "Number 데이터 분리 후 리스트 박스 열에 데이터 대체"
    # "7 index: Number"
    # "Queue2: BDDATA 처리 LOOP"
    n412 = Dequeue Element(queue=w1358, error in (no error)=w1357) -> (queue out=w1352:refnum<queue>, element=w1356:T9, error out=w1351:errorcluster)  [unwired: 1 in, 1 out]
    n413 = Dequeue Element(queue=w1354, error in (no error)=w1353) -> (element=w1348:string[])  [unwired: 1 in, 3 out]
    n414 = case shown="\"Mqtt_Subscribe\"" w1356 {
      tunnel: [_ _ TRUE] -> w1355
      tunnel: w1352 -> [_ w1396 w1401]
      tunnel: w1351 -> [_ w1395 w1400]
      frame "초기화", Default {
      }
      frame "Mqtt_Subscribe" {
        n415 = Enqueue Element(queue=w1396, element=Brain_Loop_CTL."Mqtt_Subscribe", error in (no error)=w1395) -> ()  [unwired: 1 in, 3 out]
      }
      frame "정지" {
        n416 = Flush Queue(queue=w1401, error in (no error)=w1400) -> (queue out=w1399:refnum<queue>, error out=w1398:errorcluster)  [unwired: 1 out]
        n417 = Enqueue Element(queue=w1399, element=Brain_Loop_CTL."정지", error in (no error)=w1398) -> ()  [unwired: 1 in, 3 out]
      }
    }
    n418 = Index Array(array=w1348, index=7 ("인덱스")) -> (element=w1349:string)
    n419 = case shown="\"1\"" w1349 {
      tunnel: w1348 -> [_ w1363 w1370 w1377 w1384 w1391]
      tunnel: w1347 -> [w1359 w1366 w1373 w1380 w1387 w1394]
      tunnel: [w1359 w1364 w1371 w1378 w1385 w1392] -> w1346
      frame "거짓", Default {
      }
      frame "1" {
        # "Number 데이터 분리 후 리스트 박스 열에 데이처 대체"
        n420 = Array Subset(array=w1363, index=0 ("차원 크기"), length=7 ("차원 크기")) -> (w1360:string[])
        n421 = Replace Array Subset(array=w1366, new element=w1360, index (col)=0 ("비활성화된 인덱스 (열)")) -> (w1364:string[][])  [unwired: 1 in]
        n422 = property on="Station_현황_TRX_Controller" class="MCListbox (엄격한)"("ItemNames"=w1364) -> ()  [unwired: 2 in, 2 out]
      }
      frame "2" {
        n423 = Array Subset(array=w1370, index=0 ("차원 크기"), length=7 ("차원 크기")) -> (w1367:string[])
        n424 = Replace Array Subset(array=w1373, new element=w1367, index (col)=1 ("비활성화된 인덱스 (열)")) -> (w1371:string[][])  [unwired: 1 in]
        n425 = property on="Station_현황_TRX_Controller" class="MCListbox (엄격한)"("ItemNames"=w1371) -> ()  [unwired: 2 in, 2 out]
      }
      frame "3" {
        n426 = Array Subset(array=w1377, index=0 ("차원 크기"), length=7 ("차원 크기")) -> (w1374:string[])
        n427 = Replace Array Subset(array=w1380, new element=w1374, index (col)=2 ("비활성화된 인덱스 (열)")) -> (w1378:string[][])  [unwired: 1 in]
        n428 = property on="Station_현황_TRX_Controller" class="MCListbox (엄격한)"("ItemNames"=w1378) -> ()  [unwired: 2 in, 2 out]
      }
      frame "4" {
        n429 = Array Subset(array=w1384, index=0 ("차원 크기"), length=7 ("차원 크기")) -> (w1381:string[])
        n430 = Replace Array Subset(array=w1387, new element=w1381, index (col)=3 ("비활성화된 인덱스 (열)")) -> (w1385:string[][])  [unwired: 1 in]
        n431 = property on="Station_현황_TRX_Controller" class="MCListbox (엄격한)"("ItemNames"=w1385) -> ()  [unwired: 2 in, 2 out]
      }
      frame "5" {
        n432 = Array Subset(array=w1391, index=0 ("차원 크기"), length=7 ("차원 크기")) -> (w1388:string[])
        n433 = Replace Array Subset(array=w1394, new element=w1388, index (col)=4 ("비활성화된 인덱스 (열)")) -> (w1392:string[][])  [unwired: 1 in]
        n434 = property on="Station_현황_TRX_Controller" class="MCListbox (엄격한)"("ItemNames"=w1392) -> ()  [unwired: 2 in, 2 out]
      }
    }
  }
  n435 = while {
    tunnel: w7 -> [w1440]
    tunnel: w6 -> [w1439]
    shift-right: [w1431] -> _
    shift-left: T5 {"Water_Velocity_1_3"=0.0, "Water_Velocity_1_2"=0.0, "Water_Velocity_1_4"=0.0, "Water_Velocity_1_5"=0.0, "Water_Velocity_2_3"=0.0, "Water_Velocity_2_4"=0.0, "Water_Velocity_2_5"=0.0, "Water_Velocity_3_4"=0.0, "Water_Velocity_3_5"=0.0, "Water_Velocity_4_5"=0.0, "Averange_Soundspeed_1_2"=0.0, "Averange_Soundspeed_1_3"=0.0, "Averange_Soundspeed_1_4"=0.0, "Averange_Soundspeed_1_5"=0.0, "Averange_Soundspeed_2_3"=0.0, "Averange_Soundspeed_2_4"=0.0, "Averange_Soundspeed_2_5"=0.0, "Averange_Soundspeed_3_4"=0.0, "Averange_Soundspeed_3_5"=0.0, "Averange_Soundspeed_4_5"=0.0} -> [w1410]
    tunnel: [errorcluster {"status"=FALSE, "code"=0, "source"=""} ("에러 상수")] -> w3
    stop <- w1438 stop-if-true
    n436 = local read "현재 날짜"() -> (w1406:string)
    n437 = Dequeue Element(queue=w1440, error in (no error)=w1439) -> (queue out=w1442:refnum<queue>, element=w1441:T9, error out=w1443:errorcluster)  [unwired: 1 in, 1 out]
    n438 = Format Date/Time String(time format string (%c)="%M" ("시간 포맷 문자열 (%c)")) -> (date/time string=w1437:string)  [unwired: 2 in]
    n439 = Format Date/Time String(time format string (%c)="%S" ("시간 포맷 문자열 (%c)")) -> (date/time string=w1434:string)  [unwired: 2 in]
    n440 = Format Date/Time String(time format string (%c)="%d" ("시간 포맷 문자열 (%c)")) -> (date/time string=w1407:string)  [unwired: 2 in]
    n441 = Decimal String To Number(string=w1437) -> (number=w1433:i32)  [unwired: 2 in, 1 out]
    n442 = case shown="\"Mqtt_Subscribe\"" w1441 {
      tunnel: [_ _ TRUE] -> w1438
      tunnel: w1442 -> [_ w1908 w1913]
      tunnel: w1443 -> [_ w1907 w1912]
      frame "초기화", Default {
      }
      frame "Mqtt_Subscribe" {
        n443 = Enqueue Element(queue=w1908, element=Brain_Loop_CTL."Mqtt_Subscribe", error in (no error)=w1907) -> ()  [unwired: 1 in, 3 out]
      }
      frame "정지" {
        n444 = Flush Queue(queue=w1913, error in (no error)=w1912) -> (queue out=w1911:refnum<queue>, error out=w1910:errorcluster)  [unwired: 1 out]
        n445 = Enqueue Element(queue=w1911, element=Brain_Loop_CTL."정지", error in (no error)=w1910) -> ()  [unwired: 1 in, 3 out]
      }
    }
    n446 = Decimal String To Number(string=w1434) -> (number=w1432:i32)  [unwired: 2 in, 1 out]
    n447 = Equal?(x=w1407, y=w1406) -> (x = y?=w1405:bool)
    n448 = case shown="16" w1433 {
      tunnel: w1432 -> [_ w1642 w1731 w1820]
      tunnel: w1410 -> [w1639 w1641 w1730 w1819]
      tunnel: [w1639 w1640 w1729 w1818] -> w1431
      frame 0, Default {
      }
      frame 16 {
        n449 = case shown="3" w1642 {
          tunnel: w1641 -> [w1643 w1725]
          tunnel: [w1643 w1724] -> w1640
          frame 0, Default {
          }
          frame 3 {
            n450 = property on="유속 데이터 흐름표_10분" class="MCListbox (엄격한)"() -> ("ItemNames"=w1727:string[][])  [unwired: 2 in, 2 out]
            n451 = Wait (ms)(milliseconds to wait=u32 1500 ("대기 시간 (ms)")) -> ()  [unwired: 1 out]
            n452 = property on="Station_현황_GPS" class="MCListbox (엄격한)"() -> ("ItemNames"=w1728:string[][])  [unwired: 2 in, 2 out]
            n453 = call "Graph_Water_Velocity(Subvi).vi"("GPS_ItemNames"=w1728, "Velocity_ItemNames"=w1727) -> ("1_2_Water_Velocity"=w1720:dbl, "1_2_Averange_SoundSpeed"=w1662:dbl, "1_3_Water_Velocity"=w1717:dbl, "1_3Averange_SoundSpeed"=w1661:dbl, "1_4_Water_Velocity"=w1713:dbl, "1_4_Averange_SoundSpeed"=w1660:dbl, "1_5_Water_Velocity"=w1709:dbl, "1_5_Averange_SoundSpeed"=w1659:dbl, "2_3_Water_Velocity"=w1705:dbl, "2_3_Averange_SoundSpeed"=w1658:dbl, "2_4_Water_Velocity"=w1701:dbl, "2_4_Averange_SoundSpeed"=w1657:dbl, "2_5_Water_Velocity"=w1697:dbl, "3_4_Water_Velocity"=w1692:dbl, "3_5_Water_Velocity"=w1689:dbl, "4_5_Water_Velocity"=w1684:dbl, "4_5_Averange_SoundSpeed"=w1653:dbl, "3_5_Averange_SoundSpeed"=w1654:dbl, "3_4_Averange_SoundSpeed"=w1655:dbl, "2_5_Averange_SoundSpeed"=w1656:dbl)  [unwired: 6 in]
            n454 = Build Array(w1662) -> (w1665:dbl[])
            n455 = Get Date/Time In Seconds() -> (seconds since 1Jan1904=w1664:timestamp)
            n456 = Build Array(w1661) -> (w1666:dbl[])
            n457 = Get Date/Time In Seconds() -> (seconds since 1Jan1904=w1667:timestamp)
            n458 = Build Array(w1660) -> (w1669:dbl[])
            n459 = Get Date/Time In Seconds() -> (seconds since 1Jan1904=w1668:timestamp)
            n460 = Build Array(w1659) -> (w1670:dbl[])
            n461 = Get Date/Time In Seconds() -> (seconds since 1Jan1904=w1671:timestamp)
            n462 = Build Array(w1658) -> (w1673:dbl[])
            n463 = Get Date/Time In Seconds() -> (seconds since 1Jan1904=w1672:timestamp)
            n464 = Build Array(w1657) -> (w1674:dbl[])
            n465 = Get Date/Time In Seconds() -> (seconds since 1Jan1904=w1675:timestamp)
            n466 = Build Array(w1656) -> (w1677:dbl[])
            n467 = Get Date/Time In Seconds() -> (seconds since 1Jan1904=w1676:timestamp)
            n468 = Build Array(w1655) -> (w1679:dbl[])
            n469 = Get Date/Time In Seconds() -> (seconds since 1Jan1904=w1678:timestamp)
            n470 = Build Array(w1654) -> (w1680:dbl[])
            n471 = Get Date/Time In Seconds() -> (seconds since 1Jan1904=w1681:timestamp)
            n472 = Build Array(w1653) -> (w1683:dbl[])
            n473 = Get Date/Time In Seconds() -> (seconds since 1Jan1904=w1682:timestamp)
            n474 = Bundle By Name("Y"=w1665, "t0"=w1664) -> (→"Averange_Soundspeed_1_2":waveform(dbl))  [unwired: 1 in]
            n475 = Bundle By Name("Y"=w1666, "t0"=w1667) -> (→"Averange_Soundspeed_1_3":waveform(dbl))  [unwired: 1 in]
            n476 = Bundle By Name("Y"=w1669, "t0"=w1668) -> (→"Averange_Soundspeed_1_4":waveform(dbl))  [unwired: 1 in]
            n477 = Bundle By Name("Y"=w1670, "t0"=w1671) -> (→"Averange_Soundspeed_1_5":waveform(dbl))  [unwired: 1 in]
            n478 = Bundle By Name("Y"=w1673, "t0"=w1672) -> (→"Averange_Soundspeed_2_3":waveform(dbl))  [unwired: 1 in]
            n479 = Bundle By Name("Y"=w1674, "t0"=w1675) -> (→"Averange_Soundspeed_2_4":waveform(dbl))  [unwired: 1 in]
            n480 = Bundle By Name("Y"=w1677, "t0"=w1676) -> (→"Averange_Soundspeed_2_5":waveform(dbl))  [unwired: 1 in]
            n481 = Bundle By Name("Y"=w1679, "t0"=w1678) -> (→"Averange_Soundspeed_3_4":waveform(dbl))  [unwired: 1 in]
            n482 = Bundle By Name("Y"=w1680, "t0"=w1681) -> (→"Averange_Soundspeed_3_5":waveform(dbl))  [unwired: 1 in]
            n483 = Bundle By Name("Y"=w1683, "t0"=w1682) -> (→"Averange_Soundspeed_4_5":waveform(dbl))  [unwired: 1 in]
            n484 = Build Array(w1720) -> (w1721:dbl[])
            n485 = Get Date/Time In Seconds() -> (seconds since 1Jan1904=w1723:timestamp)
            n486 = Build Array(w1717) -> (w1719:dbl[])
            n487 = Get Date/Time In Seconds() -> (seconds since 1Jan1904=w1718:timestamp)
            n488 = Build Array(w1713) -> (w1715:dbl[])
            n489 = Get Date/Time In Seconds() -> (seconds since 1Jan1904=w1716:timestamp)
            n490 = Build Array(w1709) -> (w1712:dbl[])
            n491 = Get Date/Time In Seconds() -> (seconds since 1Jan1904=w1711:timestamp)
            n492 = Build Array(w1705) -> (w1707:dbl[])
            n493 = Get Date/Time In Seconds() -> (seconds since 1Jan1904=w1708:timestamp)
            n494 = Build Array(w1701) -> (w1704:dbl[])
            n495 = Get Date/Time In Seconds() -> (seconds since 1Jan1904=w1703:timestamp)
            n496 = Build Array(w1697) -> (w1698:dbl[])
            n497 = Get Date/Time In Seconds() -> (seconds since 1Jan1904=w1699:timestamp)
            n498 = Build Array(w1692) -> (w1694:dbl[])
            n499 = Get Date/Time In Seconds() -> (seconds since 1Jan1904=w1696:timestamp)
            n500 = Build Array(w1689) -> (w1691:dbl[])
            n501 = Get Date/Time In Seconds() -> (seconds since 1Jan1904=w1690:timestamp)
            n502 = Build Array(w1684) -> (w1687:dbl[])
            n503 = Get Date/Time In Seconds() -> (seconds since 1Jan1904=w1688:timestamp)
            n504 = Bundle By Name("Y"=w1721, "t0"=w1723) -> (→"Water_Velocity_1_2":waveform(dbl))  [unwired: 1 in]
            n505 = Bundle By Name("Y"=w1719, "t0"=w1718) -> (→"Water_Velocity_1_3":waveform(dbl))  [unwired: 1 in]
            n506 = Bundle By Name("Y"=w1715, "t0"=w1716) -> (→"Water_Velocity_1_4":waveform(dbl))  [unwired: 1 in]
            n507 = Bundle By Name("Y"=w1712, "t0"=w1711) -> (→"Water_Velocity_1_5":waveform(dbl))  [unwired: 1 in]
            n508 = Bundle By Name("Y"=w1707, "t0"=w1708) -> (→"Water_Velocity_2_3":waveform(dbl))  [unwired: 1 in]
            n509 = Bundle By Name("Y"=w1704, "t0"=w1703) -> (→"Water_Velocity_2_4":waveform(dbl))  [unwired: 1 in]
            n510 = Bundle By Name("Y"=w1698, "t0"=w1699) -> (→"Water_Velocity_2_5":waveform(dbl))  [unwired: 1 in]
            n511 = Bundle By Name("Y"=w1694, "t0"=w1696) -> (→"Water_Velocity_3_4":waveform(dbl))  [unwired: 1 in]
            n512 = Bundle By Name("Y"=w1691, "t0"=w1690) -> (→"Water_Velocity_3_5":waveform(dbl))  [unwired: 1 in]
            n513 = Bundle By Name("Y"=w1687, "t0"=w1688) -> (→"Water_Velocity_4_5":waveform(dbl))  [unwired: 1 in]
            n514 = Bundle By Name(cluster=w1725, "Water_Velocity_1_3"=w1717, "Water_Velocity_1_2"=w1720, "Water_Velocity_1_4"=w1713, "Water_Velocity_1_5"=w1709, "Water_Velocity_2_3"=w1705, "Water_Velocity_2_4"=w1701, "Water_Velocity_2_5"=w1697, "Water_Velocity_3_4"=w1692, "Water_Velocity_3_5"=w1689, "Water_Velocity_4_5"=w1684, "Averange_Soundspeed_1_2"=w1662, "Averange_Soundspeed_1_3"=w1661, "Averange_Soundspeed_1_4"=w1660, "Averange_Soundspeed_1_5"=w1659, "Averange_Soundspeed_2_3"=w1658, "Averange_Soundspeed_2_4"=w1657, "Averange_Soundspeed_2_5"=w1656, "Averange_Soundspeed_3_4"=w1655, "Averange_Soundspeed_3_5"=w1654, "Averange_Soundspeed_4_5"=w1653) -> (w1724:T5)
          }
        }
      }
      frame 36 {
        n515 = case shown="3" w1731 {
          tunnel: w1730 -> [w1732 w1814]
          tunnel: [w1732 w1813] -> w1729
          frame 0, Default {
          }
          frame 3 {
            n516 = property on="유속 데이터 흐름표_30분" class="MCListbox (엄격한)"() -> ("ItemNames"=w1816:string[][])  [unwired: 2 in, 2 out]
            n517 = Wait (ms)(milliseconds to wait=u32 1500 ("대기 시간 (ms)")) -> ()  [unwired: 1 out]
            n518 = property on="Station_현황_GPS" class="MCListbox (엄격한)"() -> ("ItemNames"=w1817:string[][])  [unwired: 2 in, 2 out]
            n519 = call "Graph_Water_Velocity(Subvi).vi"("GPS_ItemNames"=w1817, "Velocity_ItemNames"=w1816) -> ("1_2_Water_Velocity"=w1772:dbl, "1_2_Averange_SoundSpeed"=w1742:dbl, "1_3_Water_Velocity"=w1771:dbl, "1_3Averange_SoundSpeed"=w1741:dbl, "1_4_Water_Velocity"=w1770:dbl, "1_4_Averange_SoundSpeed"=w1740:dbl, "1_5_Water_Velocity"=w1769:dbl, "1_5_Averange_SoundSpeed"=w1739:dbl, "2_3_Water_Velocity"=w1768:dbl, "2_3_Averange_SoundSpeed"=w1738:dbl, "2_4_Water_Velocity"=w1767:dbl, "2_4_Averange_SoundSpeed"=w1737:dbl, "2_5_Water_Velocity"=w1766:dbl, "3_4_Water_Velocity"=w1765:dbl, "3_5_Water_Velocity"=w1764:dbl, "4_5_Water_Velocity"=w1763:dbl, "4_5_Averange_SoundSpeed"=w1733:dbl, "3_5_Averange_SoundSpeed"=w1734:dbl, "3_4_Averange_SoundSpeed"=w1735:dbl, "2_5_Averange_SoundSpeed"=w1736:dbl)  [unwired: 6 in]
            n520 = Build Array(w1742) -> (w1774:dbl[])
            n521 = Get Date/Time In Seconds() -> (seconds since 1Jan1904=w1773:timestamp)
            n522 = Build Array(w1741) -> (w1775:dbl[])
            n523 = Get Date/Time In Seconds() -> (seconds since 1Jan1904=w1776:timestamp)
            n524 = Build Array(w1740) -> (w1778:dbl[])
            n525 = Get Date/Time In Seconds() -> (seconds since 1Jan1904=w1777:timestamp)
            n526 = Build Array(w1739) -> (w1779:dbl[])
            n527 = Get Date/Time In Seconds() -> (seconds since 1Jan1904=w1780:timestamp)
            n528 = Build Array(w1738) -> (w1782:dbl[])
            n529 = Get Date/Time In Seconds() -> (seconds since 1Jan1904=w1781:timestamp)
            n530 = Build Array(w1737) -> (w1783:dbl[])
            n531 = Get Date/Time In Seconds() -> (seconds since 1Jan1904=w1784:timestamp)
            n532 = Build Array(w1736) -> (w1786:dbl[])
            n533 = Get Date/Time In Seconds() -> (seconds since 1Jan1904=w1785:timestamp)
            n534 = Build Array(w1735) -> (w1788:dbl[])
            n535 = Get Date/Time In Seconds() -> (seconds since 1Jan1904=w1787:timestamp)
            n536 = Build Array(w1734) -> (w1789:dbl[])
            n537 = Get Date/Time In Seconds() -> (seconds since 1Jan1904=w1790:timestamp)
            n538 = Build Array(w1733) -> (w1792:dbl[])
            n539 = Get Date/Time In Seconds() -> (seconds since 1Jan1904=w1791:timestamp)
            n540 = Bundle By Name("Y"=w1774, "t0"=w1773) -> (w1752:waveform(dbl))  [unwired: 1 in]
            n541 = Bundle By Name("Y"=w1775, "t0"=w1776) -> (w1751:waveform(dbl))  [unwired: 1 in]
            n542 = Bundle By Name("Y"=w1778, "t0"=w1777) -> (w1750:waveform(dbl))  [unwired: 1 in]
            n543 = Bundle By Name("Y"=w1779, "t0"=w1780) -> (w1749:waveform(dbl))  [unwired: 1 in]
            n544 = Bundle By Name("Y"=w1782, "t0"=w1781) -> (w1748:waveform(dbl))  [unwired: 1 in]
            n545 = Bundle By Name("Y"=w1783, "t0"=w1784) -> (w1747:waveform(dbl))  [unwired: 1 in]
            n546 = Bundle By Name("Y"=w1786, "t0"=w1785) -> (w1746:waveform(dbl))  [unwired: 1 in]
            n547 = Bundle By Name("Y"=w1788, "t0"=w1787) -> (w1745:waveform(dbl))  [unwired: 1 in]
            n548 = Bundle By Name("Y"=w1789, "t0"=w1790) -> (w1744:waveform(dbl))  [unwired: 1 in]
            n549 = Bundle By Name("Y"=w1792, "t0"=w1791) -> (w1743:waveform(dbl))  [unwired: 1 in]
            n550 = local write "Averange_Soundspeed_1_2"(w1752) -> ()
            n551 = local write "Averange_Soundspeed_1_3"(w1751) -> ()
            n552 = local write "Averange_Soundspeed_1_4"(w1750) -> ()
            n553 = local write "Averange_Soundspeed_1_5"(w1749) -> ()
            n554 = local write "Averange_Soundspeed_2_3"(w1748) -> ()
            n555 = local write "Averange_Soundspeed_2_5"(w1746) -> ()
            n556 = local write "Averange_Soundspeed_2_4"(w1747) -> ()
            n557 = local write "Averange_Soundspeed_3_4"(w1745) -> ()
            n558 = local write "Averange_Soundspeed_3_5"(w1744) -> ()
            n559 = local write "Averange_Soundspeed_4_5"(w1743) -> ()
            n560 = Build Array(w1772) -> (w1794:dbl[])
            n561 = Get Date/Time In Seconds() -> (seconds since 1Jan1904=w1793:timestamp)
            n562 = Build Array(w1771) -> (w1795:dbl[])
            n563 = Get Date/Time In Seconds() -> (seconds since 1Jan1904=w1796:timestamp)
            n564 = Build Array(w1770) -> (w1798:dbl[])
            n565 = Get Date/Time In Seconds() -> (seconds since 1Jan1904=w1797:timestamp)
            n566 = Build Array(w1769) -> (w1799:dbl[])
            n567 = Get Date/Time In Seconds() -> (seconds since 1Jan1904=w1800:timestamp)
            n568 = Build Array(w1768) -> (w1802:dbl[])
            n569 = Get Date/Time In Seconds() -> (seconds since 1Jan1904=w1801:timestamp)
            n570 = Build Array(w1767) -> (w1803:dbl[])
            n571 = Get Date/Time In Seconds() -> (seconds since 1Jan1904=w1804:timestamp)
            n572 = Build Array(w1766) -> (w1806:dbl[])
            n573 = Get Date/Time In Seconds() -> (seconds since 1Jan1904=w1805:timestamp)
            n574 = Build Array(w1765) -> (w1808:dbl[])
            n575 = Get Date/Time In Seconds() -> (seconds since 1Jan1904=w1807:timestamp)
            n576 = Build Array(w1764) -> (w1809:dbl[])
            n577 = Get Date/Time In Seconds() -> (seconds since 1Jan1904=w1810:timestamp)
            n578 = Build Array(w1763) -> (w1812:dbl[])
            n579 = Get Date/Time In Seconds() -> (seconds since 1Jan1904=w1811:timestamp)
            n580 = Bundle By Name("Y"=w1794, "t0"=w1793) -> (w1762:waveform(dbl))  [unwired: 1 in]
            n581 = Bundle By Name("Y"=w1795, "t0"=w1796) -> (w1761:waveform(dbl))  [unwired: 1 in]
            n582 = Bundle By Name("Y"=w1798, "t0"=w1797) -> (w1760:waveform(dbl))  [unwired: 1 in]
            n583 = Bundle By Name("Y"=w1799, "t0"=w1800) -> (w1759:waveform(dbl))  [unwired: 1 in]
            n584 = Bundle By Name("Y"=w1802, "t0"=w1801) -> (w1758:waveform(dbl))  [unwired: 1 in]
            n585 = Bundle By Name("Y"=w1803, "t0"=w1804) -> (w1757:waveform(dbl))  [unwired: 1 in]
            n586 = Bundle By Name("Y"=w1806, "t0"=w1805) -> (w1756:waveform(dbl))  [unwired: 1 in]
            n587 = Bundle By Name("Y"=w1808, "t0"=w1807) -> (w1755:waveform(dbl))  [unwired: 1 in]
            n588 = Bundle By Name("Y"=w1809, "t0"=w1810) -> (w1754:waveform(dbl))  [unwired: 1 in]
            n589 = Bundle By Name("Y"=w1812, "t0"=w1811) -> (w1753:waveform(dbl))  [unwired: 1 in]
            n590 = local write "Water_Velocity_1_2"(w1762) -> ()
            n591 = local write "Water_Velocity_1_3"(w1761) -> ()
            n592 = local write "Water_Velocity_1_4"(w1760) -> ()
            n593 = local write "Water_Velocity_1_5"(w1759) -> ()
            n594 = local write "Water_Velocity_2_3"(w1758) -> ()
            n595 = local write "Water_Velocity_2_4"(w1757) -> ()
            n596 = local write "Water_Velocity_2_5"(w1756) -> ()
            n597 = local write "Water_Velocity_3_4"(w1755) -> ()
            n598 = local write "Water_Velocity_3_5"(w1754) -> ()
            n599 = local write "Water_Velocity_4_5"(w1753) -> ()
            n600 = Bundle By Name(cluster=w1814, "Water_Velocity_1_3"=w1771, "Water_Velocity_1_2"=w1772, "Water_Velocity_1_4"=w1770, "Water_Velocity_1_5"=w1769, "Water_Velocity_2_3"=w1768, "Water_Velocity_2_4"=w1767, "Water_Velocity_2_5"=w1766, "Water_Velocity_3_4"=w1765, "Water_Velocity_3_5"=w1764, "Water_Velocity_4_5"=w1763, "Averange_Soundspeed_1_2"=w1742, "Averange_Soundspeed_1_3"=w1741, "Averange_Soundspeed_1_4"=w1740, "Averange_Soundspeed_1_5"=w1739, "Averange_Soundspeed_2_3"=w1738, "Averange_Soundspeed_2_4"=w1737, "Averange_Soundspeed_2_5"=w1736, "Averange_Soundspeed_3_4"=w1735, "Averange_Soundspeed_3_5"=w1734, "Averange_Soundspeed_4_5"=w1733) -> (w1813:T5)
          }
        }
      }
      frame 56 {
        n601 = case shown="3" w1820 {
          tunnel: w1819 -> [w1821 w1903]
          tunnel: [w1821 w1902] -> w1818
          frame 0, Default {
          }
          frame 3 {
            n602 = property on="유속 데이터 흐름표_50분" class="MCListbox (엄격한)"() -> ("ItemNames"=w1905:string[][])  [unwired: 2 in, 2 out]
            n603 = Wait (ms)(milliseconds to wait=u32 1500 ("대기 시간 (ms)")) -> ()  [unwired: 1 out]
            n604 = property on="Station_현황_GPS" class="MCListbox (엄격한)"() -> ("ItemNames"=w1906:string[][])  [unwired: 2 in, 2 out]
            n605 = call "Graph_Water_Velocity(Subvi).vi"("GPS_ItemNames"=w1906, "Velocity_ItemNames"=w1905) -> ("1_2_Water_Velocity"=w1841:dbl, "1_2_Averange_SoundSpeed"=w1831:dbl, "1_3_Water_Velocity"=w1840:dbl, "1_3Averange_SoundSpeed"=w1830:dbl, "1_4_Water_Velocity"=w1839:dbl, "1_4_Averange_SoundSpeed"=w1829:dbl, "1_5_Water_Velocity"=w1838:dbl, "1_5_Averange_SoundSpeed"=w1828:dbl, "2_3_Water_Velocity"=w1837:dbl, "2_3_Averange_SoundSpeed"=w1827:dbl, "2_4_Water_Velocity"=w1836:dbl, "2_4_Averange_SoundSpeed"=w1826:dbl, "2_5_Water_Velocity"=w1835:dbl, "3_4_Water_Velocity"=w1834:dbl, "3_5_Water_Velocity"=w1833:dbl, "4_5_Water_Velocity"=w1832:dbl, "4_5_Averange_SoundSpeed"=w1822:dbl, "3_5_Averange_SoundSpeed"=w1823:dbl, "3_4_Averange_SoundSpeed"=w1824:dbl, "2_5_Averange_SoundSpeed"=w1825:dbl)  [unwired: 6 in]
            n606 = Build Array(w1831) -> (w1853:dbl[])
            n607 = Get Date/Time In Seconds() -> (seconds since 1Jan1904=w1852:timestamp)
            n608 = Build Array(w1830) -> (w1854:dbl[])
            n609 = Get Date/Time In Seconds() -> (seconds since 1Jan1904=w1855:timestamp)
            n610 = Build Array(w1829) -> (w1857:dbl[])
            n611 = Get Date/Time In Seconds() -> (seconds since 1Jan1904=w1856:timestamp)
            n612 = Build Array(w1828) -> (w1858:dbl[])
            n613 = Get Date/Time In Seconds() -> (seconds since 1Jan1904=w1859:timestamp)
            n614 = Build Array(w1827) -> (w1861:dbl[])
            n615 = Get Date/Time In Seconds() -> (seconds since 1Jan1904=w1860:timestamp)
            n616 = Build Array(w1826) -> (w1862:dbl[])
            n617 = Get Date/Time In Seconds() -> (seconds since 1Jan1904=w1863:timestamp)
            n618 = Build Array(w1825) -> (w1865:dbl[])
            n619 = Get Date/Time In Seconds() -> (seconds since 1Jan1904=w1864:timestamp)
            n620 = Build Array(w1824) -> (w1867:dbl[])
            n621 = Get Date/Time In Seconds() -> (seconds since 1Jan1904=w1866:timestamp)
            n622 = Build Array(w1823) -> (w1868:dbl[])
            n623 = Get Date/Time In Seconds() -> (seconds since 1Jan1904=w1869:timestamp)
            n624 = Build Array(w1822) -> (w1871:dbl[])
            n625 = Get Date/Time In Seconds() -> (seconds since 1Jan1904=w1870:timestamp)
            n626 = Bundle By Name("Y"=w1853, "t0"=w1852) -> (w1851:waveform(dbl))  [unwired: 1 in]
            n627 = Bundle By Name("Y"=w1854, "t0"=w1855) -> (w1850:waveform(dbl))  [unwired: 1 in]
            n628 = Bundle By Name("Y"=w1857, "t0"=w1856) -> (w1849:waveform(dbl))  [unwired: 1 in]
            n629 = Bundle By Name("Y"=w1858, "t0"=w1859) -> (w1848:waveform(dbl))  [unwired: 1 in]
            n630 = Bundle By Name("Y"=w1861, "t0"=w1860) -> (w1847:waveform(dbl))  [unwired: 1 in]
            n631 = Bundle By Name("Y"=w1862, "t0"=w1863) -> (w1846:waveform(dbl))  [unwired: 1 in]
            n632 = Bundle By Name("Y"=w1865, "t0"=w1864) -> (w1845:waveform(dbl))  [unwired: 1 in]
            n633 = Bundle By Name("Y"=w1867, "t0"=w1866) -> (w1844:waveform(dbl))  [unwired: 1 in]
            n634 = Bundle By Name("Y"=w1868, "t0"=w1869) -> (w1843:waveform(dbl))  [unwired: 1 in]
            n635 = Bundle By Name("Y"=w1871, "t0"=w1870) -> (w1842:waveform(dbl))  [unwired: 1 in]
            n636 = local write "Averange_Soundspeed_1_2"(w1851) -> ()
            n637 = local write "Averange_Soundspeed_1_3"(w1850) -> ()
            n638 = local write "Averange_Soundspeed_1_4"(w1849) -> ()
            n639 = local write "Averange_Soundspeed_1_5"(w1848) -> ()
            n640 = local write "Averange_Soundspeed_2_3"(w1847) -> ()
            n641 = local write "Averange_Soundspeed_2_5"(w1845) -> ()
            n642 = local write "Averange_Soundspeed_2_4"(w1846) -> ()
            n643 = local write "Averange_Soundspeed_3_4"(w1844) -> ()
            n644 = local write "Averange_Soundspeed_3_5"(w1843) -> ()
            n645 = local write "Averange_Soundspeed_4_5"(w1842) -> ()
            n646 = Build Array(w1841) -> (w1883:dbl[])
            n647 = Get Date/Time In Seconds() -> (seconds since 1Jan1904=w1882:timestamp)
            n648 = Build Array(w1840) -> (w1884:dbl[])
            n649 = Get Date/Time In Seconds() -> (seconds since 1Jan1904=w1885:timestamp)
            n650 = Build Array(w1839) -> (w1887:dbl[])
            n651 = Get Date/Time In Seconds() -> (seconds since 1Jan1904=w1886:timestamp)
            n652 = Build Array(w1838) -> (w1888:dbl[])
            n653 = Get Date/Time In Seconds() -> (seconds since 1Jan1904=w1889:timestamp)
            n654 = Build Array(w1837) -> (w1891:dbl[])
            n655 = Get Date/Time In Seconds() -> (seconds since 1Jan1904=w1890:timestamp)
            n656 = Build Array(w1836) -> (w1892:dbl[])
            n657 = Get Date/Time In Seconds() -> (seconds since 1Jan1904=w1893:timestamp)
            n658 = Build Array(w1835) -> (w1895:dbl[])
            n659 = Get Date/Time In Seconds() -> (seconds since 1Jan1904=w1894:timestamp)
            n660 = Build Array(w1834) -> (w1897:dbl[])
            n661 = Get Date/Time In Seconds() -> (seconds since 1Jan1904=w1896:timestamp)
            n662 = Build Array(w1833) -> (w1898:dbl[])
            n663 = Get Date/Time In Seconds() -> (seconds since 1Jan1904=w1899:timestamp)
            n664 = Build Array(w1832) -> (w1901:dbl[])
            n665 = Get Date/Time In Seconds() -> (seconds since 1Jan1904=w1900:timestamp)
            n666 = Bundle By Name("Y"=w1883, "t0"=w1882) -> (w1881:waveform(dbl))  [unwired: 1 in]
            n667 = Bundle By Name("Y"=w1884, "t0"=w1885) -> (w1880:waveform(dbl))  [unwired: 1 in]
            n668 = Bundle By Name("Y"=w1887, "t0"=w1886) -> (w1879:waveform(dbl))  [unwired: 1 in]
            n669 = Bundle By Name("Y"=w1888, "t0"=w1889) -> (w1878:waveform(dbl))  [unwired: 1 in]
            n670 = Bundle By Name("Y"=w1891, "t0"=w1890) -> (w1877:waveform(dbl))  [unwired: 1 in]
            n671 = Bundle By Name("Y"=w1892, "t0"=w1893) -> (w1876:waveform(dbl))  [unwired: 1 in]
            n672 = Bundle By Name("Y"=w1895, "t0"=w1894) -> (w1875:waveform(dbl))  [unwired: 1 in]
            n673 = Bundle By Name("Y"=w1897, "t0"=w1896) -> (w1874:waveform(dbl))  [unwired: 1 in]
            n674 = Bundle By Name("Y"=w1898, "t0"=w1899) -> (w1873:waveform(dbl))  [unwired: 1 in]
            n675 = Bundle By Name("Y"=w1901, "t0"=w1900) -> (w1872:waveform(dbl))  [unwired: 1 in]
            n676 = local write "Water_Velocity_1_2"(w1881) -> ()
            n677 = local write "Water_Velocity_1_3"(w1880) -> ()
            n678 = local write "Water_Velocity_1_4"(w1879) -> ()
            n679 = local write "Water_Velocity_1_5"(w1878) -> ()
            n680 = local write "Water_Velocity_2_3"(w1877) -> ()
            n681 = local write "Water_Velocity_2_4"(w1876) -> ()
            n682 = local write "Water_Velocity_2_5"(w1875) -> ()
            n683 = local write "Water_Velocity_3_4"(w1874) -> ()
            n684 = local write "Water_Velocity_3_5"(w1873) -> ()
            n685 = local write "Water_Velocity_4_5"(w1872) -> ()
            n686 = Bundle By Name(cluster=w1903, "Water_Velocity_1_3"=w1840, "Water_Velocity_1_2"=w1841, "Water_Velocity_1_4"=w1839, "Water_Velocity_1_5"=w1838, "Water_Velocity_2_3"=w1837, "Water_Velocity_2_4"=w1836, "Water_Velocity_2_5"=w1835, "Water_Velocity_3_4"=w1834, "Water_Velocity_3_5"=w1833, "Water_Velocity_4_5"=w1832, "Averange_Soundspeed_1_2"=w1831, "Averange_Soundspeed_1_3"=w1830, "Averange_Soundspeed_1_4"=w1829, "Averange_Soundspeed_1_5"=w1828, "Averange_Soundspeed_2_3"=w1827, "Averange_Soundspeed_2_4"=w1826, "Averange_Soundspeed_2_5"=w1825, "Averange_Soundspeed_3_4"=w1824, "Averange_Soundspeed_3_5"=w1823, "Averange_Soundspeed_4_5"=w1822) -> (w1902:T5)
          }
        }
      }
    }
    n687 = case shown="거짓" w1405 {
      frame False {
        n688 = flat-sequence {
          frame #0 {
            n689 = Format Date/Time String(time format string (%c)="%d" ("시간 포맷 문자열 (%c)")) -> (date/time string=w1445:string)  [unwired: 2 in]
            n690 = local write "현재 날짜"(w1445) -> ()
          }
          frame #1 {
            w1632 = T10 1 items=["사용자 홈"=0, "사용자 데스크탑"=1, "사용자 문서"=2, "사용자 어플리케이션 데이터"=3, "사용자 환경"=4, "사용자 임시"=5, "퍼블릭 문서"=6, "퍼블릭 어플리케이션 데이터"=7, "퍼블릭 환경"=8, "퍼블릭 캐시"=13, "시스템 코어 라이브러리"=9, "시스템 설치된 라이브러리"=10, "어플리케이션 파일"=11, "부팅 볼륨 루트"=12] ("system directory type")
            n691 = call <vilib>:"Get System Directory.vi"("system directory type"=w1632) -> ("system directory"=w1631:path)  [unwired: 10 in]
            n692 = Build Path(base path=w1631, name or relative path=path "CSV_DATA" ("이름 또는 상대 경로")) -> (appended path=w1629:path)
            n693 = call <vilib>:"Check if File or Folder Exists.vi"("path"=w1629) -> ("file or folder exists?"=w1628:bool, "dup path"=w1627:path)  [unwired: 8 in, 1 out]
            n694 = case shown="참" w1628 {
              tunnel: [w1633 w1635] -> w1451
              tunnel: w1627 -> [w1634 w1635]
              frame False {
                n695 = Create Folder(path (use dialog)=w1634) -> (created path=w1633:path)  [unwired: 2 in, 2 out]
              }
              frame True {
              }
            }
            n696 = Concatenate Strings("Averange_Soundspeed_1_5_%Y_%m_%d" ("시간 포맷 문자열 (%c)"), ".png" ("시간 포맷 문자열 (%c)")) -> (w1508:string)
            n697 = Concatenate Strings("Water_Velocity_1_2_%Y_%m_%d" ("시간 포맷 문자열 (%c)"), ".png" ("시간 포맷 문자열 (%c)")) -> (w1624:string)
            n698 = Concatenate Strings("Water_Velocity_1_3_%Y_%m_%d" ("시간 포맷 문자열 (%c)"), ".png" ("시간 포맷 문자열 (%c)")) -> (w1616:string)
            n699 = Concatenate Strings("Water_Velocity_1_4_%Y_%m_%d" ("시간 포맷 문자열 (%c)"), ".png" ("시간 포맷 문자열 (%c)")) -> (w1606:string)
            n700 = Concatenate Strings("Water_Velocity_2_3_%Y_%m_%d" ("시간 포맷 문자열 (%c)"), ".png" ("시간 포맷 문자열 (%c)")) -> (w1588:string)
            n701 = Concatenate Strings("Water_Velocity_1_5_%Y_%m_%d" ("시간 포맷 문자열 (%c)"), ".png" ("시간 포맷 문자열 (%c)")) -> (w1598:string)
            n702 = Concatenate Strings("Averange_Soundspeed_2_5_%Y_%m_%d" ("시간 포맷 문자열 (%c)"), ".png" ("시간 포맷 문자열 (%c)")) -> (w1481:string)
            n703 = Concatenate Strings("Averange_Soundspeed_4_5_%Y_%m_%d" ("시간 포맷 문자열 (%c)"), ".png" ("시간 포맷 문자열 (%c)")) -> (w1455:string)
            n704 = Format Date/Time String(time format string (%c)=w1508) -> (date/time string=w1509:string)  [unwired: 2 in]
            n705 = Format Date/Time String(time format string (%c)=w1624) -> (date/time string=w1623:string)  [unwired: 2 in]
            n706 = Format Date/Time String(time format string (%c)=w1616) -> (date/time string=w1617:string)  [unwired: 2 in]
            n707 = Format Date/Time String(time format string (%c)=w1606) -> (date/time string=w1605:string)  [unwired: 2 in]
            n708 = Format Date/Time String(time format string (%c)=w1588) -> (date/time string=w1587:string)  [unwired: 2 in]
            n709 = Format Date/Time String(time format string (%c)=w1598) -> (date/time string=w1599:string)  [unwired: 2 in]
            n710 = Format Date/Time String(time format string (%c)=w1481) -> (date/time string=w1480:string)  [unwired: 2 in]
            n711 = Format Date/Time String(time format string (%c)=w1455) -> (date/time string=w1456:string)  [unwired: 2 in]
            n712 = Build Path(base path=w1451, name or relative path=w1509) -> (appended path=w1505:path)
            n713 = Build Path(base path=w1451, name or relative path=w1623) -> (appended path=w1622:path)
            n714 = Build Path(base path=w1451, name or relative path=w1617) -> (appended path=w1613:path)
            n715 = Build Path(base path=w1451, name or relative path=w1605) -> (appended path=w1604:path)
            n716 = Build Path(base path=w1451, name or relative path=w1587) -> (appended path=w1586:path)
            n717 = Build Path(base path=w1451, name or relative path=w1599) -> (appended path=w1595:path)
            n718 = Build Path(base path=w1451, name or relative path=w1480) -> (appended path=w1479:path)
            n719 = Build Path(base path=w1451, name or relative path=w1456) -> (appended path=w1452:path)
            n720 = invoke on="Water_Velocity_1_2" class="WFChart (엄격한)" method="Export Image"("FileType"=enum32{"BMP", "EPS", "EMF", "PICT"}."BMP" ("파일 타입"), "Target"=enum32{"File", "Clipboard"}."File" ("타겟"), "Path"=w1622, "HideGrid"=FALSE ("눈금 숨기기"), "Overwrite"=TRUE ("항상 덮어쓰기")) -> ()  [unwired: 3 in, 8 out]
            n721 = invoke on="Water_Velocity_1_3" class="WFChart (엄격한)" method="Export Image"("FileType"=enum32{"BMP", "EPS", "EMF", "PICT"}."BMP" ("파일 타입"), "Target"=enum32{"File", "Clipboard"}."File" ("타겟"), "Path"=w1613, "HideGrid"=FALSE ("눈금 숨기기"), "Overwrite"=TRUE ("항상 덮어쓰기")) -> ()  [unwired: 3 in, 8 out]
            n722 = invoke on="Water_Velocity_1_4" class="WFChart (엄격한)" method="Export Image"("FileType"=enum32{"BMP", "EPS", "EMF", "PICT"}."BMP" ("파일 타입"), "Target"=enum32{"File", "Clipboard"}."File" ("타겟"), "Path"=w1604, "HideGrid"=FALSE ("눈금 숨기기"), "Overwrite"=TRUE ("항상 덮어쓰기")) -> ()  [unwired: 3 in, 8 out]
            n723 = invoke on="Averange_Soundspeed_4_5" class="WFChart (엄격한)" method="Export Image"("FileType"=enum32{"BMP", "EPS", "EMF", "PICT"}."BMP" ("파일 타입"), "Target"=enum32{"File", "Clipboard"}."File" ("타겟"), "Path"=w1452, "HideGrid"=FALSE ("눈금 숨기기"), "Overwrite"=TRUE ("항상 덮어쓰기")) -> ()  [unwired: 3 in, 8 out]
            n724 = invoke on="Water_Velocity_1_5" class="WFChart (엄격한)" method="Export Image"("FileType"=enum32{"BMP", "EPS", "EMF", "PICT"}."BMP" ("파일 타입"), "Target"=enum32{"File", "Clipboard"}."File" ("타겟"), "Path"=w1595, "HideGrid"=FALSE ("눈금 숨기기"), "Overwrite"=TRUE ("항상 덮어쓰기")) -> ()  [unwired: 3 in, 8 out]
            n725 = invoke on="Averange_Soundspeed_1_5" class="WFChart (엄격한)" method="Export Image"("FileType"=enum32{"BMP", "EPS", "EMF", "PICT"}."BMP" ("파일 타입"), "Target"=enum32{"File", "Clipboard"}."File" ("타겟"), "Path"=w1505, "HideGrid"=FALSE ("눈금 숨기기"), "Overwrite"=TRUE ("항상 덮어쓰기")) -> ()  [unwired: 3 in, 8 out]
            n726 = invoke on="Averange_Soundspeed_2_5" class="WFChart (엄격한)" method="Export Image"("FileType"=enum32{"BMP", "EPS", "EMF", "PICT"}."BMP" ("파일 타입"), "Target"=enum32{"File", "Clipboard"}."File" ("타겟"), "Path"=w1479, "HideGrid"=FALSE ("눈금 숨기기"), "Overwrite"=TRUE ("항상 덮어쓰기")) -> ()  [unwired: 3 in, 8 out]
            n727 = invoke on="Water_Velocity_2_3" class="WFChart (엄격한)" method="Export Image"("FileType"=enum32{"BMP", "EPS", "EMF", "PICT"}."BMP" ("파일 타입"), "Target"=enum32{"File", "Clipboard"}."File" ("타겟"), "Path"=w1586, "HideGrid"=FALSE ("눈금 숨기기"), "Overwrite"=TRUE ("항상 덮어쓰기")) -> ()  [unwired: 3 in, 8 out]
            n728 = Concatenate Strings("Water_Velocity_2_4_%Y_%m_%d" ("시간 포맷 문자열 (%c)"), ".png" ("시간 포맷 문자열 (%c)")) -> (w1580:string)
            n729 = Concatenate Strings("Water_Velocity_2_5_%Y_%m_%d" ("시간 포맷 문자열 (%c)"), ".png" ("시간 포맷 문자열 (%c)")) -> (w1570:string)
            n730 = Concatenate Strings("Water_Velocity_3_4_%Y_%m_%d" ("시간 포맷 문자열 (%c)"), ".png" ("시간 포맷 문자열 (%c)")) -> (w1562:string)
            n731 = Concatenate Strings("Water_Velocity_3_5_%Y_%m_%d" ("시간 포맷 문자열 (%c)"), ".png" ("시간 포맷 문자열 (%c)")) -> (w1552:string)
            n732 = Concatenate Strings("Averange_Soundspeed_2_3_%Y_%m_%d" ("시간 포맷 문자열 (%c)"), ".png" ("시간 포맷 문자열 (%c)")) -> (w1499:string)
            n733 = Concatenate Strings("Averange_Soundspeed_3_4_%Y_%m_%d" ("시간 포맷 문자열 (%c)"), ".png" ("시간 포맷 문자열 (%c)")) -> (w1472:string)
            n734 = Format Date/Time String(time format string (%c)=w1580) -> (date/time string=w1581:string)  [unwired: 2 in]
            n735 = Format Date/Time String(time format string (%c)=w1570) -> (date/time string=w1569:string)  [unwired: 2 in]
            n736 = Format Date/Time String(time format string (%c)=w1562) -> (date/time string=w1563:string)  [unwired: 2 in]
            n737 = Format Date/Time String(time format string (%c)=w1552) -> (date/time string=w1551:string)  [unwired: 2 in]
            n738 = Format Date/Time String(time format string (%c)=w1499) -> (date/time string=w1500:string)  [unwired: 2 in]
            n739 = Format Date/Time String(time format string (%c)=w1472) -> (date/time string=w1471:string)  [unwired: 2 in]
            n740 = Build Path(base path=w1451, name or relative path=w1581) -> (appended path=w1577:path)
            n741 = Build Path(base path=w1451, name or relative path=w1569) -> (appended path=w1568:path)
            n742 = Build Path(base path=w1451, name or relative path=w1563) -> (appended path=w1559:path)
            n743 = Build Path(base path=w1451, name or relative path=w1551) -> (appended path=w1550:path)
            n744 = Build Path(base path=w1451, name or relative path=w1500) -> (appended path=w1496:path)
            n745 = Build Path(base path=w1451, name or relative path=w1471) -> (appended path=w1470:path)
            n746 = invoke on="Water_Velocity_2_4" class="WFChart (엄격한)" method="Export Image"("FileType"=enum32{"BMP", "EPS", "EMF", "PICT"}."BMP" ("파일 타입"), "Target"=enum32{"File", "Clipboard"}."File" ("타겟"), "Path"=w1577, "HideGrid"=FALSE ("눈금 숨기기"), "Overwrite"=TRUE ("항상 덮어쓰기")) -> ()  [unwired: 3 in, 8 out]
            n747 = invoke on="Water_Velocity_2_5" class="WFChart (엄격한)" method="Export Image"("FileType"=enum32{"BMP", "EPS", "EMF", "PICT"}."BMP" ("파일 타입"), "Target"=enum32{"File", "Clipboard"}."File" ("타겟"), "Path"=w1568, "HideGrid"=FALSE ("눈금 숨기기"), "Overwrite"=TRUE ("항상 덮어쓰기")) -> ()  [unwired: 3 in, 8 out]
            n748 = invoke on="Water_Velocity_3_4" class="WFChart (엄격한)" method="Export Image"("FileType"=enum32{"BMP", "EPS", "EMF", "PICT"}."BMP" ("파일 타입"), "Target"=enum32{"File", "Clipboard"}."File" ("타겟"), "Path"=w1559, "HideGrid"=FALSE ("눈금 숨기기"), "Overwrite"=TRUE ("항상 덮어쓰기")) -> ()  [unwired: 3 in, 8 out]
            n749 = invoke on="Water_Velocity_3_5" class="WFChart (엄격한)" method="Export Image"("FileType"=enum32{"BMP", "EPS", "EMF", "PICT"}."BMP" ("파일 타입"), "Target"=enum32{"File", "Clipboard"}."File" ("타겟"), "Path"=w1550, "HideGrid"=FALSE ("눈금 숨기기"), "Overwrite"=TRUE ("항상 덮어쓰기")) -> ()  [unwired: 3 in, 8 out]
            n750 = invoke on="Averange_Soundspeed_2_3" class="WFChart (엄격한)" method="Export Image"("FileType"=enum32{"BMP", "EPS", "EMF", "PICT"}."BMP" ("파일 타입"), "Target"=enum32{"File", "Clipboard"}."File" ("타겟"), "Path"=w1496, "HideGrid"=FALSE ("눈금 숨기기"), "Overwrite"=TRUE ("항상 덮어쓰기")) -> ()  [unwired: 3 in, 8 out]
            n751 = invoke on="Averange_Soundspeed_3_4" class="WFChart (엄격한)" method="Export Image"("FileType"=enum32{"BMP", "EPS", "EMF", "PICT"}."BMP" ("파일 타입"), "Target"=enum32{"File", "Clipboard"}."File" ("타겟"), "Path"=w1470, "HideGrid"=FALSE ("눈금 숨기기"), "Overwrite"=TRUE ("항상 덮어쓰기")) -> ()  [unwired: 3 in, 8 out]
            n752 = Concatenate Strings("Water_Velocity_4_5_%Y_%m_%d" ("시간 포맷 문자열 (%c)"), ".png" ("시간 포맷 문자열 (%c)")) -> (w1543:string)
            n753 = Concatenate Strings("Averange_Soundspeed_1_2_%Y_%m_%d" ("시간 포맷 문자열 (%c)"), ".png" ("시간 포맷 문자열 (%c)")) -> (w1535:string)
            n754 = Concatenate Strings("Averange_Soundspeed_1_3_%Y_%m_%d" ("시간 포맷 문자열 (%c)"), ".png" ("시간 포맷 문자열 (%c)")) -> (w1525:string)
            n755 = Concatenate Strings("Averange_Soundspeed_1_4_%Y_%m_%d" ("시간 포맷 문자열 (%c)"), ".png" ("시간 포맷 문자열 (%c)")) -> (w1517:string)
            n756 = Concatenate Strings("Averange_Soundspeed_3_5_%Y_%m_%d" ("시간 포맷 문자열 (%c)"), ".png" ("시간 포맷 문자열 (%c)")) -> (w1464:string)
            n757 = Concatenate Strings("Averange_Soundspeed_2_4_%Y_%m_%d" ("시간 포맷 문자열 (%c)"), ".png" ("시간 포맷 문자열 (%c)")) -> (w1489:string)
            n758 = Format Date/Time String(time format string (%c)=w1543) -> (date/time string=w1542:string)  [unwired: 2 in]
            n759 = Format Date/Time String(time format string (%c)=w1535) -> (date/time string=w1536:string)  [unwired: 2 in]
            n760 = Format Date/Time String(time format string (%c)=w1525) -> (date/time string=w1524:string)  [unwired: 2 in]
            n761 = Format Date/Time String(time format string (%c)=w1517) -> (date/time string=w1518:string)  [unwired: 2 in]
            n762 = Format Date/Time String(time format string (%c)=w1464) -> (date/time string=w1465:string)  [unwired: 2 in]
            n763 = Format Date/Time String(time format string (%c)=w1489) -> (date/time string=w1488:string)  [unwired: 2 in]
            n764 = Build Path(base path=w1451, name or relative path=w1542) -> (appended path=w1541:path)
            n765 = Build Path(base path=w1451, name or relative path=w1536) -> (appended path=w1532:path)
            n766 = Build Path(base path=w1451, name or relative path=w1524) -> (appended path=w1523:path)
            n767 = Build Path(base path=w1451, name or relative path=w1518) -> (appended path=w1514:path)
            n768 = Build Path(base path=w1451, name or relative path=w1465) -> (appended path=w1461:path)
            n769 = Build Path(base path=w1451, name or relative path=w1488) -> (appended path=w1487:path)
            n770 = invoke on="Water_Velocity_4_5" class="WFChart (엄격한)" method="Export Image"("FileType"=enum32{"BMP", "EPS", "EMF", "PICT"}."BMP" ("파일 타입"), "Target"=enum32{"File", "Clipboard"}."File" ("타겟"), "Path"=w1541, "HideGrid"=FALSE ("눈금 숨기기"), "Overwrite"=TRUE ("항상 덮어쓰기")) -> ()  [unwired: 3 in, 8 out]
            n771 = invoke on="Averange_Soundspeed_1_2" class="WFChart (엄격한)" method="Export Image"("FileType"=enum32{"BMP", "EPS", "EMF", "PICT"}."BMP" ("파일 타입"), "Target"=enum32{"File", "Clipboard"}."File" ("타겟"), "Path"=w1532, "HideGrid"=FALSE ("눈금 숨기기"), "Overwrite"=TRUE ("항상 덮어쓰기")) -> ()  [unwired: 3 in, 8 out]
            n772 = invoke on="Averange_Soundspeed_1_3" class="WFChart (엄격한)" method="Export Image"("FileType"=enum32{"BMP", "EPS", "EMF", "PICT"}."BMP" ("파일 타입"), "Target"=enum32{"File", "Clipboard"}."File" ("타겟"), "Path"=w1523, "HideGrid"=FALSE ("눈금 숨기기"), "Overwrite"=TRUE ("항상 덮어쓰기")) -> ()  [unwired: 3 in, 8 out]
            n773 = invoke on="Averange_Soundspeed_1_4" class="WFChart (엄격한)" method="Export Image"("FileType"=enum32{"BMP", "EPS", "EMF", "PICT"}."BMP" ("파일 타입"), "Target"=enum32{"File", "Clipboard"}."File" ("타겟"), "Path"=w1514, "HideGrid"=FALSE ("눈금 숨기기"), "Overwrite"=TRUE ("항상 덮어쓰기")) -> ()  [unwired: 3 in, 8 out]
            n774 = invoke on="Averange_Soundspeed_2_4" class="WFChart (엄격한)" method="Export Image"("FileType"=enum32{"BMP", "EPS", "EMF", "PICT"}."BMP" ("파일 타입"), "Target"=enum32{"File", "Clipboard"}."File" ("타겟"), "Path"=w1487, "HideGrid"=FALSE ("눈금 숨기기"), "Overwrite"=TRUE ("항상 덮어쓰기")) -> ()  [unwired: 3 in, 8 out]
            n775 = invoke on="Averange_Soundspeed_3_5" class="WFChart (엄격한)" method="Export Image"("FileType"=enum32{"BMP", "EPS", "EMF", "PICT"}."BMP" ("파일 타입"), "Target"=enum32{"File", "Clipboard"}."File" ("타겟"), "Path"=w1461, "HideGrid"=FALSE ("눈금 숨기기"), "Overwrite"=TRUE ("항상 덮어쓰기")) -> ()  [unwired: 3 in, 8 out]
          }
          frame #2 {
            w1638 = waveform(dbl)[] [] ("히스토리 데이터")
            n776 = call "Save_teplete(Subvi).vi"("숫자형"=1) -> ()  [unwired: 11 in]
            n777 = property on="데이터 통계 현황_결과창" class="Str"("Value"="") -> ()  [unwired: 2 in, 2 out]
            n778 = property on="Water_Velocity_1_2" class="WFChart (엄격한)"("History Data"=w1638) -> ()  [unwired: 2 in, 2 out]
            n779 = property on="Water_Velocity_1_3" class="WFChart (엄격한)"("History Data"=w1638) -> ()  [unwired: 2 in, 2 out]
            n780 = property on="Water_Velocity_1_4" class="WFChart (엄격한)"("History Data"=w1638) -> ()  [unwired: 2 in, 2 out]
            n781 = property on="Water_Velocity_1_5" class="WFChart (엄격한)"("History Data"=w1638) -> ()  [unwired: 2 in, 2 out]
            n782 = property on="Water_Velocity_2_5" class="WFChart (엄격한)"("History Data"=w1638) -> ()  [unwired: 2 in, 2 out]
            n783 = property on="Water_Velocity_2_3" class="WFChart (엄격한)"("History Data"=w1638) -> ()  [unwired: 2 in, 2 out]
            n784 = property on="Water_Velocity_2_4" class="WFChart (엄격한)"("History Data"=w1638) -> ()  [unwired: 2 in, 2 out]
            n785 = property on="Water_Velocity_2_5" class="WFChart (엄격한)"("History Data"=w1638) -> ()  [unwired: 2 in, 2 out]
            n786 = property on="Water_Velocity_3_4" class="WFChart (엄격한)"("History Data"=w1638) -> ()  [unwired: 2 in, 2 out]
            n787 = property on="Water_Velocity_3_5" class="WFChart (엄격한)"("History Data"=w1638) -> ()  [unwired: 2 in, 2 out]
            n788 = property on="Water_Velocity_4_5" class="WFChart (엄격한)"("History Data"=w1638) -> ()  [unwired: 2 in, 2 out]
            n789 = property on="Averange_Soundspeed_1_2" class="WFChart (엄격한)"("History Data"=w1638) -> ()  [unwired: 2 in, 2 out]
            n790 = property on="Averange_Soundspeed_1_3" class="WFChart (엄격한)"("History Data"=w1638) -> ()  [unwired: 2 in, 2 out]
            n791 = property on="Averange_Soundspeed_1_4" class="WFChart (엄격한)"("History Data"=w1638) -> ()  [unwired: 2 in, 2 out]
            n792 = property on="Averange_Soundspeed_1_5" class="WFChart (엄격한)"("History Data"=w1638) -> ()  [unwired: 2 in, 2 out]
            n793 = property on="Averange_Soundspeed_2_3" class="WFChart (엄격한)"("History Data"=w1638) -> ()  [unwired: 2 in, 2 out]
            n794 = property on="Averange_Soundspeed_2_4" class="WFChart (엄격한)"("History Data"=w1638) -> ()  [unwired: 2 in, 2 out]
            n795 = property on="Averange_Soundspeed_2_5" class="WFChart (엄격한)"("History Data"=w1638) -> ()  [unwired: 2 in, 2 out]
            n796 = property on="Averange_Soundspeed_3_4" class="WFChart (엄격한)"("History Data"=w1638) -> ()  [unwired: 2 in, 2 out]
            n797 = property on="Averange_Soundspeed_3_5" class="WFChart (엄격한)"("History Data"=w1638) -> ()  [unwired: 2 in, 2 out]
            n798 = property on="Averange_Soundspeed_4_5" class="WFChart (엄격한)"("History Data"=w1638) -> ()  [unwired: 2 in, 2 out]
          }
        }
      }
      frame True {
      }
    }
    n799 = Wait (ms)(milliseconds to wait=u32 1000 ("대기 시간 (ms)")) -> ()  [unwired: 1 out]
    n800 = Unbundle By Name(w1431) -> ("Water_Velocity_1_3"=→"Water_Velocity_1_3":dbl, "Water_Velocity_1_2"=→"Water_Velocity_1_2":dbl, "Water_Velocity_1_4"=→"Water_Velocity_1_4":dbl, "Water_Velocity_1_5"=→"Water_Velocity_1_5":dbl, "Water_Velocity_2_3"=→"Water_Velocity_2_3":dbl, "Water_Velocity_2_4"=→"Water_Velocity_2_4":dbl, "Water_Velocity_2_5"=→"Water_Velocity_2_5":dbl, "Water_Velocity_3_4"=→"Water_Velocity_3_4":dbl, "Water_Velocity_3_5"=→"Water_Velocity_3_5":dbl, "Water_Velocity_4_5"=→"Water_Velocity_4_5":dbl, "Averange_Soundspeed_1_2"=→"Averange_Soundspeed_1_2":dbl, "Averange_Soundspeed_1_3"=→"Averange_Soundspeed_1_3":dbl, "Averange_Soundspeed_1_4"=→"Averange_Soundspeed_1_4":dbl, "Averange_Soundspeed_1_5"=→"Averange_Soundspeed_1_5":dbl, "Averange_Soundspeed_2_3"=→"Averange_Soundspeed_2_3":dbl, "Averange_Soundspeed_2_4"=→"Averange_Soundspeed_2_4":dbl, "Averange_Soundspeed_2_5"=→"Averange_Soundspeed_2_5":dbl, "Averange_Soundspeed_3_4"=→"Averange_Soundspeed_3_4":dbl, "Averange_Soundspeed_3_5"=→"Averange_Soundspeed_3_5":dbl, "Averange_Soundspeed_4_5"=→"Averange_Soundspeed_4_5":dbl)
  }
  n801 = while {
    tunnel: w29 -> [w1926]
    tunnel: w19 -> [w1925]
    tunnel: [errorcluster {"status"=FALSE, "code"=0, "source"=""} ("에러 상수")] -> w26
    tunnel: w7 -> [w1919]
    tunnel: w6 -> [w1918]
    shift-right: [w1916] -> _
    shift-left: T8 {"Python 경로"=path "", "Publish 모듈 경로"=path "", "지도 모듈 경로"=path "", "Subscribe 모듈 경로"=path ""} -> [w1917]
    stop <- w1922 stop-if-true
    # "Brain_Loop"
    n802 = Dequeue Element(queue=w1925, error in (no error)=w1926) -> (queue out=w1921:refnum<queue>, element=w1923:T9, error out=w1920:errorcluster)  [unwired: 1 in, 1 out]
    n803 = case shown="\"유속 데이터\"" w1923 {
      tunnel: [_ _ _ _ _ _ _ w2044] -> w1922
      tunnel: w1921 -> [_ _ _ _ _ _ _ _]
      tunnel: w1920 -> [_ _ _ _ _ _ _ _]
      tunnel: w1919 -> [w1948 _ _ _ _ _ _ w2047]
      tunnel: w1918 -> [w1947 _ _ _ _ _ _ w2046]
      tunnel: w1917 -> [w1939 w1950 w1965 w1978 w2036 w2038 w2041 w2043]
      tunnel: [w1938 w1950 w1965 w1978 w2036 w2038 w2041 w2043] -> w1916
      frame "초기화", Default {
        w1931 = string[][] [["TX", "", "", "", "", "", "", "", "", ""], ["", "TX", "", "", "", "", "", "", "", ""], ["", "", "TX", "", "", "", "", "", "", ""], ["", "", "", "TX", "", "", "", "", "", ""], ["", "", "", "", "TX", "", "", "", "", ""], ["", "", "", "", "", "TX", "", "", "", ""], ["", "", "", "", "", "", "TX", "", "", ""], ["", "", "", "", "", "", "", "TX", "", ""], ["", "", "", "", "", "", "", "", "TX", ""], ["", "", "", "", "", "", "", "", "", "TX"]] ("아이템 이름")
        w1933 = FALSE
        w1934 = cluster{dbl[], i32[]} {[], []} ("값(신호)")
        w1943 = string[] ["TMC_SET_1", "TMC_SET_2", "TMC_SET_3", "TMC_SET_4", "TMC_SET_5"]
        # "배터리 전원, 소모전류, 컨트롤 온도, 수온, 압력, Roll, Pitch"
        # "※ 1) GUI가 실행 될때는 (0,0)에서 실행된다. 2) 탭 컨트롤은 데이터 통계로 초기화 한다. 3) 웨이브폼 그래프 값 초기화 4) Station_현황_GPS, TRX_Controller의 리스트 초기화(Brain_LOOP)"
        n804 = property on="구획" class="Pane"("Origin"=T11 {"Horizontal"=0, "Vertical"=0} ("원점")) -> ()  [unwired: 2 in, 2 out]
        n805 = Format Date/Time String(time format string (%c)="%d" ("시간 포맷 문자열 (%c)")) -> (date/time string=→"현재 날짜":string)  [unwired: 2 in]
        n806 = Enqueue Element(queue=w1948, element=Brain_Loop_CTL."Mqtt_Subscribe", error in (no error)=w1947) -> ()  [unwired: 1 in, 3 out]
        n807 = Bundle By Name(cluster=w1939, "Python 경로"="Python 경로", "Publish 모듈 경로"="Publish_모듈 경로", "지도 모듈 경로"="지도 모듈 경로", "Subscribe 모듈 경로"="Subscribe_모듈 경로") -> (w1938:T8)
        n808 = property on="전체메뉴_탭_컨트롤" class="TabCtl (엄격한)"("Value"=enum32{"지도", "데이터 통계", "관리자", "유속 데이터"}."데이터 통계" ("전체메뉴_탭_컨트롤")) -> ()  [unwired: 2 in, 2 out]
        n809 = call "Save_teplete(Subvi).vi"("숫자형"=1) -> ()  [unwired: 11 in]
        n810 = property on="데이터 통계 현황_결과창" class="Str"("Value"="") -> ()  [unwired: 2 in, 2 out]
        n811 = property on="Station_현황_TRX_Controller" class="MCListbox (엄격한)"("ColHdrString"=w1943, "ItemNames"=string[][] [["", "", "", "", "", "", ""], ["", "", "", "", "", "", ""], ["", "", "", "", "", "", ""], ["", "", "", "", "", "", ""], ["", "", "", "", "", "", ""], ["", "", "", "", "", "", ""], ["", "", "", "", "", "", ""], ["", "", "", "", "", "0", ""], ["", "", "", "", "", "", ""], ["", "", "", "", "", "", ""], ["", "", "", "", "", "", ""], ["", "", "", "", "", "", ""], ["", "", "", "", "", "", ""], ["", "", "", "", "", "", ""]], "RowHdrs[]"=string[] ["배터리 전원", "소모전류", "수온", "압력", "ROLL", "PITCH", "컨트롤 온도", "", ""]) -> ()  [unwired: 2 in, 2 out]
        n812 = property on="Station_현황_GPS" class="MCListbox (엄격한)"("ColHdrString"=w1943, "ItemNames"=string[][] [["", "", "", "", "", ""], ["", "", "", "", "", ""], ["", "", "", "", "", ""], ["", "", "", "", "", ""], ["", "", "", "", "", ""], ["", "", "", "", "", ""], ["", "", "", "", "", ""], ["", "", "", "", "", "0"]], "RowHdrs[]"=string[] ["1PPS", "Latitude", "Longitude"]) -> ()  [unwired: 2 in, 2 out]
        n813 = property on="유속 데이터 흐름표_10분" class="MCListbox (엄격한)"("ItemNames"=w1931) -> ()  [unwired: 2 in, 2 out]
        n814 = property on="유속 데이터 흐름표_30분" class="MCListbox (엄격한)"("ItemNames"=w1931) -> ()  [unwired: 2 in, 2 out]
        n815 = property on="유속 데이터 흐름표_50분" class="MCListbox (엄격한)"("ItemNames"=w1931) -> ()  [unwired: 2 in, 2 out]
        n816 = local write "TX_LED_5"(w1933) -> ()
        n817 = local write "TX_LED_4"(w1933) -> ()
        n818 = local write "TX_LED_3"(w1933) -> ()
        n819 = local write "TX_LED_1"(w1933) -> ()
        n820 = local write "TX_LED_2"(w1933) -> ()
        n821 = local write "RX_LED_5"(w1933) -> ()
        n822 = local write "RX_LED_4"(w1933) -> ()
        n823 = local write "RX_LED_3"(w1933) -> ()
        n824 = local write "RX_LED_2"(w1933) -> ()
        n825 = local write "RX_LED_1"(w1933) -> ()
        n826 = property on="Station_1" class="XYGraph (엄격한)"("Val(Sgnl)"=w1934) -> ()  [unwired: 2 in, 2 out]
        n827 = property on="Station_2" class="XYGraph (엄격한)"("Val(Sgnl)"=w1934) -> ()  [unwired: 2 in, 2 out]
        n828 = property on="Station_3" class="XYGraph (엄격한)"("Val(Sgnl)"=w1934) -> ()  [unwired: 2 in, 2 out]
        n829 = property on="Station_4" class="XYGraph (엄격한)"("Val(Sgnl)"=w1934) -> ()  [unwired: 2 in, 2 out]
        n830 = property on="Station_5" class="XYGraph (엄격한)"("Val(Sgnl)"=w1934) -> ()  [unwired: 2 in, 2 out]
      }
      frame "Mqtt_Publish" {
        # "※ 적용 버튼을 클릭시 Brain_Loop에서 Mqtt_Publish Python 모듈 실행(Brain_LOOP)['Stop,Order,Q,'Start']"
        n831 = Unbundle By Name(w1950) -> ("Python 경로"=w1952:path, "Publish 모듈 경로"=w1951:path)
        n832 = Open Python Session(python version="3.9" ("Python 버전"), python path=w1952) -> (session out=w1961:refnum<k35>, error out=w1957:errorcluster)  [unwired: 1 in]
        n833 = node(w1961, w1951, "Mqtt_Publish" ("함수 이름"), w1957, " ", "Order", "Q 값") -> (w1959:refnum<k35>, w1960:errorcluster)  [unwired: 3 in, 2 out]
        n834 = Close Python Session(session in=w1959, error in=w1960) -> ()  [unwired: 1 out]
        n835 = flat-sequence {
          frame #0 {
            n836 = property on="적용_LED" class="Bool (엄격한)"("Blinking"=TRUE ("점멸")) -> ()  [unwired: 2 in, 2 out]
            n837 = Wait (ms)(milliseconds to wait=u32 2000 ("대기 시간 (ms)")) -> ()  [unwired: 1 out]
          }
          frame #1 {
            n838 = property on="적용_LED" class="Bool (엄격한)"("Blinking"=FALSE ("점멸")) -> ()  [unwired: 2 in, 2 out]
          }
        }
      }
      frame "Mqtt_Publish_2" {
        # "※ 적용 버튼을 클릭시 Brain_Loop에서 Mqtt_Publish Python 모듈 실행(Brain_LOOP)['Stop,Order,Q,'Start']"
        n839 = Unbundle By Name(w1965) -> ("Python 경로"=w1967:path, "Publish 모듈 경로"=w1966:path)
        n840 = Open Python Session(python version="3.9" ("Python 버전"), python path=w1967) -> (session out=w1974:refnum<k35>, error out=w1970:errorcluster)  [unwired: 1 in]
        n841 = node(w1974, w1966, "Mqtt_Publish_2" ("함수 이름"), w1970, " ") -> (w1972:refnum<k35>, w1973:errorcluster)  [unwired: 1 in, 2 out]
        n842 = Close Python Session(session in=w1972, error in=w1973) -> ()  [unwired: 1 out]
        n843 = flat-sequence {
          frame #0 {
            n844 = property on="적용_LED 2" class="Bool (엄격한)"("Blinking"=TRUE ("점멸")) -> ()  [unwired: 2 in, 2 out]
            n845 = Wait (ms)(milliseconds to wait=u32 2000 ("대기 시간 (ms)")) -> ()  [unwired: 1 out]
          }
          frame #1 {
            n846 = property on="적용_LED 2" class="Bool (엄격한)"("Blinking"=FALSE ("점멸")) -> ()  [unwired: 2 in, 2 out]
          }
        }
      }
      frame "지도" {
        # "※ 리스트에 표시된 데이터를 이용하여 Python 모듈과 연동하여 지도 모듈 구현(Brain_LOOP)"
        n847 = property on="Station_현황_GPS" class="MCListbox (엄격한)"() -> ("ItemNames"=w1990:string[][])  [unwired: 2 in, 2 out]
        n848 = Delete From Array(array=w1990, index (row)=2 ("인덱스 (행)")) -> (deleted portion=w1991:string[])  [unwired: 2 in, 1 out]
        n849 = Delete From Array(array=w1990, index (row)=1 ("인덱스 (행)")) -> (deleted portion=w1992:string[])  [unwired: 2 in, 1 out]
        n850 = Unbundle By Name(w1978) -> ("Python 경로"=w1980:path, "지도 모듈 경로"=w1979:path)
        n851 = Build Array(w1992, w1991) -> (w1988:string[][])
        n852 = disable-structure shown="기본" {
          disable-tunnel: [w1995] -> w1981
          frame Enabled {
            w1996 = T10 1 items=["사용자 홈"=0, "사용자 데스크탑"=1, "사용자 문서"=2, "사용자 어플리케이션 데이터"=3, "사용자 환경"=4, "사용자 임시"=5, "퍼블릭 문서"=6, "퍼블릭 어플리케이션 데이터"=7, "퍼블릭 환경"=8, "퍼블릭 캐시"=13, "시스템 코어 라이브러리"=9, "시스템 설치된 라이브러리"=10, "어플리케이션 파일"=11, "부팅 볼륨 루트"=12] ("system directory type")
            # "※ Python 모듈에서 .html 파일의 저장 위치는 데이터 저장 폴더위치와 동일하게 설정한다\n    만약 해당 폴더가 없을 경우 폴더를 생성하여 해당 폴더에 저장한다."
            n853 = call <vilib>:"Get System Directory.vi"("system directory type"=w1996) -> ("system directory"=w1998:path)  [unwired: 10 in]
            n854 = Build Path(base path=w1998, name or relative path="CSV_DATA") -> (appended path=w2002:path)
            n855 = call <vilib>:"Check if File or Folder Exists.vi"("path"=w2002) -> ("error out"=w2001:errorcluster, "file or folder exists?"=w1999:bool, "dup path"=w2000:path)  [unwired: 8 in]
            n856 = case shown="거짓" w1999 {
              tunnel: w2000 -> [w2007 w2009]
              tunnel: w2001 -> [w2006 w2008]
              tunnel: [w2005 w2009] -> w2003
              tunnel: [w2004 w2008] -> _
              frame False {
                n857 = Create Folder(path (use dialog)=w2007, error in=w2006) -> (created path=w2005:path, error out=w2004:errorcluster)  [unwired: 1 in, 1 out]
              }
              frame True {
              }
            }
            n858 = Path To String(path=w2003) -> (string=w1995:string)
          }
        }
        n859 = Delete From Array(array=w1988, index (col)=5 ("비활성화된 인덱스 (열)")) -> (array with subset deleted=w1987:string[][])  [unwired: 2 in, 1 out]
        n860 = Fract/Exp String To Number(string=w1987) -> (number=w1983:dbl[][])  [unwired: 3 in, 1 out]
        n861 = disable-structure shown="기본" {
          disable-tunnel: [w2012] -> w1986
          disable-tunnel: w1983 -> [w2010]
          frame Enabled {
            # "※ 지도 모듈 버튼 작동시 GPS 데이터가 최소 2개이상 들어와야 Python 모듈이 작동된다. 5개의 데이터 중 2개 이상 들어온다면 인덱스 값: 3 \n 에러없이 작동됨에 따라 2개이상 데이터가 없다면 LED 블랭크 작동"
            n862 = for {
              tunnel: w2010 -> [w2016] mode=indexing
              tunnel: [w2014] -> w2012
              tunnel: 0 -> [w2013]
              n863 = Equal To 0?(x=w2016) -> (x = 0?=w2015:bool[])
              n864 = for {
                tunnel: w2015 -> [w2019] mode=indexing
                shift-right: [w2017] -> w2014
                shift-left: w2013 -> [w2018]
                n865 = case shown="참" w2019 {
                  tunnel: w2018 -> [w2020 w2022]
                  tunnel: [w2020 w2021] -> w2017
                  frame False {
                  }
                  frame True {
                    n866 = Increment(x=w2022) -> (x+1=w2021:i32)
                  }
                }
              }
            }
          }
        }
        n867 = call "Reshape_Array_GPS(Subvi).vi"("2차원_GPS_Data"=w1983) -> ("1차원_GPS_Data"=w1982:dbl[])  [unwired: 10 in]
        n868 = Less Or Equal?(x=w1986, y=3) -> (x <= y?=w1984:bool)
        n869 = case shown="참" w1984 {
          tunnel: w1982 -> [_ w2027]
          tunnel: w1981 -> [_ w2026]
          tunnel: w1980 -> [_ w2025]
          tunnel: w1979 -> [_ w2024]
          frame False {
            # "※ 2개이상 없다면 LED 블랭크"
            n870 = property on="지도모듈_LED" class="Bool (엄격한)"("Blinking"=TRUE ("점멸")) -> ()  [unwired: 2 in, 2 out]
          }
          frame True {
            # "※ GPS 데이터가 2개 이상 들어온다면 Python 모듈 실행, 2개이상 있다면 LED 블랭크 F"
            n871 = Open Python Session(python version="3.9" ("Python 버전"), python path=w2025) -> (session out=w2030:refnum<k35>, error out=w2034:errorcluster)  [unwired: 1 in]
            n872 = node(w2030, w2024, "Map" ("함수 이름"), w2034, dbl[] [0.0], w2026, w2027) -> (w2032:refnum<k35>, w2031:errorcluster)  [unwired: 3 in, 2 out]
            n873 = property on="지도모듈_LED" class="Bool (엄격한)"("Blinking"=FALSE ("점멸")) -> ()  [unwired: 2 in, 2 out]
            n874 = Close Python Session(session in=w2032, error in=w2031) -> ()  [unwired: 1 out]
          }
        }
      }
      frame "관리자" {
        # "※ 관리자 버튼 클릭시 탭 컨트롤을 관리자로 변경(Brain_LOOP)"
        n875 = property on="전체메뉴_탭_컨트롤" class="TabCtl (엄격한)"("Value"=enum32{"지도", "데이터 통계", "관리자", "유속 데이터"}."관리자" ("전체메뉴_탭_컨트롤")) -> ()  [unwired: 2 in, 2 out]
      }
      frame "데이터통계" {
        # "※ 데이터통계 버튼 클릭시 탭 컨트롤을 데이터 통계로 변경(Brain_LOOP)"
        n876 = property on="전체메뉴_탭_컨트롤" class="TabCtl (엄격한)"("Value"=enum32{"지도", "데이터 통계", "관리자", "유속 데이터"}."데이터 통계" ("전체메뉴_탭_컨트롤")) -> ()  [unwired: 2 in, 2 out]
      }
      frame "유속 데이터" {
        # "※ 알림 버튼 클릭시 탭 컨트롤을 알림으로 변경(Brain_LOOP)"
        n877 = property on="전체메뉴_탭_컨트롤" class="TabCtl (엄격한)"("Value"=enum32{"지도", "데이터 통계", "관리자", "유속 데이터"}."유속 데이터" ("전체메뉴_탭_컨트롤")) -> ()  [unwired: 2 in, 2 out]
        n878 = property on="구획" class="Pane"("Origin"=T11 {"Horizontal"=24, "Vertical"=941} ("원점")) -> ()  [unwired: 2 in, 2 out]
      }
      frame "정지" {
        w2044 = TRUE
        # "※ 정지 버튼 클릭시 탭 컨트롤을 관리자로 변경(Brain_LOOP), 정지 버튼 클릭시 GUI 종료"
        n879 = Enqueue Element(queue=w2047, element=Brain_Loop_CTL."정지", error in (no error)=w2046) -> ()  [unwired: 1 in, 3 out]
        n880 = Quit LabVIEW(quit? (T)=w2044) -> ()
      }
    }
  }
  n881 = Merge Errors(w27, w26, w16, w15) -> (w13:errorcluster)
  n882 = while {
    tunnel: w7 -> [w2061]
    tunnel: w6 -> [w2060]
    tunnel: w21 -> [w2058]
    tunnel: w20 -> [w2057]
    shift-right: [w2050] -> _
    shift-left: string[][] [["", "", "", "", "", ""], ["", "", "", "", "", ""], ["", "", "", "", "", ""], ["", "", "", "", "", "0"], ["", "", "", "", "", ""], ["", "", "", "", "", ""], ["", "", "", "", "", ""], ["", "", "", "", "", "0"], ["", "", "", "", "", ""], ["", "", "", "", "", ""], ["", "", "", "", "", ""], ["", "", "", "", "", ""], ["", "", "", "", "", ""]] -> [w2052]
    tunnel: [errorcluster {"status"=FALSE, "code"=0, "source"=""} ("에러 상수")] -> w14
    stop <- w2059 stop-if-true
    # "Number 데이터 분리 후 리스트 박스 열에 데이터 대체"
    # "3 index: Number"
    n883 = Dequeue Element(queue=w2061, error in (no error)=w2060) -> (queue out=w2056:refnum<queue>, element=w2049:T9, error out=w2055:errorcluster)  [unwired: 1 in, 1 out]
    n884 = Dequeue Element(queue=w2058, error in (no error)=w2057) -> (element=w2051:string[])  [unwired: 1 in, 3 out]
    n885 = case shown="\"정지\"" w2049 {
      tunnel: [_ _ TRUE] -> w2059
      tunnel: w2056 -> [_ w2099 w2104]
      tunnel: w2055 -> [_ w2098 w2103]
      frame "초기화", Default {
      }
      frame "Mqtt_Subscribe" {
        n886 = Enqueue Element(queue=w2099, element=Brain_Loop_CTL."Mqtt_Subscribe", error in (no error)=w2098) -> ()  [unwired: 1 in, 3 out]
      }
      frame "정지" {
        n887 = Flush Queue(queue=w2104, error in (no error)=w2103) -> (queue out=w2101:refnum<queue>, error out=w2102:errorcluster)  [unwired: 1 out]
        n888 = Enqueue Element(queue=w2101, element=Brain_Loop_CTL."정지", error in (no error)=w2102) -> ()  [unwired: 1 in, 3 out]
      }
    }
    n889 = Index Array(array=w2051, index=3 ("인덱스")) -> (element=w2053:string)
    n890 = case shown="\"3\"" w2053 {
      tunnel: w2051 -> [_ w2067 w2074 w2081 w2088 w2095]
      tunnel: w2052 -> [w2062 w2069 w2076 w2083 w2090 w2097]
      tunnel: [w2062 w2063 w2070 w2077 w2084 w2091] -> w2050
      frame "거짓", Default {
      }
      frame "1" {
        # "Number 데이터 분리 후 리스트 박스 열에 데이처 대체"
        n891 = Array Subset(array=w2067, index=0 ("차원 크기"), length=3 ("차원 크기")) -> (w2064:string[])
        n892 = Replace Array Subset(array=w2069, new element=w2064, index (col)=0 ("비활성화된 인덱스 (열)")) -> (w2063:string[][])  [unwired: 1 in]
        n893 = property on="Station_현황_GPS" class="MCListbox (엄격한)"("ItemNames"=w2063) -> ()  [unwired: 2 in, 2 out]
      }
      frame "2" {
        # "Number 데이터 분리 후 리스트 박스 열에 데이처 대체"
        n894 = Array Subset(array=w2074, index=0 ("차원 크기"), length=3 ("차원 크기")) -> (w2071:string[])
        n895 = Replace Array Subset(array=w2076, new element=w2071, index (col)=1 ("비활성화된 인덱스 (열)")) -> (w2070:string[][])  [unwired: 1 in]
        n896 = property on="Station_현황_GPS" class="MCListbox (엄격한)"("ItemNames"=w2070) -> ()  [unwired: 2 in, 2 out]
      }
      frame "3" {
        # "Number 데이터 분리 후 리스트 박스 열에 데이처 대체"
        n897 = Array Subset(array=w2081, index=0 ("차원 크기"), length=3 ("차원 크기")) -> (w2078:string[])
        n898 = Replace Array Subset(array=w2083, new element=w2078, index (col)=2 ("비활성화된 인덱스 (열)")) -> (w2077:string[][])  [unwired: 1 in]
        n899 = property on="Station_현황_GPS" class="MCListbox (엄격한)"("ItemNames"=w2077) -> ()  [unwired: 2 in, 2 out]
      }
      frame "4" {
        # "Number 데이터 분리 후 리스트 박스 열에 데이처 대체"
        n900 = Array Subset(array=w2088, index=0 ("차원 크기"), length=3 ("차원 크기")) -> (w2085:string[])
        n901 = Replace Array Subset(array=w2090, new element=w2085, index (col)=3 ("비활성화된 인덱스 (열)")) -> (w2084:string[][])  [unwired: 1 in]
        n902 = property on="Station_현황_GPS" class="MCListbox (엄격한)"("ItemNames"=w2084) -> ()  [unwired: 2 in, 2 out]
      }
      frame "5" {
        # "Number 데이터 분리 후 리스트 박스 열에 데이처 대체"
        n903 = Array Subset(array=w2095, index=0 ("차원 크기"), length=3 ("차원 크기")) -> (w2092:string[])
        n904 = Replace Array Subset(array=w2097, new element=w2092, index (col)=4 ("비활성화된 인덱스 (열)")) -> (w2091:string[][])  [unwired: 1 in]
        n905 = property on="Station_현황_GPS" class="MCListbox (엄격한)"("ItemNames"=w2091) -> ()  [unwired: 2 in, 2 out]
      }
    }
  }
  n906 = disable-structure shown="비활성화" {
    frame Disabled {
      (unwired) dbl[] [37.5072384, 127.0238756, 37.4172384, 127.1338756, 37.5442384, 127.0448756, 37.4032384, 127.4638756, 37.8055384, 127.7643756]
    }
    frame Enabled {
    }
  }
  n907 = Merge Errors(w13, w14, w4, w3) -> (w2:errorcluster)
  n908 = call <vilib>:"Clear Errors.vi"("error in (no error)"=w2, "specific error code to clear (0: all)"=0) -> ()  [unwired: 4 in, 2 out]
